vi "Beampointing_ajgEditObsolete.vi"() -> ()   [LabVIEW 2020]
uses:
  Shared/GUI_Template/GUI_master/tcp new data cluster.ctl
  <userlib>/_OpenG.lib/array/array.llb/Filter 1D Array with Scalar (String)__ogtk.vi
  <vilib>/Analysis/NI_AALBase.lvlib
  GUI_Beampointing_single_TRA/Ctrs/move.ctl
  Ctrs/beam detection.ctl
  <vilib>/vision/NI_Vision_Development_Module.lvlib
  General GUIs/Device GUIs/GUI_Cameras/Controls/Crosshair type def.ctl
  Ctrs/BP configuration.ctl
  <userlib>/_OpenG.lib/array/array.llb/Remove Duplicates from 1D Array (String)__ogtk.vi
  <vilib>/Utility/file.llb/Write To Spreadsheet File (string).vi
  <userlib>/_OpenG.lib/file/file.llb/Strip Path Extension - String__ogtk.vi
  <userlib>/_OpenG.lib/file/file.llb/File Exists - Scalar__ogtk.vi
  Shared/GUI_Template/GUI_master/tcp_new_data_event.ctl
panel:
  in  "active CCDs":i32(listbox)
  out "Prev State":string
  out "tcp data event 2":T1
  out "error out 3":errorcluster
  out "cam means":sgl[](array[numeric])
  in  "save path":path=path "W:/BP_DATA"
  out "particles":T2(array[cluster])
  out "millisecond timer value":u32
  out "motor refs 3":refnum<vi>[](array[refnum])
  in  "active man refs":cluster{"Ref X":refnum<vi>, "Ref Y":refnum<vi>}
  in  "#imgs avd so far":dbl
  out "Current State":string
  out "CCDs":string[](array[string])
  in  "GUIdevice 12":string
  in  "GUIdevice 11":string
  in  "GUIdevice 10":string
  in  "GUIdevice 9":string
  out "error out 2":errorcluster
  out "Names":string[](array[string])
  out "Box":T3(array[cluster])
  in  "Tab Cams":enum32{"Config ", "Main", "History", "Other"}(tab)=enum."Main"
  in  "Cameras and motors":T4(array[cluster]) {"Motor Alias Y" items=["M2 Y Axis", "M2 X Axis", "M4 Y Axis", "M4 X Axis", "M5 X Axis", "M5 Y Axis", "M1 Y Axis (mm)", "M1 X Axis (mm)", "Compression", "Grating 2&3", "Grating 1&4", "Clocking", "MIX", "F3M2 Horizontal", "F3M2 Vertical", "F3M3 Vertical", "F3M3 Horizontal", "F3M6 Horizontal", "F3M5 Horizontal", "F3M6 Vertical", "F3M5 Vertical", "HeatM5-X", "HeatM5-Y", "HeatM5-XY", "PlamsaLensHexapod", "HPD2 stage position", "HPD stage position", "M1-HPD X position", "M1-HPD Y position", "M2-HPD X position", "M2-HPD Y position", "HPDccd2 Stage position", "TargetX", "TargetY", "TargetZ", "IP", "PM4-X", "PM4-Y", "SDI_1x", "SDI_1y", "SDI_2x", "SDI_2y", "Comp-2BL-separation [mm]", "Comp-2BL-G1G4-angle [degree]", "Comp-2BL-G2G3-angle [degree]", "Comp-2BL-delay [mm]"]; "Motor Alias X" items=["M2 Y Axis", "M2 X Axis", "M4 Y Axis", "M4 X Axis", "M5 X Axis", "M5 Y Axis", "M1 Y Axis (mm)", "M1 X Axis (mm)", "Compression", "Grating 2&3", "Grating 1&4", "Clocking", "MIX", "F3M2 Horizontal", "F3M2 Vertical", "F3M3 Vertical", "F3M3 Horizontal", "F3M6 Horizontal", "F3M5 Horizontal", "F3M6 Vertical", "F3M5 Vertical", "HeatM5-X", "HeatM5-Y", "HeatM5-XY", "PlamsaLensHexapod", "HPD2 stage position", "HPD stage position", "M1-HPD X position", "M1-HPD Y position", "M2-HPD X position", "M2-HPD Y position", "HPDccd2 Stage position", "TargetX", "TargetY", "TargetZ", "IP", "PM4-X", "PM4-Y", "SDI_1x", "SDI_1y", "SDI_2x", "SDI_2y", "Comp-2BL-separation [mm]", "Comp-2BL-G1G4-angle [degree]", "Comp-2BL-G2G3-angle [degree]", "Comp-2BL-delay [mm]"]}
  out "Status":cluster{i32, i32, "Centroid X":dbl[][]}(graph)
  in  "tdms root":path=path "c:/BP_DATAsd"
  out "get pos time":u32
  out "config path":string
  in  "Exposure:12":dbl=0.095 min=0.0001 max=1.0 format="%#_6f"
  in  "Triggerdelay::12":dbl=0.003 min=0.0 max=0.09 format="%#_6f"
  in  "Exposure::11":dbl=0.095 min=0.0001 max=1.0 format="%#_6f"
  in  "Triggerdelay::11":dbl=0.003 min=0.0 max=0.09 format="%#_6f"
  in  "Exposure::10":dbl=0.095 min=0.0001 max=1.0 format="%#_6f"
  in  "Triggerdelay::10":dbl=0.003 min=0.0 max=0.09 format="%#_6f"
  in  "Exposure::9":dbl=0.095 min=0.0001 max=1.0 format="%#_6f"
  in  "Triggerdelay::9":dbl=0.003 min=0.0 max=0.09 format="%#_6f"
  in  "Trigger::9":bool
  in  "Trigger::10":bool caption="Trigger:10"
  in  "Trigger::11":bool
  in  "Trigger::12":bool
  in  "Target.Y::9":dbl=45.0 caption="T9y" min=0.0 max=2000.0 format="%#_6f"
  in  "Target.X::9":dbl=47.0 caption="Tx9" min=0.0 max=2000.0 format="%#_6f"
  in  "Target.Y::10":dbl=45.0 caption="T10y" min=0.0 max=2000.0 format="%#_6f"
  in  "Target.X::10":dbl=47.0 caption="T10x" min=0.0 max=2000.0 format="%#_6f"
  in  "Target.Y::11":dbl=45.0 caption="T11y" min=0.0 max=2000.0 format="%#_6f"
  in  "Target.X::11":dbl=47.0 caption="T11x" min=0.0 max=2000.0 format="%#_6f"
  in  "Target.Y::12":dbl=45.0 caption="T12y" min=0.0 max=2000.0 format="%#_6f"
  in  "Target.X::12":dbl=47.0 caption="T12x" min=0.0 max=2000.0 format="%#_6f"
  in  "Exposure::8":dbl=0.095 min=0.0001 max=1.0 format="%#_6f"
  in  "Triggerdelay::8":dbl=0.003 min=0.0 max=0.09 format="%#_6f"
  in  "Trigger::8":bool
  in  "Target.Y::8":dbl=45.0 caption="T8y" min=0.0 max=2000.0 format="%#_6f"
  in  "Target.X::8":dbl=47.0 caption="T8x" min=0.0 max=2000.0 format="%#_6f"
  in  "Target.Y::7":dbl=45.0 caption="T7x" min=0.0 max=2000.0 format="%#_6f"
  in  "Target.X::7":dbl=47.0 caption="T7y" min=0.0 max=2000.0 format="%#_6f"
  in  "Target.Y::6":dbl=45.0 caption="T6y" min=0.0 max=2000.0 format="%#_6f"
  in  "Target.X::6":dbl=47.0 caption="T6x" min=0.0 max=2000.0 format="%#_6f"
  in  "Target.Y::5":dbl=45.0 caption="T5y" min=0.0 max=2000.0 format="%#_6f"
  in  "Target.X::5":dbl=47.0 caption="T5x" min=0.0 max=2000.0 format="%#_6f"
  in  "Target.Y::4":dbl=45.0 caption="T4y" min=0.0 max=2000.0 format="%#_6f"
  in  "Target.X::4":dbl=47.0 caption="T4x" min=0.0 max=2000.0 format="%#_6f"
  in  "Target.Y::3":dbl=163.0 caption="T3y" min=0.0 max=2000.0 format="%#_6f"
  in  "Target.X::3":dbl=152.0 caption="T3x" min=0.0 max=2000.0 format="%#_6f"
  in  "Target.Y::2":dbl=74.0 caption="T2y" min=0.0 max=2000.0 format="%#_6f"
  in  "Target.X::2":dbl=75.0 caption="T2x" min=0.0 max=2000.0 format="%#_6f"
  in  "Target.Y::1":dbl=61.0 caption="T1y" min=0.0 max=2000.0 format="%#_6f"
  in  "Target.X::1":dbl=77.0 caption="T1x" min=0.0 max=2000.0 format="%#_6f"
  in  "Exposure::7":dbl=0.095 min=3.8e-05 max=1.0 format="%#_6f"
  in  "Triggerdelay::7":dbl=0.003 min=0.0 max=0.09 format="%#_6f"
  in  "Trigger::7":bool
  in  "Exposure::6":dbl=0.095 min=3.8e-05 max=1.0 format="%#_6f"
  in  "Triggerdelay::6":dbl=0.003 min=0.0 max=0.09 format="%#_6f"
  in  "Trigger::6":bool
  in  "Exposure::5":dbl=0.095 min=3.8e-05 max=1.0 format="%#_6f"
  in  "Triggerdelay::5":dbl=0.003 min=0.0 max=0.09 format="%#_6f"
  in  "Trigger::5":bool
  in  "Exposure::4":dbl=0.095 min=3.8e-05 max=1.0 format="%#_6f"
  in  "Triggerdelay::4":dbl=0.003 min=0.0 max=0.09 format="%#_6f"
  in  "Trigger::4":bool
  in  "Exposure::3":dbl=0.095 min=3.8e-05 max=1.0 format="%#_6f"
  in  "Triggerdelay::3":dbl=0.003 min=0.0 max=0.09 format="%#_6f"
  in  "Trigger::3":bool
  in  "Exposure::2":dbl=0.095 min=3.8e-05 max=1.0 format="%#_6f"
  in  "Triggerdelay::2":dbl=0.003 min=0.0 max=0.09 format="%#_6f"
  in  "Trigger::2":bool
  out "image::1":T5(plugin-control) caption="CAM-2BL-GHOST"
  out "image::2":T5(plugin-control) caption="CAM-2BL-F3M7"
  out "image::3":T5(plugin-control)
  out "image::4":T5(plugin-control)
  out "image::5":T5(plugin-control)
  out "image::6":T5(plugin-control)
  out "image::7":T5(plugin-control)
  out "image::8":T5(plugin-control)
  in  "Exposure::1":dbl=0.095 min=3.8e-05 max=1.0 format="%#_6f"
  in  "Triggerdelay::1":dbl=0.003 min=0.0 max=0.09 format="%#_6f"
  in  "Trigger::1":bool
  in  "UDP error message":string
  out "required Y":bool[](array[boolean])
  out "required X":bool[](array[boolean])
  out "detected":bool[](array[boolean])
  out "name array":string[](array[string])
  out "image::9":T5(plugin-control)
  out "image::10":T5(plugin-control)
  out "image::11":T5(plugin-control)
  out "image::12":T5(plugin-control)
  out "speedmode X":bool[](array[boolean])
  out "speedmode Y":bool[](array[boolean])
  out "CCD 9":cluster{timestamp[], dbl[]}[](graph)
  out "CCD 10":cluster{timestamp[], dbl[]}[](graph)
  out "CCD 11":cluster{timestamp[], dbl[]}[](graph)
  out "CCD 12":cluster{timestamp[], dbl[]}[](graph)
  out "CCD 5":cluster{timestamp[], dbl[]}[](graph)
  out "CCD 6":cluster{timestamp[], dbl[]}[](graph)
  out "CCD 7":cluster{timestamp[], dbl[]}[](graph)
  out "CCD 8":cluster{timestamp[], dbl[]}[](graph)
  out "CCD 2":cluster{timestamp[], dbl[]}[](graph)
  out "CCD 1":cluster{timestamp[], dbl[]}[](graph)
  out "CCD 3":cluster{timestamp[], dbl[]}[](graph)
  out "CCD 4":cluster{timestamp[], dbl[]}[](graph)
  in  "History Size":i32=500
  out "History Index":i32
  out "Moving X":string
  out "Moving Y":string
  in  "Feedback Global":bool
  in  "GUIdevice 8":string
  in  "Tab Control":T6(tab)
  in  "alarms":bool
  in  "new tdms":bool
  in  "Save Stats":bool
  in  "Save Config":bool
  in  "Load Config":bool
  in  "update speed [ms]":i32=2000
  in  "img to avg":i32=6 min=3 max=200
  in  "Reset History":bool
  in  "autodetect":bool
  in  "Detection Rate":dbl=0.9 min=0.001 max=1.0
  in  "Center":bool
  in  "Align":bool
  in  "Speedmode":dbl=5.0 min=1.0 max=20.0
  in  "device ini":bool
  in  "average centroid":bool
  in  "beam detection para":T7={"Filter"=1, "Filter Para"={"X Size"=5, "Y Size"=5, "% Tolerance"=1}, "detection method"=4, "smal para"=[{"Measurement Parameter"=35, "Range Lower Value"=0.0, "Range Upper Value"=500.0, "Range"=FALSE, "Measurement Type"=FALSE}], "Remove small Objects"=TRUE, "Restrict to round Objects"=FALSE} {"smal para"."Measurement Parameter" items=["Center of Mass X", "Center of Mass Y", "First Pixel X", "First Pixel Y", "Bounding Rect Left", "Bounding Rect Top", "Bounding Rect Right", "Bounding Rect Bottom", "Max Feret Diameter Start X", "Max Feret Diameter Start Y", "Max Feret Diameter End X", "Max Feret Diameter End Y", "Max Horiz. Segment Length Left", "Max Horiz. Segment Length Right", "Max Horiz. Segment Length Row", "-", "Bounding Rect Width", "Bounding Rect Height", "Bounding Rect Diagonal", "Perimeter", "Convex Hull Perimeter", "Holes' Perimeter", "Max Feret Diameter", "Equivalent Ellipse Major Axis", "Equivalent Ellipse Minor Axis", "Equivalent Ellipse Minor Axis (Feret)", "Equivalent Rect Long Side", "Equivalent Rect Short Side", "Equivalent Rect Diagonal", "Equivalent Rect Short Side (Feret)", "Average Horiz. Segment Length", "Average Vert. Segment Length", "Hydraulic Radius", "Waddel Disk Diameter", "-", "Area", "Holes' Area", "Particle & Holes' Area", "Convex Hull Area", "Image Area", "-", "Number of Holes", "Number of Horiz. Segments", "Number of Vert. Segments", "-", "Orientation", "Max Feret Diameter Orientation", "-", "% Area/Image Area", "% Area/(Particle & Holes' Area)", "Ratio of Equivalent Ellipse Axes", "Ratio of Equivalent Rect Sides", "-", "Elongation Factor", "Compactness Factor", "Heywood Circularity Factor", "Type Factor", "-", "Sum X", "Sum Y", "Sum XX", "Sum XY", "Sum YY", "Sum XXX", "Sum XXY", "Sum XYY", "Sum YYY", "-", "Moment of Inertia XX", "Moment of Inertia XY", "Moment of Inertia YY", "Moment of Inertia XXX", "Moment of Inertia XXY", "Moment of Inertia XYY", "Moment of Inertia YYY", "Norm. Moment of Inertia XX", "Norm. Moment of Inertia XY", "Norm. Moment of Inertia YY", "Norm. Moment of Inertia XXX", "Norm. Moment of Inertia XXY", "Norm. Moment of Inertia XYY", "Norm. Moment of Inertia YYY", "Hu Moment 1", "Hu Moment 2", "Hu Moment 3", "Hu Moment 4", "Hu Moment 5", "Hu Moment 6", "Hu Moment 7"]; "smal para"."Range Lower Value" format="%.2f"; "smal para"."Range Upper Value" format="%.2f"; "detection method" items=["clustering", "entropy", "metric", "moments", "inter-class variance"]; "Filter" items=["No Filter", "Median Filter", "Low Pass Filter"]}
  in  "move config":T9={"Tolerance [%]"=0.1, "Stepsize"=0.0001, "Invert Axis"=TRUE, "Invert Direction X"=FALSE, "Invert Direction Y"=TRUE, "enable feedback"=FALSE, "Set Centriod Target"=FALSE}
  in  "Position 2":dbl=0.001 caption="Stepsize" min=0.0 max=999999.0 format="%_6f"
  in  "Position 1":dbl=0.001 caption="Stepsize" min=0.0 max=999999.0 format="%_6f"
  in  "Right":bool caption="RelativeMove.Axis 1.CCW::1"
  in  "Left":bool caption="RelativeMove.Axis 1.CW::1"
  in  "Down":bool caption="RelativeMove.Axis. 2.CCW::1"
  in  "Up":bool caption="RelativeMove.Axis 2.CW::1"
  in  "StepSize":dbl=1.0 caption="Stepsize" min=0.0 max=1.0 step=0.001 format="%#_6p"
  in  "Time":timestamp[][](array[timestamp])
  in  "Offset X":dbl[][](array[numeric])
  in  "Mean Centroid X":dbl[][](array[numeric])
  in  "GUIdevice 7":string
  in  "GUIdevice 6":string
  in  "GUIdevice 5":string
  in  "GUIdevice 4":string
  in  "GUIdevice 3":string="TargetCam10Hz_Diode"
  in  "GUIdevice 2":string="StagingM1Far"
  in  "insert tag":bool=TRUE
  in  "stop":bool
  in  "GUIdevice 1":string="StagingM1Near"
  out "error IO 2":errorcluster
  # "Motor axes must have aliases"
  # "max"
  # "invert axis no longer used"
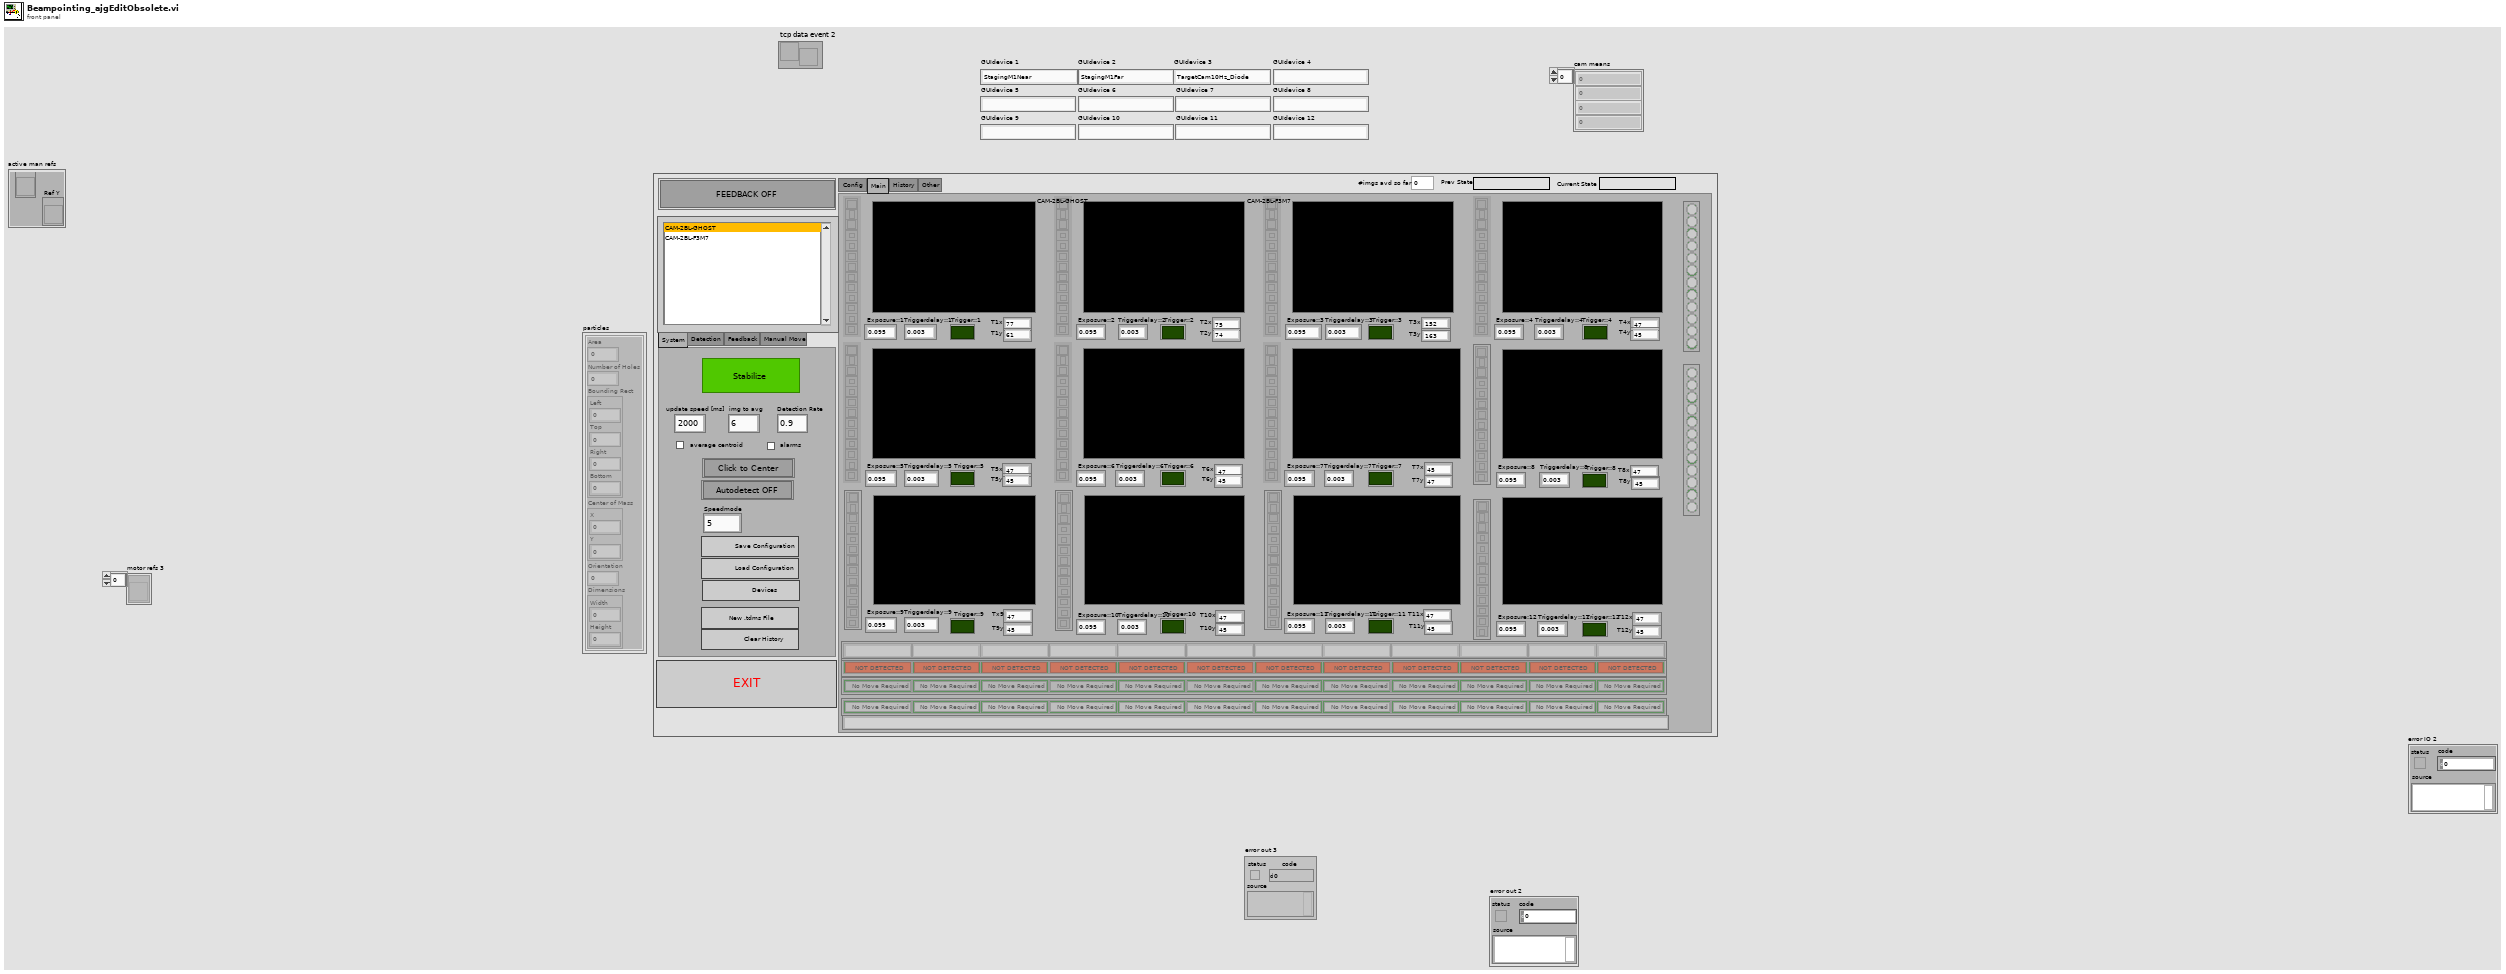
[diagram p1: front panel]
types:
  T1 = typedef "tcp_new_data_event.ctl" = refnum<user-event>
  T2 = cluster{"Area":dbl, "Number of Holes":dbl, "Bounding Rect":cluster{"Left":dbl, "Top":dbl, "Right":dbl, "Bottom":dbl}, "Center of Mass":cluster{"X":dbl, "Y":dbl}, "Orientation":dbl, "Dimensions":cluster{"Width":dbl, "Height":dbl}}[]
  T3 = cluster{"Left":dbl, "Top":dbl, "Right":dbl, "Bottom":dbl}[]
  T4 = cluster{"Camera":string, "Motor Alias X":u16, "Motor Alias Y":u16}[]
  T5 = typedef "IMAQ Image.ctl" = refnum<image>
  T6 = enum32{"System", "Detection", "Feedback", "Manual Move"}
  T7 = typedef "beam detection.ctl" = cluster{"Filter":u16, "Filter Para":cluster{"X Size":i32, "Y Size":i32, "% Tolerance":i32}, "detection method":i32, "smal para":cluster{"Measurement Parameter":T8, "Range Lower Value":dbl, "Range Upper Value":dbl, "Range":bool, "Measurement Type":bool}[], "Remove small Objects":bool, "Restrict to round Objects":bool}
  T8 = typedef "Particle Parameters" = i32
  T9 = typedef "move.ctl" = cluster{"Tolerance [%]":dbl, "Stepsize":dbl, "Invert Axis":bool, "Invert Direction X":bool, "Invert Direction Y":bool, "enable feedback":bool, "Set Centriod Target":bool}
  T10 = cluster{"Target.X::1":refnum<vi>, "Target.Y::1":refnum<vi>}
  T11 = cluster{"Target.X::2":refnum<vi>, "Target.Y::2":refnum<vi>}
  T12 = cluster{"Target.X::3":refnum<vi>, "Target.Y::3":refnum<vi>}
  T13 = cluster{"Target.X::4":refnum<vi>, "Target.Y::4":refnum<vi>}
  T14 = cluster{"Target.X::5":refnum<vi>, "Target.Y::5":refnum<vi>}
  T15 = cluster{"Target.X::6":refnum<vi>, "Target.Y::6":refnum<vi>}
  T16 = cluster{"Target.X::7":refnum<vi>, "Target.Y::7":refnum<vi>}
  T17 = cluster{"Target.X::8":refnum<vi>, "Target.Y::8":refnum<vi>}
  T18 = cluster{"Target.X::12":refnum<vi>, "Target.Y::12":refnum<vi>}
  T19 = cluster{"Target.X::9":refnum<vi>, "Target.Y::9":refnum<vi>}
  T20 = cluster{"Target.X::10":refnum<vi>, "Target.Y::10":refnum<vi>}
  T21 = cluster{"Target.X::11":refnum<vi>, "Target.Y::11":refnum<vi>}
  T22 = cluster{"Target.X::12":refnum<vi>, "Target.Y::12":refnum<vi>}[]
  T23 = enum32{"invalid app kind", "Development System", "Run Time System", "Student Edition", "Embedded LabVIEW", "Evaluation", "Custom"}
  T24 = enum32{"Invalid", "Standard", "Closed", "Hidden", "Minimized", "Maximized"}
  T25 = typedef "tcp new data cluster.ctl" = cluster{"EventEnum":enum16{"new data", "connection status update"}, "Device name":string}
  T26 = enum16{"open", "replace", "create", "open or create", "replace or create", "replace or create with confirmation"}
  T27 = enum8{"Enabled", "Disabled", "Disabled and Grayed Out"}
  T28 = enum16{"open", "open or create", "create or replace", "create", "open (read-only)"}
  T29 = cluster{"Left":dbl, "Top":dbl, "Right":dbl, "Bottom":dbl}
  T30 = typedef "move.ctl" = cluster{"Tolerance [pix]":dbl, "Stepsize":dbl, "Invert Direction X":bool, "Invert Direction Y":bool, "enable feedback":bool, "Set Centriod Target":bool}
  T31 = cluster{"Core":cluster{"Current VI Reference":refnum<vi>, "Close Panel on Exit?":bool}, "detection para":T7[], "thresholds":cluster{"Lower value":sgl, "Upper value":sgl}[], "Centroid X":dbl[][], "Centroid Y":dbl[][], "img to avg":i32, "Mean Centroid X":dbl[][], "Mean Centroid Y":dbl[][], "Offset X":dbl[][], "Offset Y":dbl[][], "Offset X stats ":dbl[][], "Offset Y stats ":dbl[][], "Size":dbl[][], "Mean Size":dbl[][], "Time":timestamp[][], "move properties":T30[], "active axis refs 2":cluster{"Ref X":refnum<vi>, "Ref Y":refnum<vi>}[], "active ccd":i32, "Feedback global":bool, "Motor X":dbl[][], "Motor Y":dbl[][], "active cams":string[], "tdms ref":refnum<k34>, "active man refs":cluster{"Ref X":refnum<vi>, "Ref Y":refnum<vi>}, "detected":bool[], "speedmode X":bool[], "speedmode Y":bool[], "steps speed X":dbl[], "steps speed Y":dbl[], "Supergui":cluster{"STOP queue":refnum<queue>, "SuperGUI ref":refnum<vi>}, "dev var alias arrays":cluster{"dev variable alias":string[][], "dev variable alias Motors X":string[][], "dev variable alias Motors Y":string[][]}, "Motor positions":cluster{"Positions x":dbl[], "Positions y":dbl[]}}
  T32 = cluster{"Positions x":dbl[], "Positions y":dbl[]}
  T33 = cluster{"dev variable alias":string[][], "dev variable alias Motors X":string[][], "dev variable alias Motors Y":string[][]}
  T34 = cluster{"Ref X":refnum<vi>, "Ref Y":refnum<vi>}[]
  T35 = cluster{"STOP queue":refnum<queue>, "SuperGUI ref":refnum<vi>}
  T36 = cluster{"Current VI Reference":refnum<vi>, "Close Panel on Exit?":bool}
  T37 = cluster{"Camera":string, "Motor Alias X":u16, "Motor Alias Y":u16}
  T38 = typedef "BP configuration.ctl" = cluster{"Camera names":string[], "Motor aliases x":string[], "Motor aliases y":string[], "detection para":T7[], "thresholds":cluster{"Lower value":sgl, "Upper value":sgl}[], "move properties":T30[]}
  T39 = typedef "Image Type" = u32
  T40 = cluster{"appended array":timestamp[], "appended array":dbl[]}
  T41 = cluster{"appended array":timestamp[], "appended array":dbl[]}[]
  T42 = typedef "Crosshair type def.ctl" = cluster{"Draw":bool, "Target":cluster{"x":dbl, "y":dbl}, "Size":cluster{"x":dbl, "y":dbl}, "Angle":dbl, "Color":u32, "Thickness":u8, "CrosshairLabel":string}
  T43 = cluster{"Left":i32, "Top":i32, "Right":i32, "Bottom":i32}
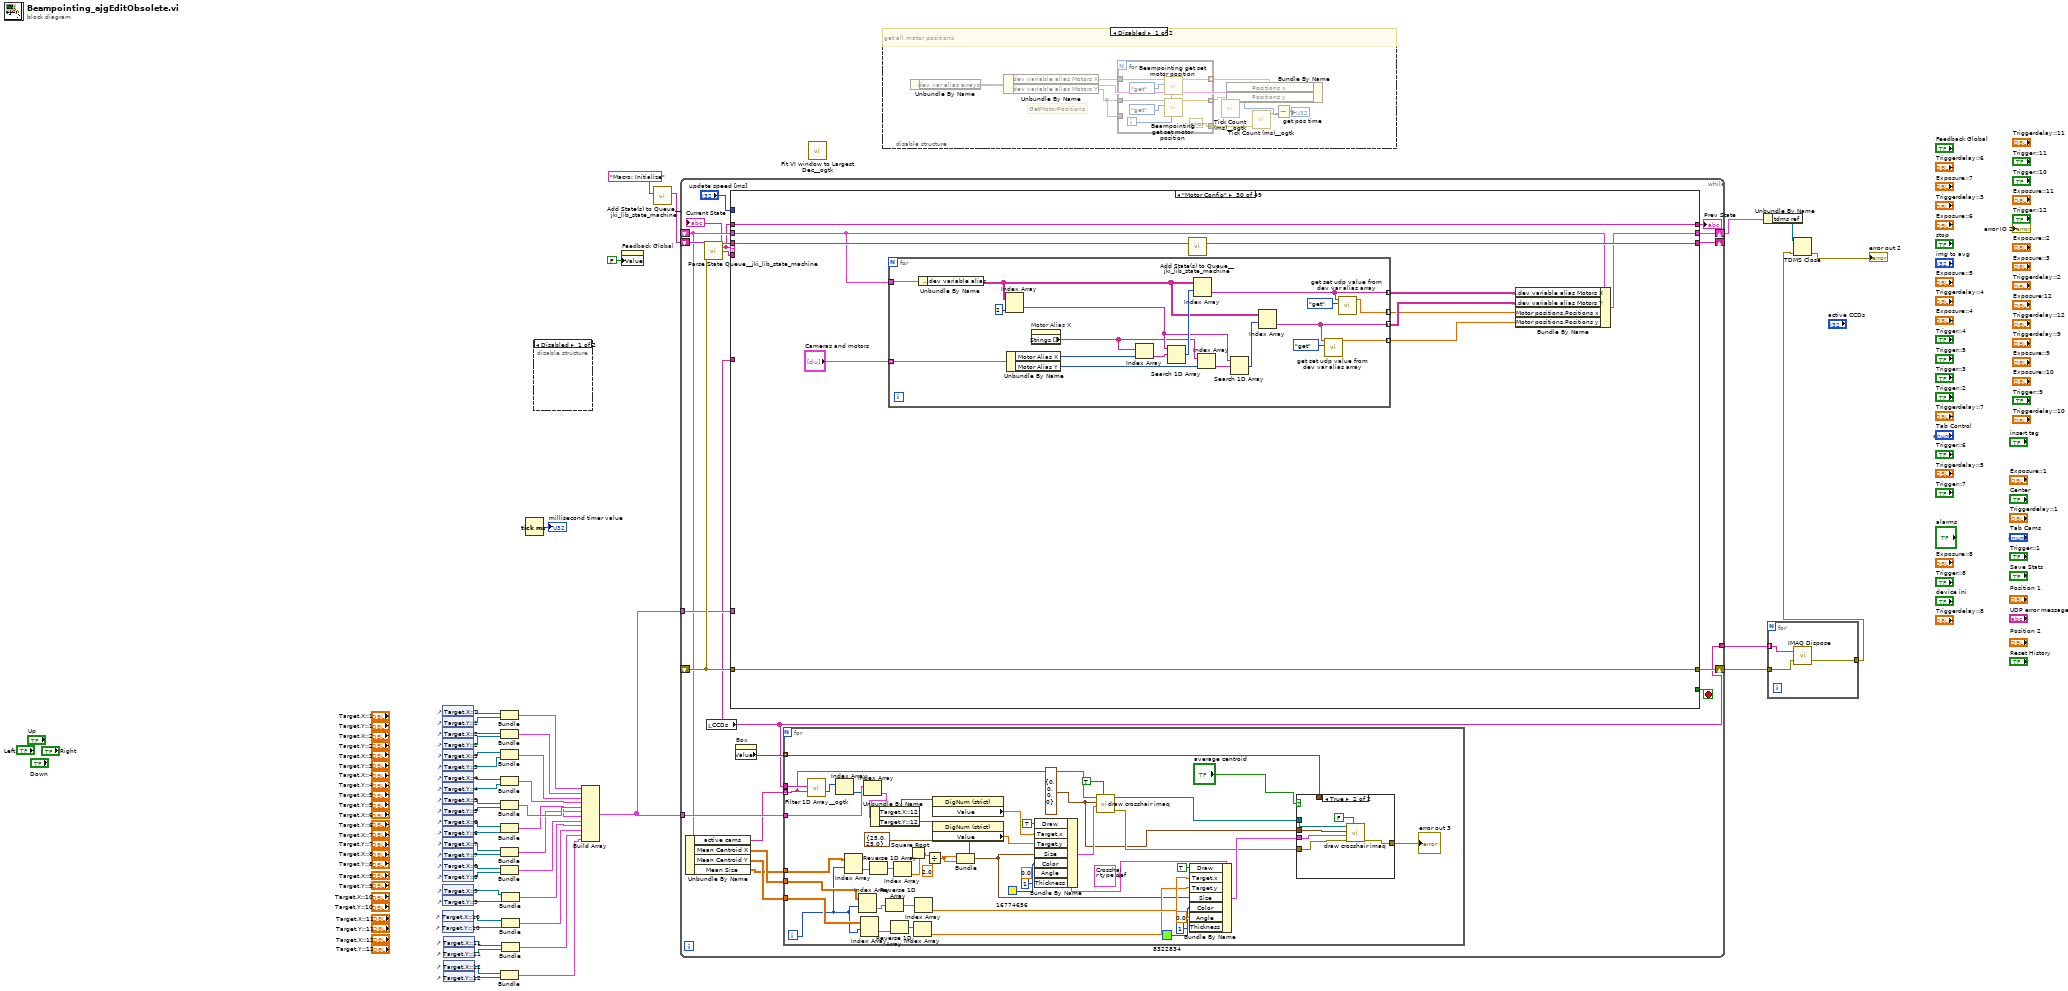
[diagram p0: block diagram]
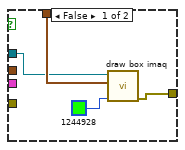
[diagram p4: hidden frame]
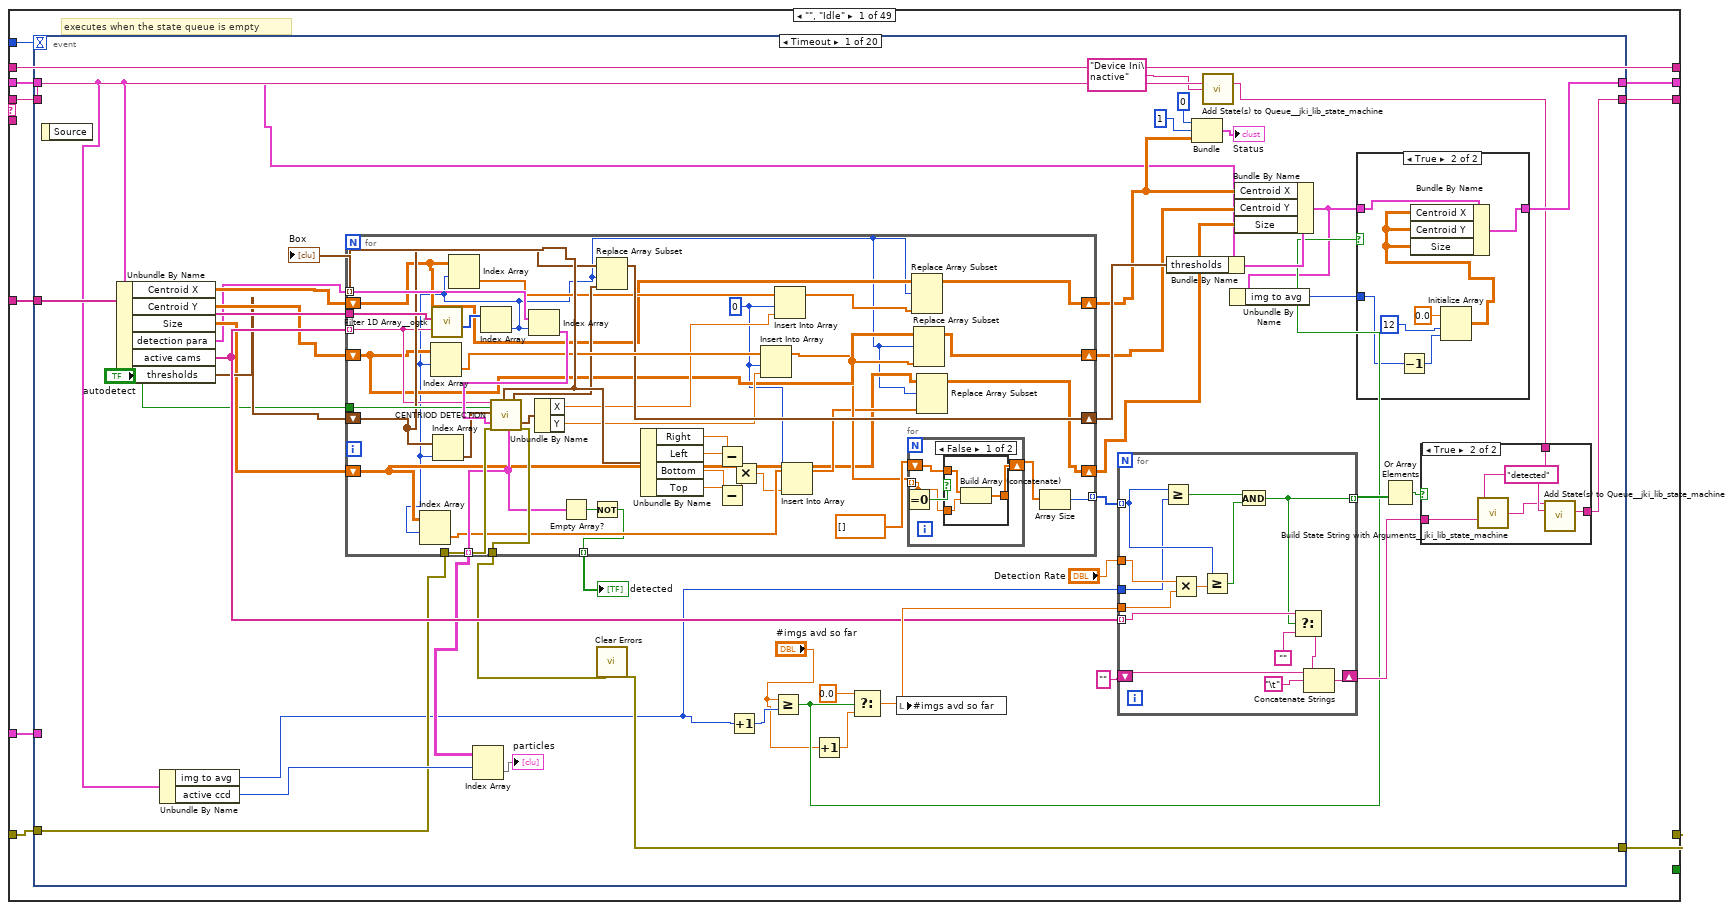
[diagram p5: hidden frame]
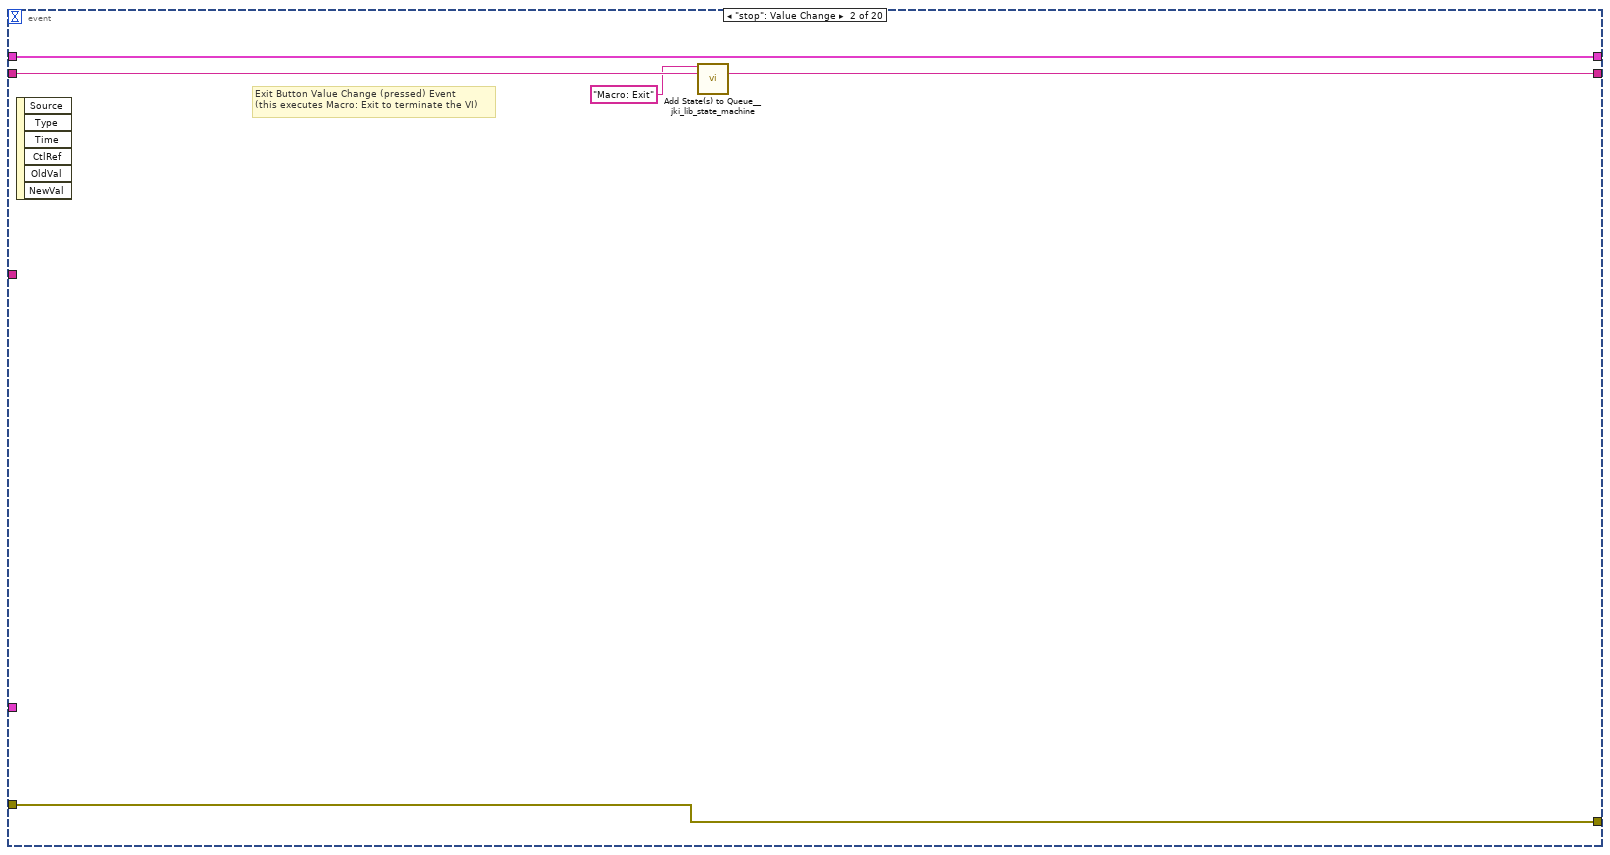
[diagram p9: hidden frame]
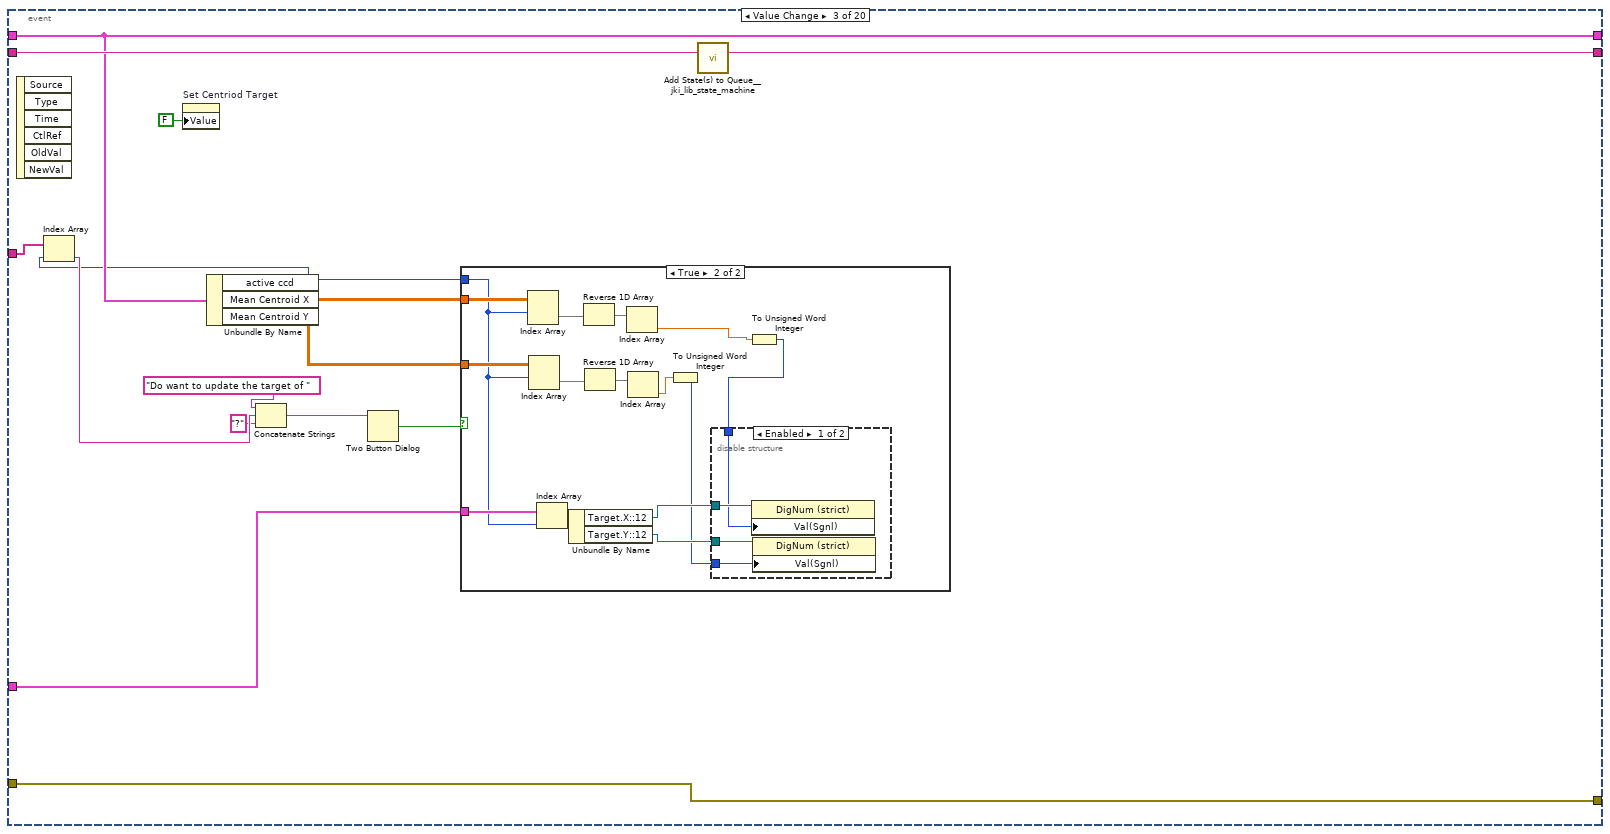
[diagram p10: hidden frame]
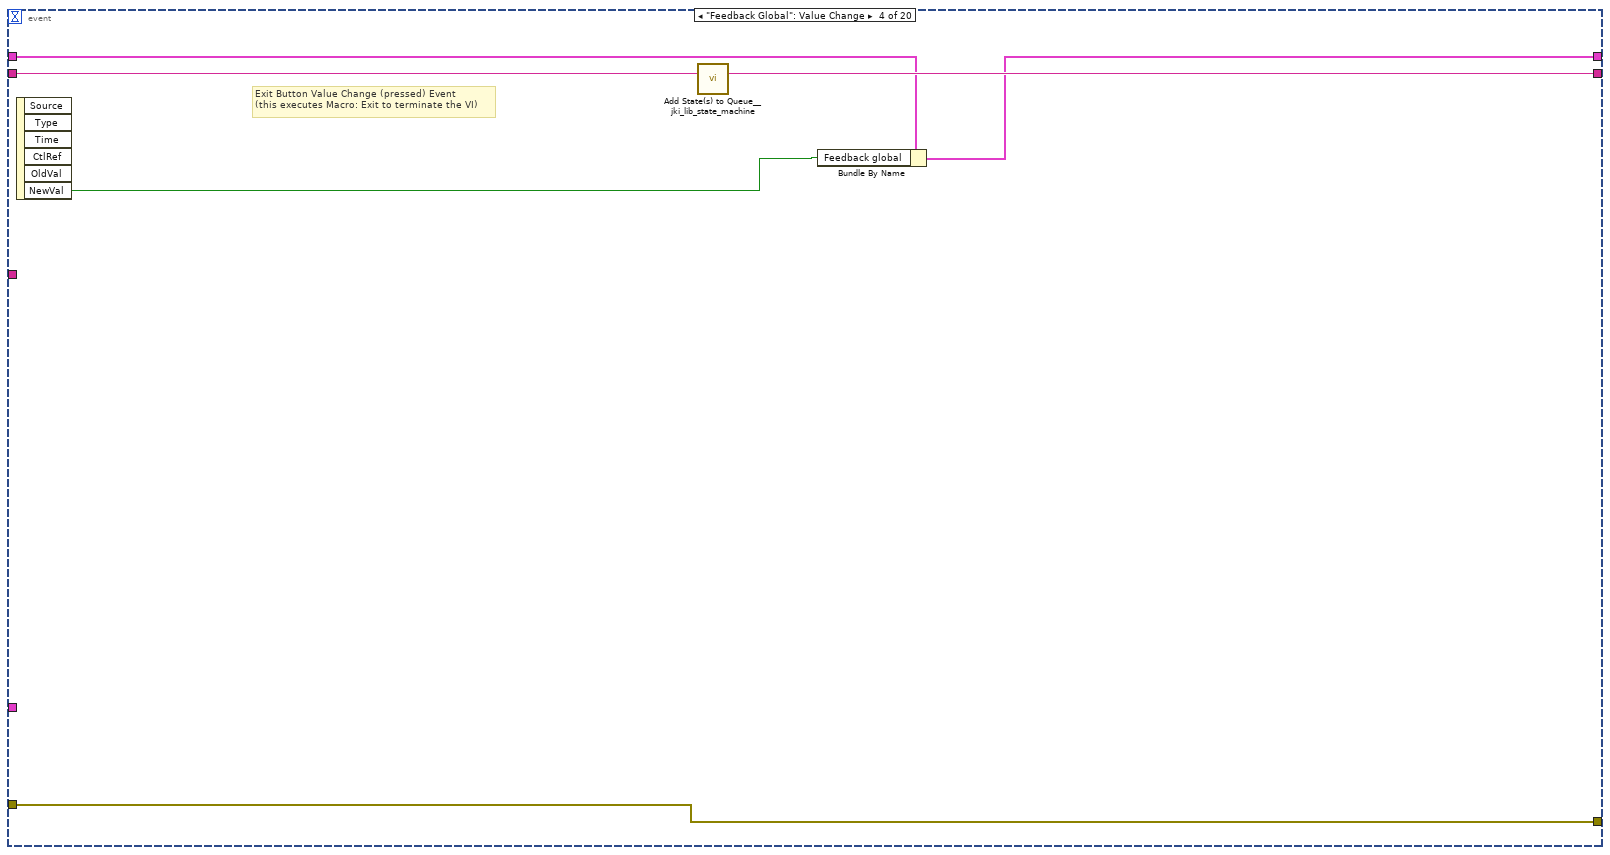
[diagram p13: hidden frame]
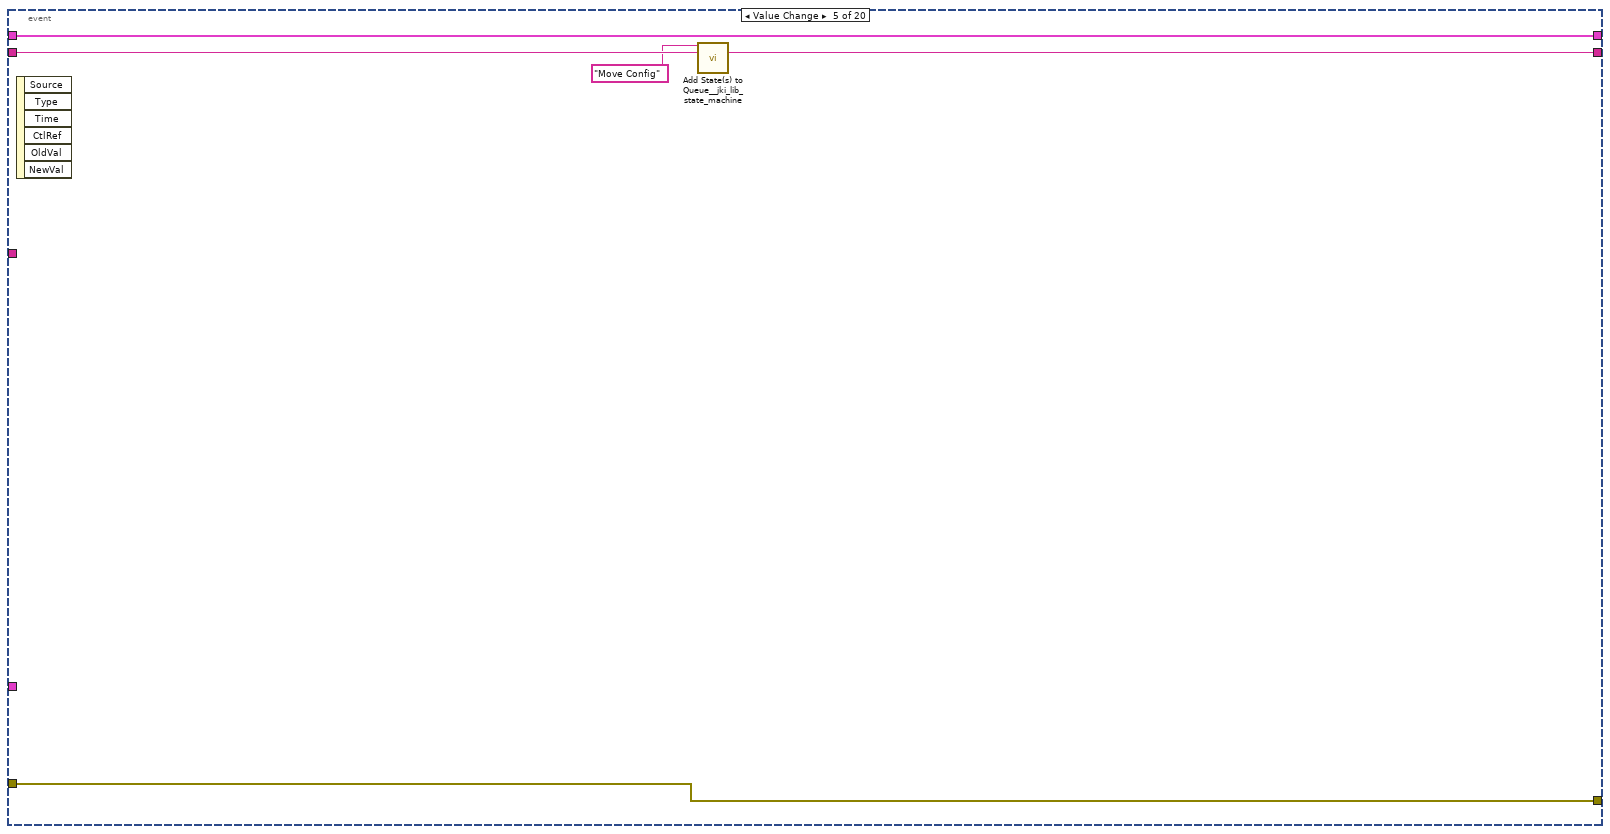
[diagram p14: hidden frame]
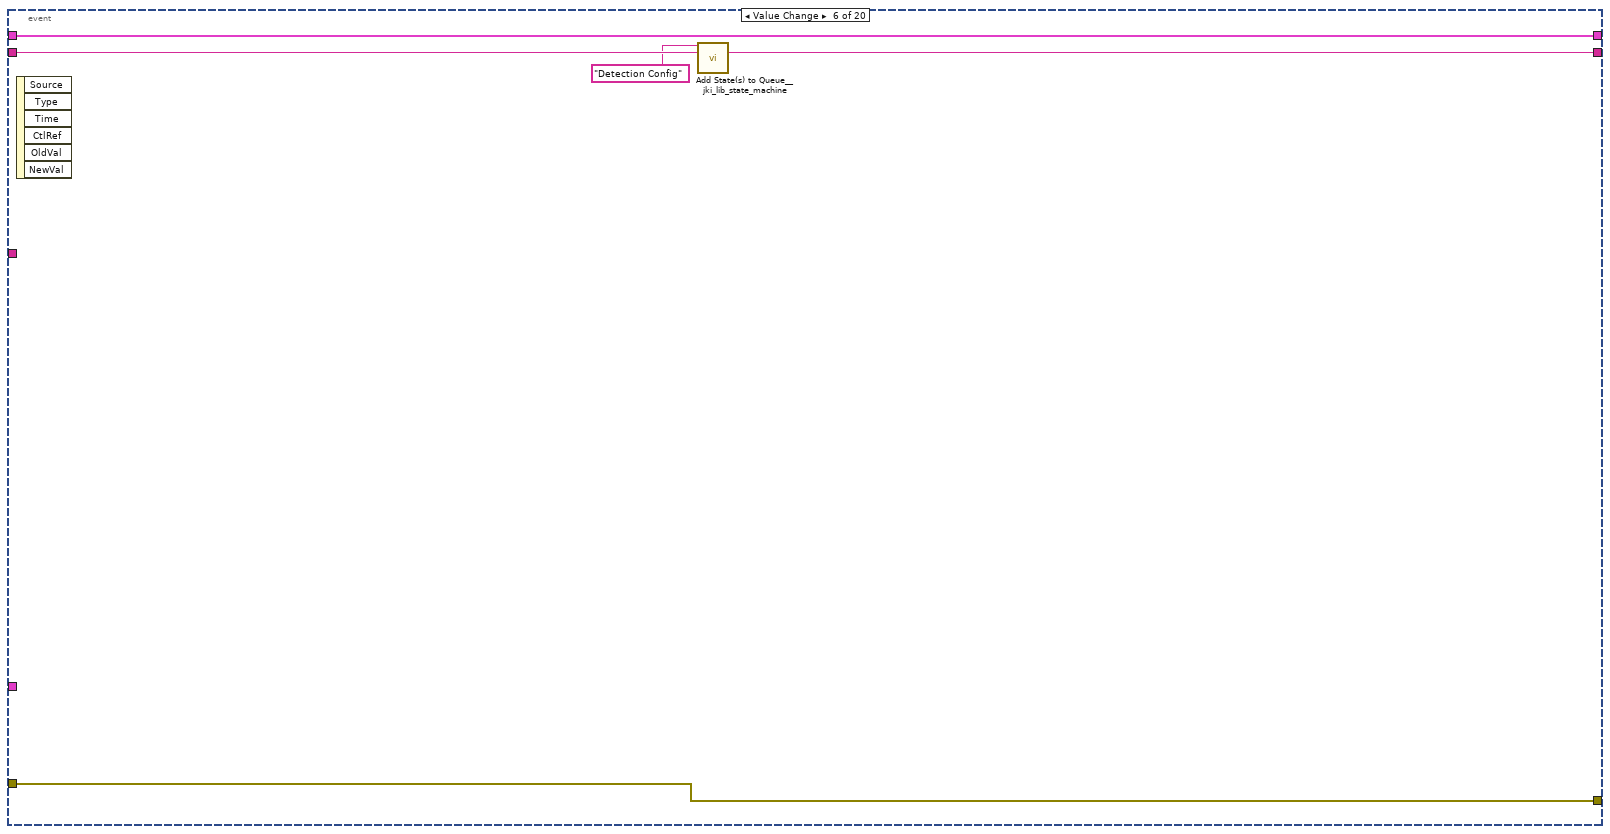
[diagram p15: hidden frame]
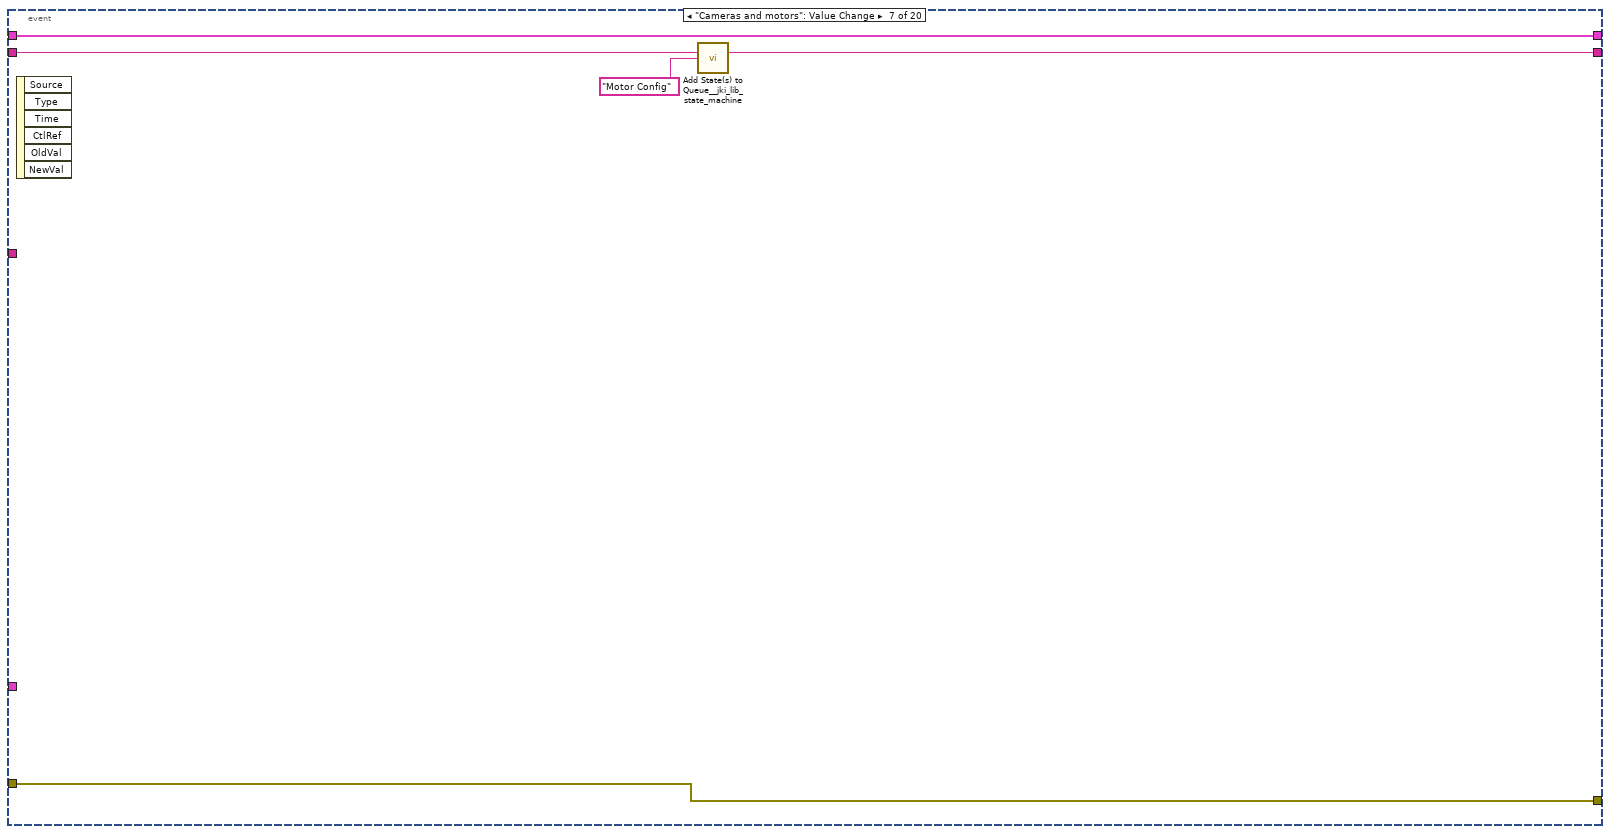
[diagram p16: hidden frame]
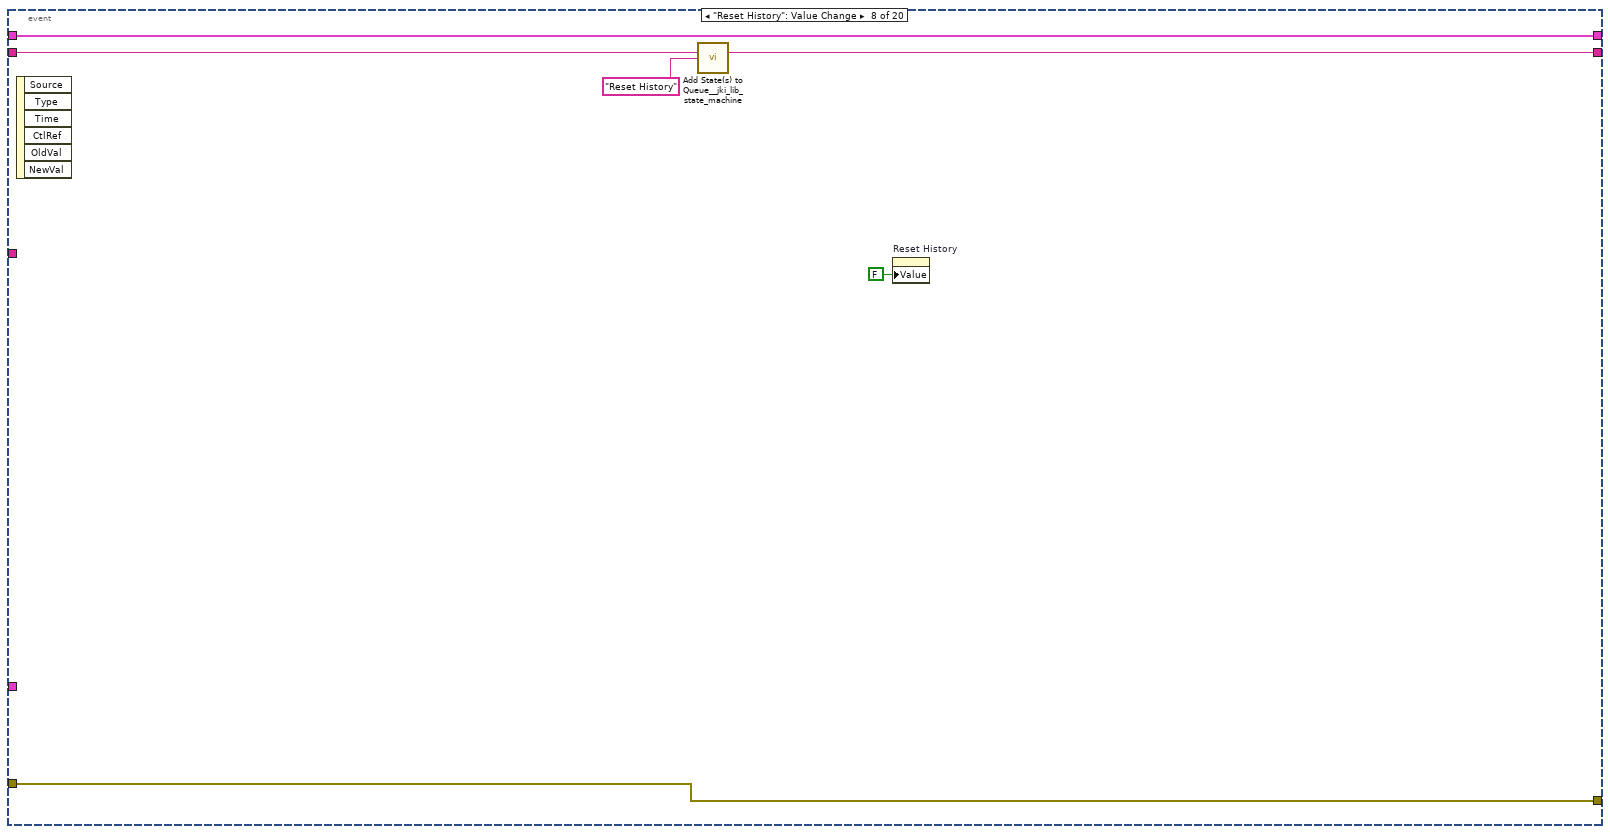
[diagram p17: hidden frame]
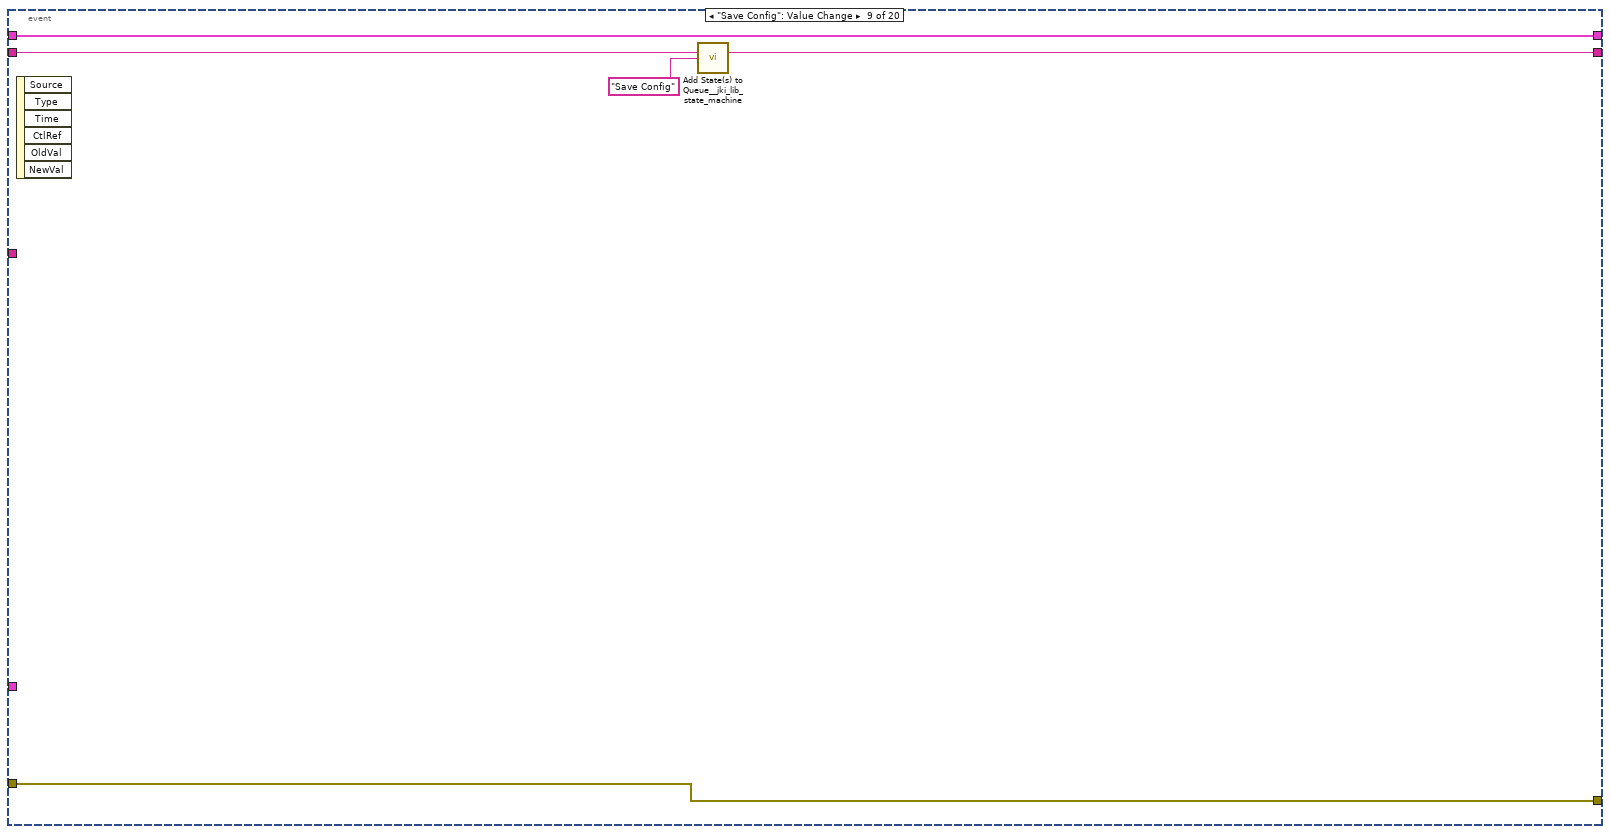
[diagram p18: hidden frame]
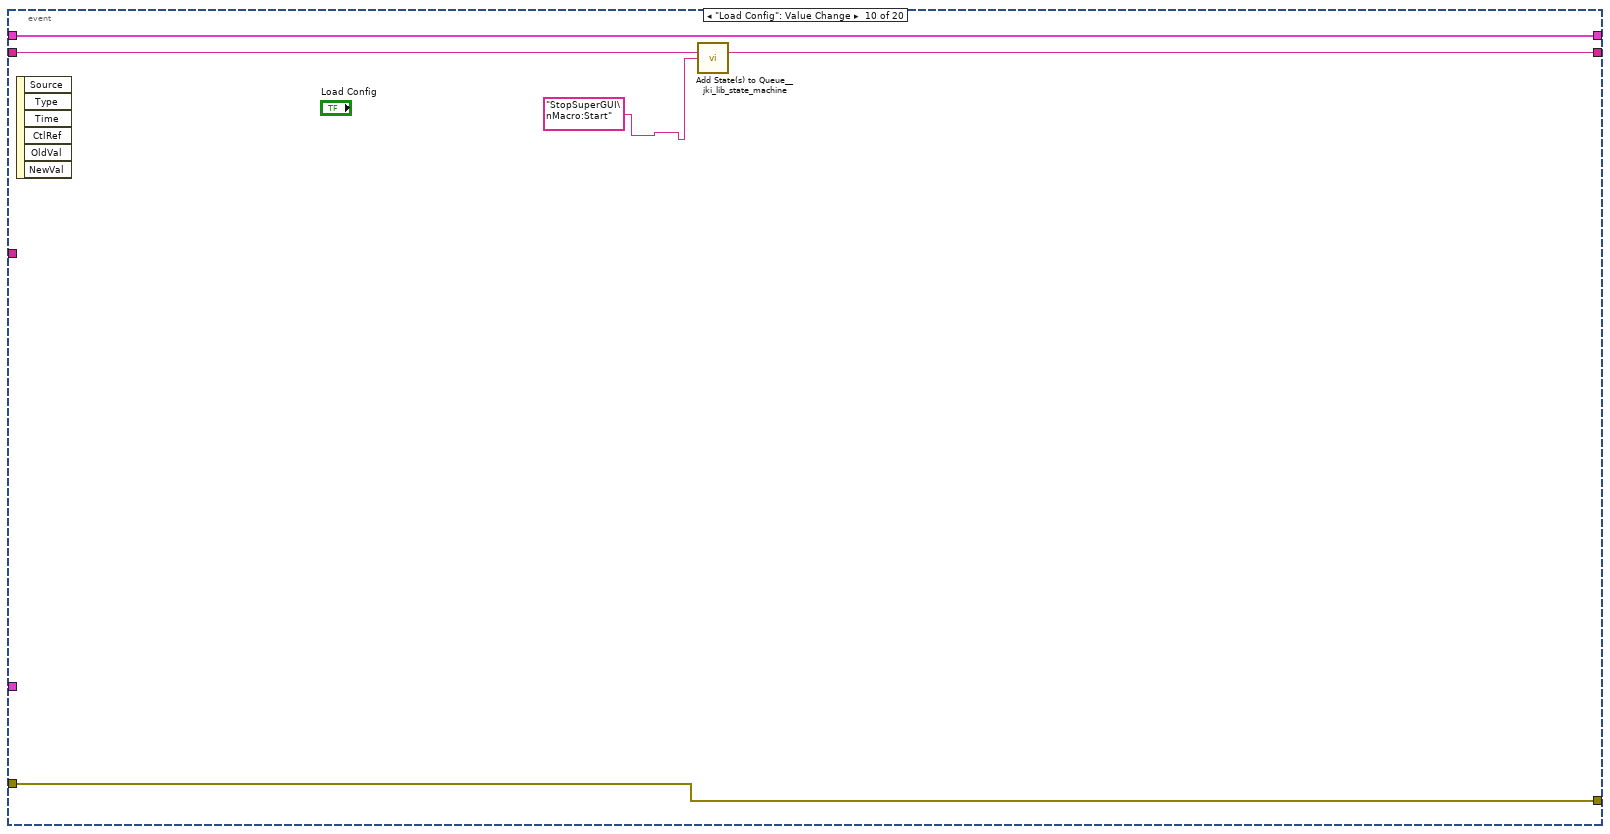
[diagram p19: hidden frame]
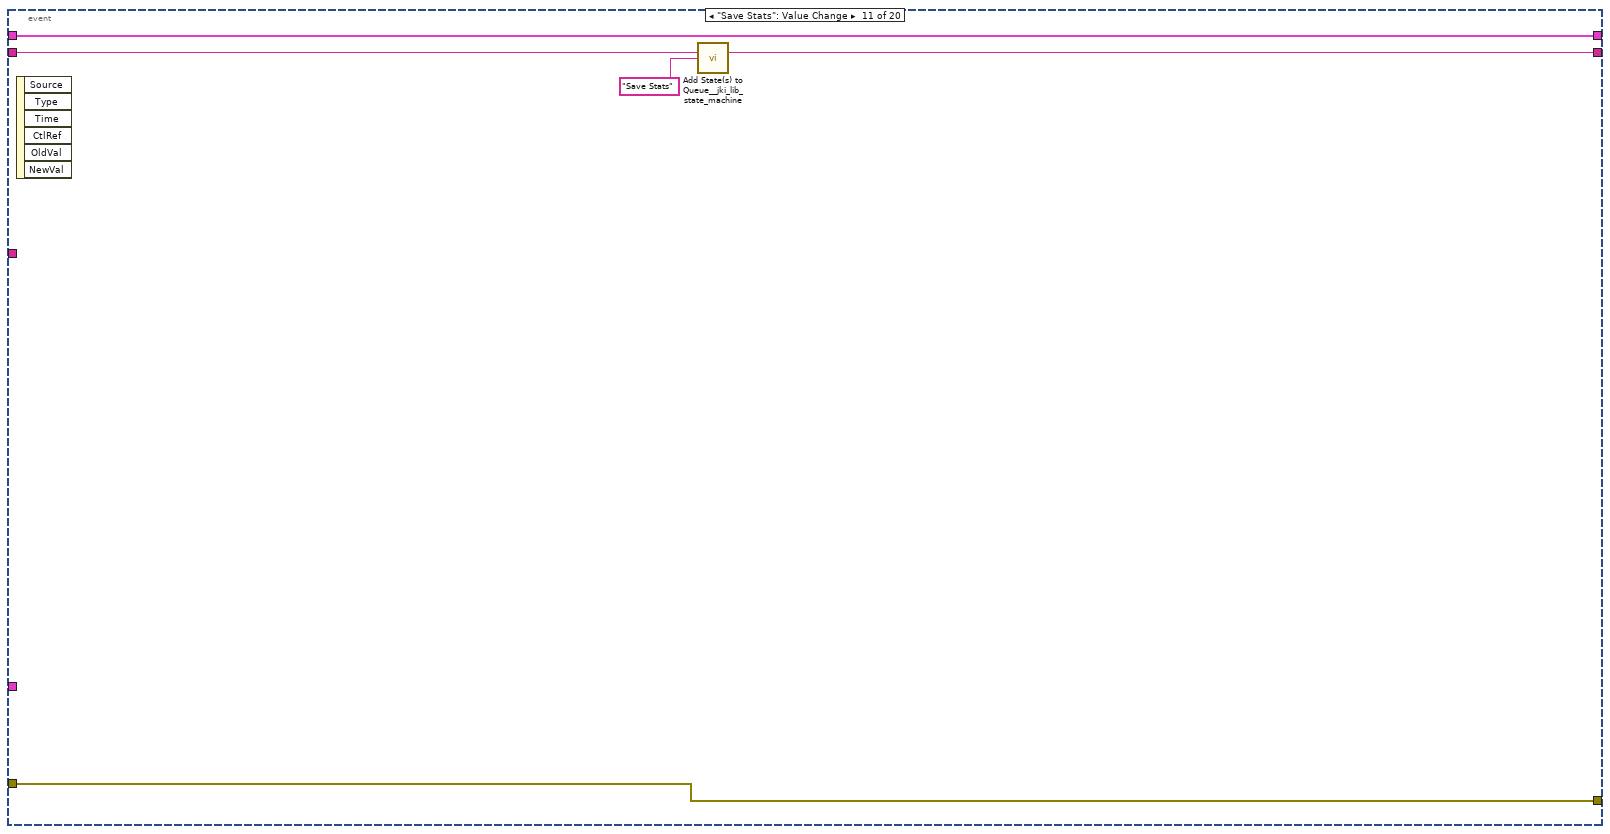
[diagram p20: hidden frame]
diagram:
  n1 = control-ref of="Target.X::1"() -> (w43:refnum<vi>)
  n2 = control-ref of="Target.Y::1"() -> (w42:refnum<vi>)
  n3 = control-ref of="Target.X::2"() -> (w41:refnum<vi>)
  n4 = control-ref of="Target.Y::2"() -> (w40:refnum<vi>)
  n5 = control-ref of="Target.X::3"() -> (w39:refnum<vi>)
  n6 = control-ref of="Target.Y::3"() -> (w38:refnum<vi>)
  n7 = control-ref of="Target.X::4"() -> (w37:refnum<vi>)
  n8 = control-ref of="Target.Y::4"() -> (w36:refnum<vi>)
  n9 = control-ref of="Target.X::5"() -> (w35:refnum<vi>)
  n10 = control-ref of="Target.Y::5"() -> (w34:refnum<vi>)
  n11 = control-ref of="Target.X::6"() -> (w33:refnum<vi>)
  n12 = control-ref of="Target.Y::6"() -> (w32:refnum<vi>)
  n13 = control-ref of="Target.X::7"() -> (w31:refnum<vi>)
  n14 = control-ref of="Target.Y::7"() -> (w30:refnum<vi>)
  n15 = control-ref of="Target.X::8"() -> (w29:refnum<vi>)
  n16 = control-ref of="Target.Y::8"() -> (w28:refnum<vi>)
  n17 = control-ref of="Target.X::9"() -> (w14:refnum<vi>)
  n18 = control-ref of="Target.Y::9"() -> (w13:refnum<vi>)
  n19 = control-ref of="Target.X::10"() -> (w12:refnum<vi>)
  n20 = control-ref of="Target.Y::10"() -> (w11:refnum<vi>)
  n21 = control-ref of="Target.X::11"() -> (w10:refnum<vi>)
  n22 = control-ref of="Target.Y::11"() -> (w9:refnum<vi>)
  n23 = control-ref of="Target.X::12"() -> (w8:refnum<vi>)
  n24 = control-ref of="Target.Y::12"() -> (w7:refnum<vi>)
  n25 = Bundle("Target.X::1"=w43, "Target.Y::1"=w42) -> (w27:T10)  [unwired: 1 in]
  n26 = Bundle("Target.X::2"=w41, "Target.Y::2"=w40) -> (w26:T11)  [unwired: 1 in]
  n27 = Bundle("Target.X::3"=w39, "Target.Y::3"=w38) -> (w25:T12)  [unwired: 1 in]
  n28 = Bundle("Target.X::4"=w37, "Target.Y::4"=w36) -> (w18:T13)  [unwired: 1 in]
  n29 = Bundle("Target.X::5"=w35, "Target.Y::5"=w34) -> (w24:T14)  [unwired: 1 in]
  n30 = Bundle("Target.X::6"=w33, "Target.Y::6"=w32) -> (w23:T15)  [unwired: 1 in]
  n31 = Bundle("Target.X::7"=w31, "Target.Y::7"=w30) -> (w22:T16)  [unwired: 1 in]
  n32 = Bundle("Target.X::8"=w29, "Target.Y::8"=w28) -> (w21:T17)  [unwired: 1 in]
  n33 = Bundle("Target.X::12"=w8, "Target.Y::12"=w7) -> (w3:T18)  [unwired: 1 in]
  n34 = Bundle("Target.X::9"=w14, "Target.Y::9"=w13) -> (w6:T19)  [unwired: 1 in]
  n35 = Bundle("Target.X::10"=w12, "Target.Y::10"=w11) -> (w5:T20)  [unwired: 1 in]
  n36 = Bundle("Target.X::11"=w10, "Target.Y::11"=w9) -> (w4:T21)  [unwired: 1 in]
  n37 = Tick Count (ms)() -> (millisecond timer value=→"millisecond timer value":u32)
  n38 = disable-structure shown="Disabled" {
    frame Disabled {
    }
    frame Enabled {
    }
  }
  n39 = Build Array(w27, w26, w25, w18, w24, w23, w22, w21, w6, w5, w4, w3) -> (w20:T22)
  n40 = property on="Feedback Global" class="Bool (strict)"("Value"=FALSE ("Feedback Global")) -> ()  [unwired: 2 in, 2 out]
  n41 = call <vilib>:"Add State(s) to Queue__jki_lib_state_machine.vi"("State(s) in (\"\")"="Macro: Initialize") -> ("States Out"=w47:string)  [unwired: 14 in]
  n42 = while "JKI - String-Based Queued State Machine (Basic) v1.0" {
    shift-right: [w62] -> w17
    shift-left: _ -> [w56]
    shift-right: [w64] -> w44
    shift-left: _ -> [w61]
    shift-right: [w50] -> _
    shift-left: w47 -> [w65]
    tunnel: w20 -> [w59]
    tunnel: [w51] -> w45
    tunnel: w20 -> [w58]
    stop <- w63 stop-if-true
    n43 = Unbundle By Name(w56) -> ("active cams"=w55:string[], "Mean Centroid X"=w54:dbl[][], "Mean Centroid Y"=w53:dbl[][], "Mean Size"=w52:dbl[][])
    n44 = call <vilib>:"Parse State Queue__jki_lib_state_machine.vi"("State Queue"=w65, "Error In (no error)"=w61) -> ("Remaining States"=w67:string, "Current State"=w48:string, "Arguments"=w66:string)  [unwired: 11 in]
    "Current State" <- w48
    n45 = local read "CCDs"() -> (w51:string[])
    n46 = case shown="\"Motor Config\"" w48 {
      selector: w48 -> [_ _ w413 _ _ _ _ _ _ _ _ _ _ _ _ _ _ _ _ _ _ _ _ _ _ _ _ _ _ _ _ _ _ _ _ _ _ _ _ _ _ _ _ _ _ _ _ _ _]
      tunnel: w67 -> [w133 w411 w417 w436 w443 w449 w454 w495 w506 w514 w524 w529 w536 w548 w573 w579 w589 w600 w612 w617 w651 w698 w716 w746 w767 w795 w872 w919 w929 w940 w968 w973 w995 w1140 w1307 w1370 w1414 w1467 w1517 w1552 w1568 w1644 w1693 w1704 w1746 w1840 w1867 w1882 w1906]
      tunnel: w66 -> [_ _ _ _ _ _ _ _ _ _ _ _ w531 w543 _ _ _ _ _ _ w618 _ _ _ _ w773 _ w906 _ _ _ _ w996 _ w1292 w1360 w1404 w1452 w1511 _ _ _ _ _ _ _ _ w1886 _]
      tunnel: w56 -> [w131 w408 w415 w426 w440 w447 w451 _ w499 w511 w521 w527 w534 w542 w570 w576 w585 w597 w604 w614 w629 w696 w714 w744 w752 w788 w870 w902 w925 w936 w961 w970 w984 w1123 w1284 w1351 w1393 w1439 w1513 w1549 w1565 w1640 w1690 w1701 w1720 w1838 w1864 w1885 w1897]
      tunnel: [w130 w409 w419 w434 errorcluster {"status"=FALSE, "code"=0, "source"=""} ("error out") w446 w452 w463 w504 w510 w522 w526 w532 w545 w571 w577 w587 w598 w610 w615 w633 w695 w713 w743 w749 w791 w868 w910 w927 w938 w966 w971 w1024 w1153 w1305 w1368 w1412 w1465 w1509 w1550 w1566 w1641 w1691 w1702 w1713 w1809 w1865 w1880 w1904] -> w64
      tunnel: w61 -> [w129 w409 w418 w434 w439 w446 w452 w463 w497 w510 w522 w526 w533 w546 w571 w577 w587 w598 w610 w615 w621 w695 w713 w743 w750 w792 w869 w909 w927 w938 w966 w971 w1024 w1153 w1305 w1368 w1412 w1465 w1510 w1550 w1566 w1642 w1691 w1702 w1714 w1836 w1865 w1880 w1904]
      tunnel: [w132 w410 w416 w435 w442 w448 w453 w494 w505 w513 w523 w528 w535 w547 w572 w578 w588 w599 w611 w616 w650 w697 w715 w745 w766 w782 w871 w918 w928 w939 w967 w972 w978 w1154 w1306 w1369 w1413 w1466 w1516 w1551 w1567 w1643 w1692 w1703 w1745 w1839 w1866 w1881 w1905] -> w50
      tunnel: [_ _ _ _ _ TRUE _ _ _ _ _ _ _ _ _ _ _ _ _ _ _ _ _ _ _ _ _ _ _ _ _ _ _ _ _ _ _ _ _ _ _ _ _ _ _ _ _ _ _] -> w63
      tunnel: [w126 w408 w415 w425 w440 w447 w451 w464 w499 w511 w521 w527 w534 w542 w570 w576 w584 w597 w604 w614 w642 w696 w714 w744 w751 w793 w870 w913 w924 w937 w960 w970 w977 w1124 w1279 w1350 w1392 w1438 w1515 w1549 w1565 w1640 w1689 w1701 w1720 w1837 w1864 w1884 w1896] -> w62
      tunnel: "update speed [ms]" -> [w128 _ _ _ _ _ _ _ _ _ _ _ _ _ _ _ _ _ _ _ _ _ _ _ _ _ _ _ _ _ _ _ _ _ _ _ _ _ _ _ _ _ _ _ _ _ _ _ _]
      tunnel: w59 -> [w125 _ _ _ _ _ _ _ _ _ _ _ _ _ _ _ _ _ _ _ _ _ _ _ _ _ _ _ _ _ _ _ w975 _ _ _ _ _ _ _ _ _ _ _ _ _ w1849 _ _]
      tunnel: w51 -> [w127 _ _ _ _ _ _ _ _ _ _ _ _ _ _ _ _ _ _ _ _ _ _ _ _ w794 _ w914 _ _ _ _ w988 w1125 w1304 _ _ w1464 w1512 _ w1555 _ _ _ w1719 _ _ _ _]
      tunnel: [w124 w407 w412 w424 w437 w444 w450 w456 w502 w507 w520 w525 w530 w541 w569 w574 w580 w591 w601 w613 w628 w694 w699 w717 w747 w769 w854 w900 w920 w932 w959 w969 w976 w1114 w1288 w1359 w1403 w1445 w1508 w1548 w1553 w1622 w1684 w1700 w1705 w1810 w1847 w1876 w1887] -> w49
      tunnel: w48 -> [w124 w407 w412 w424 w437 w444 w450 w456 w502 w507 w520 w525 w530 w541 w569 w574 w580 w591 w601 w613 w628 w694 w699 w717 w747 w769 w854 w900 w920 w932 w959 w969 w976 w1114 w1288 w1359 w1403 w1445 w1508 w1548 w1553 w1622 w1684 w1700 w1705 w1810 w1847 w1876 w1887]
      frame "", "Idle" {
        # "executes when the state queue is empty"
        n47 = event shown="[0] Timeout" {
          selector: _ -> [_ _ _ _ _ _ _ _ _ _ _ _ _ _ _ _ _ _ _ _]
          dyn-events: _ -> [_ _ _ _ _ _ _ _ _ _ _ _ _ _ _ _ _ _ _ _]
          timeout: w128 -> [_ _ _ _ _ _ _ _ _ _ _ _ _ _ _ _ _ _ _ _]
          tunnel: w133 -> [w141 w262 w277 w302 w307 w312 w317 w323 w328 w333 w338 w340 w355 w367 w372 w377 w383 w392 w396 w406]
          tunnel: [w164 w261 w276 w301 w306 w311 w316 w322 w327 w332 w337 w339 w354 w366 w371 w376 w382 w391 w395 w405] -> w132
          tunnel: w131 -> [w135 w259 w273 w298 w304 w309 w314 w320 w325 w330 w335 w343 w353 w365 w370 w375 w381 w385 w397 w403]
          tunnel: [w174 w260 w275 w300 w305 w310 w315 w321 w326 w331 w336 w342 w348 w360 w369 w374 w380 w390 w394 w404] -> w130
          tunnel: w129 -> [w152 w260 w275 w300 w305 w310 w315 w321 w326 w331 w336 w342 w349 w361 w369 w374 w380 w390 w394 w404]
          tunnel: [w163 w259 w273 w297 w304 w309 w314 w320 w325 w330 w335 w343 w353 w365 w370 w375 w381 w385 w397 w403] -> w126
          tunnel: w127 -> [w157 _ w269 _ _ _ _ _ _ _ _ _ _ _ _ _ _ _ _ _]
          tunnel: w125 -> [_ _ w271 _ _ _ _ _ _ _ _ _ _ _ _ _ _ _ _ _]
          event Timeout {
            n48 = event-data() -> ()  [unwired: 1 in, 1 out]
            n49 = Unbundle By Name(w135) -> ("Centroid X"=w158:dbl[][], "Centroid Y"=w155:dbl[][], "Size"=w153:dbl[][], "detection para"=w136:T7[], "active cams"=w156:string[], "thresholds"=w154:cluster{"Lower value":sgl, "Upper value":sgl}[])
            n50 = Unbundle By Name(w135) -> ("img to avg"=w138:i32, "active ccd"=w160:i32)
            n51 = for {
              tunnel: w156 -> [w195] mode=indexing
              tunnel: [w196] -> w145 mode=indexing
              tunnel: w157 -> [w218]
              tunnel: w136 -> [w216]
              tunnel: [w179] -> w144 mode=indexing
              tunnel: [w214] -> w151 mode=indexing
              tunnel: [w212] -> w159 mode=indexing
              tunnel: "autodetect" -> [w206]
              tunnel: w152 -> [w219]
              tunnel: [w220] -> w150
              shift-right: [w203] -> w148
              shift-left: w154 -> [w205]
              shift-right: [w190] -> w137
              shift-left: w158 -> [w192]
              shift-right: [w186] -> w147
              shift-left: w155 -> [w188]
              shift-right: [w180] -> w146
              shift-left: w153 -> [w182]
              w184 = 0 ("index")
              n52 = call-poly <userlib>:"Filter 1D Array__ogtk.vi"("items to filter"=w195, "array"=w218) -> ("filtered item indices"=w217:i32[])  [unwired: 4 in, 1 out]
              n53 = Index Array(array=w217) -> (element=w181:i32)  [unwired: 1 in]
              n54 = Index Array(array=w182, index (row)=w181) -> (element=w210:dbl[])  [unwired: 1 in]
              n55 = Index Array(array=w188, index (row)=w181) -> (element=w211:dbl[])  [unwired: 1 in]
              n56 = Index Array(array=w205, index=w181) -> (element=w209:cluster{"Lower value":sgl, "Upper value":sgl})
              n57 = Index Array(array=w192, index (row)=w181) -> (element=w194:dbl[])  [unwired: 1 in]
              n58 = Index Array(array=w216, index=w181) -> (element=w213:T7)
              n59 = call "CENTRIOD DETECTION.vi"("Refnum in"=w195, "auto threshold"=w206, "Threshold Range In"=w209, "beam detection para"=w213, "error in (no error)"=w219) -> ("Bounding Rect"=w212:T29, "Particle Reports (Pixels)"=w214:T2, "Threshold Range Out"=w204:cluster{"Lower value":sgl, "Upper value":sgl}, "Centriod"=w221:cluster{"X":dbl, "Y":dbl}, "error out"=w220:errorcluster)  [unwired: 7 in, 3 out]
              n60 = Unbundle By Name(w221) -> ("X"=w193:dbl, "Y"=w189:dbl)
              n61 = Empty Array?(array=w214) -> (empty?=w215:bool)
              n62 = Not(x=w215) -> (.not. x?=w179:bool)
              n63 = Replace Array Subset(array=w205, new element=w204, index=w181) -> (w203:cluster{"Lower value":sgl, "Upper value":sgl}[])
              n64 = Unbundle By Name(w212) -> ("Right"=w202:dbl, "Left"=w201:dbl, "Bottom"=w200:dbl, "Top"=w199:dbl)
              n65 = Subtract(x=w202, y=w201) -> (x-y=w197:dbl)
              n66 = Subtract(x=w200, y=w199) -> (x-y=w198:dbl)
              n67 = Multiply(x=w197, y=w198) -> (x*y=w185:dbl)
              n68 = Insert Into Array(array=w211, index=w184, new element=w189) -> (w187:dbl[])
              n69 = Insert Into Array(array=w194, index=w184, new element=w193) -> (w191:dbl[])
              n70 = Insert Into Array(array=w210, index=w184, new element=w185) -> (w183:dbl[])
              n71 = for {
                shift-right: [w222] -> w207
                shift-left: dbl[] [] ("Array 4") -> [w225]
                tunnel: w187 -> [w223] mode=indexing
                n72 = Equal To 0?(x=w223) -> (x = 0?=w224:bool)
                n73 = case shown="False" w224 {
                  tunnel: w225 -> [w228 w229]
                  tunnel: w223 -> [w227 _]
                  tunnel: [w226 w229] -> w222
                  frame False {
                    n74 = Build Array (concatenate)(w228, w227) -> (w226:dbl[])
                  }
                  frame True {
                  }
                }
              }
              n75 = Replace Array Subset(array=w192, new element=w191, index (row)=w181) -> (w190:dbl[][])  [unwired: 1 in]
              n76 = Replace Array Subset(array=w188, new element=w187, index (row)=w181) -> (w186:dbl[][])  [unwired: 1 in]
              n77 = Replace Array Subset(array=w182, new element=w183, index (row)=w181) -> (w180:dbl[][])  [unwired: 1 in]
              n78 = Array Size(array=w207) -> (size(s)=w196:i32)
            }
            "detected" <- w144
            "Box" <- w159
            n79 = Index Array(array=w151, index (row)=w160) -> (element=→"particles":T2)  [unwired: 1 in]
            n80 = call <vilib>:"Clear Errors.vi"("error in (no error)"=w150) -> ("error out"=w174:errorcluster)  [unwired: 5 in, 1 out]
            n81 = Increment(x=w138) -> (x+1=w165:i32)
            n82 = Greater Or Equal?(x="#imgs avd so far", y=w165) -> (x >= y?=w162:bool)
            n83 = Increment(x="#imgs avd so far") -> (x+1=w167:dbl)
            n84 = Select(t=0.0, s=w162, f=w167) -> (s? t:f=w166:dbl)
            n85 = local write "#imgs avd so far"(w166) -> ()
            n86 = for {
              tunnel: w145 -> [w251] mode=indexing
              tunnel: w156 -> [w257] mode=indexing
              shift-right: [w252] -> w175
              shift-left: "" ("GUIdevice 7") -> [w255]
              tunnel: [w246] -> w177 mode=indexing
              tunnel: "Detection Rate" -> [w250]
              tunnel: w166 -> [w248]
              tunnel: w138 -> [w244]
              n87 = Greater Or Equal?(x=w251, y=w244) -> (x >= y?=w247:bool)
              n88 = Multiply(x=w250, y=w248) -> (x*y=w249:dbl)
              n89 = Greater Or Equal?(x=w251, y=w249) -> (x >= y?=w245:bool)
              n90 = And(x=w247, y=w245) -> (x .and. y?=w246:bool)
              n91 = Select(t=w257, s=w246, f="") -> (s? t:f=w253:string)
              n92 = Concatenate Strings(w255, "\t", w253) -> (w252:string)
            }
            n93 = Bundle By Name(cluster=w135, "thresholds"=w148) -> (w170:T31)
            n94 = Bundle(0, 1, "Centroid X"=w137) -> (→"Status":cluster{i32, i32, "Centroid X":dbl[][]})  [unwired: 1 in]
            n95 = call <vilib>:"Add State(s) to Queue__jki_lib_state_machine.vi"("State(s) in (\"\")"=w141, "State(s) at Back (\"\")"="Device Ini\nactive" ("State(s) at Back (\"\")")) -> ("States Out"=w140:string)  [unwired: 13 in]
            n96 = Bundle By Name(cluster=w170, "Centroid X"=w137, "Centroid Y"=w147, "Size"=w146) -> (w143:T31)
            n97 = Unbundle By Name(w143) -> ("img to avg"=w142:i32)
            n98 = case shown="True" w162 {
              tunnel: w143 -> [w230 w237]
              tunnel: [w230 w236] -> w163
              tunnel: w142 -> [_ w232]
              frame False {
              }
              frame True {
                n99 = Decrement(x=w232) -> (x-1=w235:i32)
                n100 = Initialize Array(0.0 ("element"), 12 ("dimension size"), w235) -> (w231:dbl[][])
                n101 = Bundle By Name(cluster=w237, "Centroid X"=w231, "Centroid Y"=w231, "Size"=w231) -> (w236:T31)
              }
            }
            n102 = Or Array Elements(Boolean array=w177) -> (logical OR=w176:bool)
            n103 = case shown="True" w176 {
              tunnel: w175 -> [_ w242]
              tunnel: w140 -> [w238 w241]
              tunnel: [w238 w240] -> w164
              frame False {
              }
              frame True {
                n104 = call <vilib>:"Build State String with Arguments__jki_lib_state_machine.vi"("Arguments (\"\")"=w242, "State"="detected") -> ("State with Arguments"=w239:string)  [unwired: 4 in]
                n105 = call <vilib>:"Add State(s) to Queue__jki_lib_state_machine.vi"("State(s) in Front (\"\")"=w239, "State(s) in (\"\")"=w241) -> ("States Out"=w240:string)  [unwired: 13 in]
              }
            }
          }
          event "stop": Value Change {
            # "Exit Button Value Change (pressed) Event\n(this executes Macro: Exit to terminate the VI)"
            n106 = event-data() -> ()  [unwired: 1 in, 6 out]
            n107 = call <vilib>:"Add State(s) to Queue__jki_lib_state_machine.vi"("State(s) in Front (\"\")"="Macro: Exit", "State(s) in (\"\")"=w262) -> ("States Out"=w261:string)  [unwired: 13 in]
          }
          event Value Change {
            n108 = event-data() -> ()  [unwired: 1 in, 6 out]
            n109 = property on="Set Centriod Target" class="Bool (strict)"("Value"=FALSE) -> ()  [unwired: 2 in, 2 out]
            n110 = Unbundle By Name(w273) -> ("active ccd"=w265:i32, "Mean Centroid X"=w264:dbl[][], "Mean Centroid Y"=w263:dbl[][])
            n111 = Index Array(array=w269, index=w265) -> (element=w268:string)
            n112 = Concatenate Strings("Do want to update the target of " ("message"), w268, "?" ("string")) -> (w266:string)
            n113 = Two Button Dialog(message=w266) -> (T button?=w272:bool)  [unwired: 2 in]
            n114 = case shown="True" w272 {
              tunnel: w271 -> [_ w286]
              tunnel: w265 -> [_ w285]
              tunnel: w264 -> [_ w292]
              tunnel: w263 -> [_ w287]
              frame False {
              }
              frame True {
                n115 = Index Array(array=w292, index (row)=w285) -> (element=w291:dbl[])  [unwired: 1 in]
                n116 = Index Array(array=w287, index (row)=w285) -> (element=w288:dbl[])  [unwired: 1 in]
                n117 = Index Array(array=w286, index=w285) -> (element=w284:T18)
                n118 = Unbundle By Name(w284) -> ("Target.X::12"=w283:refnum<vi>, "Target.Y::12"=w282:refnum<vi>)
                n119 = Reverse 1D Array(array=w291) -> (reversed array=w290:dbl[])
                n120 = Reverse 1D Array(array=w288) -> (reversed array=w289:dbl[])
                n121 = Index Array(array=w290) -> (element=w281:dbl)  [unwired: 1 in]
                n122 = Index Array(array=w289) -> (element=w279:dbl)  [unwired: 1 in]
                n123 = To Unsigned Word Integer(number=w279) -> (unsigned 16bit integer=w278:u16)
                n124 = To Unsigned Word Integer(number=w281) -> (unsigned 16bit integer=w280:u16)
                n125 = disable-structure shown="Enabled" {
                  disable-tunnel: w283 -> [w296 _]
                  disable-tunnel: w280 -> [w295 _]
                  disable-tunnel: w282 -> [w294 _]
                  disable-tunnel: w278 -> [w293 _]
                  frame Enabled {
                    n126 = property class="DigNum (strict)"(reference=w296, "Val(Sgnl)"=w295) -> ()  [unwired: 1 in, 2 out]
                    n127 = property class="DigNum (strict)"(reference=w294, "Val(Sgnl)"=w293) -> ()  [unwired: 1 in, 2 out]
                  }
                  frame Disabled {
                  }
                }
              }
            }
            n128 = call <vilib>:"Add State(s) to Queue__jki_lib_state_machine.vi"("State(s) in (\"\")"=w277) -> ("States Out"=w276:string)  [unwired: 14 in]
          }
          event "Feedback Global": Value Change {
            # "Exit Button Value Change (pressed) Event\n(this executes Macro: Exit to terminate the VI)"
            n129 = event-data() -> ("NewVal"=w299:bool)  [unwired: 1 in, 5 out]
            n130 = call <vilib>:"Add State(s) to Queue__jki_lib_state_machine.vi"("State(s) in (\"\")"=w302) -> ("States Out"=w301:string)  [unwired: 14 in]
            n131 = Bundle By Name(cluster=w298, "Feedback global"=w299) -> (w297:T31)
          }
          event Value Change {
            n132 = event-data() -> ()  [unwired: 1 in, 6 out]
            n133 = call <vilib>:"Add State(s) to Queue__jki_lib_state_machine.vi"("State(s) in Front (\"\")"="Move Config", "State(s) in (\"\")"=w307) -> ("States Out"=w306:string)  [unwired: 13 in]
          }
          event Value Change {
            n134 = event-data() -> ()  [unwired: 1 in, 6 out]
            n135 = call <vilib>:"Add State(s) to Queue__jki_lib_state_machine.vi"("State(s) in Front (\"\")"="Detection Config", "State(s) in (\"\")"=w312) -> ("States Out"=w311:string)  [unwired: 13 in]
          }
          event "Cameras and motors": Value Change {
            n136 = event-data() -> ()  [unwired: 1 in, 6 out]
            n137 = call <vilib>:"Add State(s) to Queue__jki_lib_state_machine.vi"("State(s) in (\"\")"=w317, "State(s) at Back (\"\")"="Motor Config" ("State(s) at Back (\"\")")) -> ("States Out"=w316:string)  [unwired: 13 in]
          }
          event "Reset History": Value Change {
            n138 = event-data() -> ()  [unwired: 1 in, 6 out]
            n139 = call <vilib>:"Add State(s) to Queue__jki_lib_state_machine.vi"("State(s) in (\"\")"=w323, "State(s) at Back (\"\")"="Reset History" ("State(s) at Back (\"\")")) -> ("States Out"=w322:string)  [unwired: 13 in]
            n140 = property on="Reset History" class="Bool (strict)"("Value"=FALSE ("Reset History")) -> ()  [unwired: 2 in, 2 out]
          }
          event "Save Config": Value Change {
            n141 = event-data() -> ()  [unwired: 1 in, 6 out]
            n142 = call <vilib>:"Add State(s) to Queue__jki_lib_state_machine.vi"("State(s) in (\"\")"=w328, "State(s) at Back (\"\")"="Save Config" ("State(s) at Back (\"\")")) -> ("States Out"=w327:string)  [unwired: 13 in]
          }
          event "Load Config": Value Change {
            n143 = event-data() -> ()  [unwired: 1 in, 6 out]
            n144 = call <vilib>:"Add State(s) to Queue__jki_lib_state_machine.vi"("State(s) in (\"\")"=w333, "State(s) at Back (\"\")"="StopSuperGUI\nMacro:Start" ("State(s) at Back (\"\")")) -> ("States Out"=w332:string)  [unwired: 13 in]
          }
          event "Save Stats": Value Change {
            n145 = event-data() -> ()  [unwired: 1 in, 6 out]
            n146 = call <vilib>:"Add State(s) to Queue__jki_lib_state_machine.vi"("State(s) in (\"\")"=w338, "State(s) at Back (\"\")"="Save Stats" ("State(s) at Back (\"\")")) -> ("States Out"=w337:string)  [unwired: 13 in]
          }
          event "Tab Cams": Value Change {
            n147 = event-data() -> ()  [unwired: 1 in, 6 out]
            n148 = call <vilib>:"Add State(s) to Queue__jki_lib_state_machine.vi"("State(s) in (\"\")"=w340, "State(s) at Back (\"\")"="stats" ("State")) -> ("States Out"=w339:string)  [unwired: 13 in]
          }
          event "Left", "Right": Value Change {
            n149 = event-data() -> ("CtlRef"=w352:refnum<vi>)  [unwired: 1 in, 5 out]
            n150 = property class="Bool (strict)"(reference=w352, error in=w349) -> (reference out=w351:refnum<vi>, error out=w350:errorcluster, "Label.Text"=w346:string)
            n151 = property class="Bool (strict)"(reference=w351, error in=w350, "Value"=FALSE) -> (error out=w348:errorcluster)  [unwired: 1 out]
            n152 = call <vilib>:"Build State String with Arguments__jki_lib_state_machine.vi"("Arguments (\"\")"=w346, "State"="ManMove X") -> ("State with Arguments"=w345:string)  [unwired: 4 in]
            n153 = call <vilib>:"Add State(s) to Queue__jki_lib_state_machine.vi"("State(s) in (\"\")"=w355, "State(s) at Back (\"\")"=w345) -> ("States Out"=w354:string)  [unwired: 13 in]
          }
          event "Up", "Down": Value Change {
            n154 = event-data() -> ("CtlRef"=w364:refnum<vi>)  [unwired: 1 in, 5 out]
            n155 = property class="Bool (strict)"(reference=w364, error in=w361) -> (reference out=w363:refnum<vi>, error out=w362:errorcluster, "Label.Text"=w358:string)
            n156 = property class="Bool (strict)"(reference=w363, error in=w362, "Value"=FALSE) -> (error out=w360:errorcluster)  [unwired: 1 out]
            n157 = call <vilib>:"Build State String with Arguments__jki_lib_state_machine.vi"("Arguments (\"\")"=w358, "State"="ManMove Y") -> ("State with Arguments"=w357:string)  [unwired: 4 in]
            n158 = call <vilib>:"Add State(s) to Queue__jki_lib_state_machine.vi"("State(s) in (\"\")"=w367, "State(s) at Back (\"\")"=w357) -> ("States Out"=w366:string)  [unwired: 13 in]
          }
          event "Center": Value Change {
            n159 = event-data() -> ()  [unwired: 1 in, 6 out]
            n160 = call <vilib>:"Add State(s) to Queue__jki_lib_state_machine.vi"("State(s) in (\"\")"=w372, "State(s) at Back (\"\")"="Center" ("State(s) at Back (\"\")")) -> ("States Out"=w371:string)  [unwired: 13 in]
          }
          event "new tdms": Value Change {
            n161 = event-data() -> ()  [unwired: 1 in, 6 out]
            n162 = call <vilib>:"Add State(s) to Queue__jki_lib_state_machine.vi"("State(s) in (\"\")"=w377, "State(s) at Back (\"\")"="newtdms" ("State(s) at Back (\"\")")) -> ("States Out"=w376:string)  [unwired: 13 in]
          }
          event "device ini": Value Change {
            n163 = event-data() -> ()  [unwired: 1 in, 6 out]
            n164 = property on="device ini" class="Bool (strict)"("Value"=FALSE ("test")) -> ()  [unwired: 2 in, 2 out]
            n165 = call <vilib>:"Add State(s) to Queue__jki_lib_state_machine.vi"("State(s) in (\"\")"=w383, "State(s) at Back (\"\")"="Device Ini" ("State(s) at Back (\"\")")) -> ("States Out"=w382:string)  [unwired: 13 in]
          }
          event "active CCDs": Value Change {
            n166 = event-data() -> ("NewVal"=w386:i32)  [unwired: 1 in, 5 out]
            n167 = Unbundle By Name(w385) -> ("active cams"=w387:string[])
            n168 = Index Array(array=w387, index=w386) -> (element=w388:string)
            n169 = call <vilib>:"Build State String with Arguments__jki_lib_state_machine.vi"("Arguments (\"\")"=w388, "State"="active" ("State(s) at Back (\"\")")) -> ("State with Arguments"=w384:string)  [unwired: 4 in]
            n170 = call <vilib>:"Add State(s) to Queue__jki_lib_state_machine.vi"("State(s) in (\"\")"=w392, "State(s) at Back (\"\")"=w384) -> ("States Out"=w391:string)  [unwired: 13 in]
          }
          event "img to avg": Value Change {
            n171 = event-data() -> ("NewVal"=w398:i32)  [unwired: 1 in, 5 out]
            n172 = Number To Decimal String(number=w398) -> (decimal integer string=w400:string)  [unwired: 1 in]
            n173 = call <vilib>:"Build State String with Arguments__jki_lib_state_machine.vi"("Arguments (\"\")"=w400, "State"="ImgToAvg" ("State(s) at Back (\"\")")) -> ("State with Arguments"=w393:string)  [unwired: 4 in]
            n174 = call <vilib>:"Add State(s) to Queue__jki_lib_state_machine.vi"("State(s) in Front (\"\")"=w393, "State(s) in (\"\")"=w396) -> ("States Out"=w395:string)  [unwired: 13 in]
          }
          event Panel Close? {
            # "Discard the event because we'll close the front panel ourselves in Macro: Exit"
            # "Close Panel button (pressed) Event\n(this executes Macro: Exit to terminate the VI)"
            n175 = event-data() -> ()  [unwired: 1 in, 1 out]
            n176 = call <vilib>:"Add State(s) to Queue__jki_lib_state_machine.vi"("State(s) in Front (\"\")"="Macro: Exit", "State(s) in (\"\")"=w406) -> ("States Out"=w405:string)  [unwired: 13 in]
            n177 = event-data("Discard?"=TRUE) -> ()  [unwired: 1 in, 1 out]
          }
        }
      }
      frame "---------- Core ----------" {
        # "Do not put any code in this frame.\n(it is a separator no-op)"
        n178 = call <vilib>:"Add State(s) to Queue__jki_lib_state_machine.vi"("State(s) in (\"\")"=w411) -> ("States Out"=w410:string)  [unwired: 14 in]
      }
      frame Default {
        w422 = 42 items=["No error", "Argument error", "Memory is full", "Out of zone", "End of file", "File already open", "Generic file I/O error", "File not found", "File permission error", "Disk is full", "Duplicate path", "Too many files open", "System feature not enabled", "Resource file not found", "Cannot add resource", "Resource not found", "Image not found", "Image memory error", "Pen does not exist", "Config type invalid", "Config token not found", "Config parse error", "Config memory error", "Bad external code format", "Bad external code offset", "External code not present", "Null window", "Destroy window error", "Null menu", "Print aborted", "Bad print record", "Print driver error", "Windows error during printing", "Memory error during printing", "Print dialog error", "Generic print error", "Invalid device refnum", "Device not found", "Device parameter error", "Device unit error", "Cannot open device", "Device call aborted", "Generic error", "Cancelled by user", "Object ID too low", "Object ID too high", "Object not in heap", "Unknown heap", "Unknown object (invalid DefProc)", "Unknown object (DefProc not in table)", "Message out of range", "Invalid (null) method", "Unknown message", "Manager call not supported", "Bad address", "Network operation in progress", "Network operation timed out", "Connection is busy", "Network attribute not supported", "Network error", "Address in use", "System out of memory", "Connection aborted", "Connection refused", "Not connected", "Already connected", "Connection closed", "Initialization error (interapplication manager)", "Bad occurrence", "Wait on unbound occurrence handler", "Occurrence queue overflow", "Datalog type conflict", "Unused", "Unrecognized type (interapplication manager)", "Memory corrupt", "Failed to make temporary DLL", "Old CIN version", "Drag socket not found", "Failed to load drop-object", "Failed to register OLE object", "Failed to release OLE object", "Format specifier type mismatch", "Unknown format specifier", "Too few format specifiers", "Too many format specifiers", "Scan failed", "Newer CIN version", "Error converting to variant", "Runtime menu error", "Password tampered", "Variant attribute not found", "Incompatible variant data type", "Event data is not available", "Event Store is not present", "Occurrence is not found", "Event Queue is not created", "Event info is not available", "Refnum passed is NULL", "Error retrieving Class GUID", "Error retrieving CoClass GUID", "Error retrieving TypeLib GUID.", "Bad built application magic bytes.", "Specific driver is different from the specific driver associated with the Logical Name.", "There is no session opened to the class driver.", "Max Error", "MAX - Error with config objects", "MAX - Error loading configuration", "MAX - Group not supported"]
        # "Current State"
        # "Do not delete, rename, or modify this frame.\n(this is used to capture unhandled states and typos)"
        # "Handle mistyped state name (developer tool)"
        n179 = Format Into String(format string="Software Exception: Unhandled State \"%s\"." ("message"), error in=w418, w413) -> (resulting string=w421:string, error out=w420:errorcluster)  [unwired: 1 in]
        n180 = call <vilib>:"Error Cluster From Error Code.vi"("show call chain? (False)"=TRUE, "error in (no error)"=w420, "error message (\"\")"=w421, "error code (0)"=w422) -> ("error out"=w419:errorcluster)  [unwired: 5 in]
        n181 = call <vilib>:"Add State(s) to Queue__jki_lib_state_machine.vi"("State(s) in (\"\")"=w417) -> ("States Out"=w416:string)  [unwired: 14 in]
      }
      frame "Initialize Core Data" {
        # "Do not delete, rename, or modify this frame.\n(this is used to determine panel behavior on exit)"
        # "originally closed?"
        # "exe?"
        # "If panel starts closed or is an EXE, then close it when we exit"
        n182 = property class="VI"() -> ("Front Panel.Open"=w433:bool)  [unwired: 2 in, 2 out]
        n183 = property class="App"() -> ("App.Kind"=w432:T23)  [unwired: 2 in, 2 out]
        n184 = control-ref of="Current VI Reference"() -> (w427:refnum<vi>)
        n185 = Not(x=w433) -> (.not. x?=w430:bool)
        n186 = Equal?(x=w432, y=T23."Run Time System" ("Application:Kind")) -> (x = y?=w429:bool)
        n187 = Or(x=w430, y=w429) -> (x .or. y?=w428:bool)
        n188 = Bundle By Name(cluster=w426, "Core.Current VI Reference"=w427, "Core.Close Panel on Exit?"=w428) -> (w425:T31)
        n189 = call <vilib>:"Add State(s) to Queue__jki_lib_state_machine.vi"("State(s) in (\"\")"=w436) -> ("States Out"=w435:string)  [unwired: 14 in]
      }
      frame "Error Handler" {
        # "Unhandled Error -- Display it"
        # "Handle any errors here.\nYou can also output any states to clean-up after errors occur"
        # "Clear error"
        n190 = call <vilib>:"General Error Handler.vi"("error in (no error)"=w439) -> ()  [unwired: 10 in, 5 out]
        n191 = call <vilib>:"Add State(s) to Queue__jki_lib_state_machine.vi"("State(s) in Front (\"\")"="/* Post Error States", "State(s) in (\"\")"=w443) -> ("States Out"=w442:string)  [unwired: 13 in]
      }
      frame "Exit" {
        # "Do not put any code in this frame.\n(No errors that occur here will be handled.)"
        n192 = call <vilib>:"Add State(s) to Queue__jki_lib_state_machine.vi"("State(s) in (\"\")"=w449) -> ("States Out"=w448:string)  [unwired: 14 in]
      }
      frame "---------- Data ----------" {
        # "Do not put any code in this frame.\n(It is a separator no-op. You can make a copy of this frame to create a new Data frame)"
        n193 = call <vilib>:"Add State(s) to Queue__jki_lib_state_machine.vi"("State(s) in (\"\")"=w454) -> ("States Out"=w453:string)  [unwired: 14 in]
      }
      frame "Data: Initialize" {
        w455 = T32 {"Positions x"=[0.0, 0.0, 0.0, 0.0, 0.0, 0.0, 0.0, 0.0, 0.0, 0.0, 0.0, 0.0], "Positions y"=[0.0, 0.0, 0.0, 0.0, 0.0, 0.0, 0.0, 0.0, 0.0, 0.0, 0.0, 0.0]}  # Motor positions
        w457 = T33 {"dev variable alias"=[], "dev variable alias Motors X"=[], "dev variable alias Motors Y"=[]}  # dev var alias arrays
        w477 = dbl[][] []  # Offset Y stats
        w487 = dbl[][] []  # Size
        w486 = dbl[][] []  # Mean Size
        w484 = T30[] [{"Tolerance [pix]"=0.1, "Stepsize"=0.0001, "Invert Direction X"=FALSE, "Invert Direction Y"=TRUE, "enable feedback"=FALSE, "Set Centriod Target"=FALSE}, {"Tolerance [pix]"=0.1, "Stepsize"=0.0001, "Invert Direction X"=FALSE, "Invert Direction Y"=TRUE, "enable feedback"=FALSE, "Set Centriod Target"=FALSE}, {"Tolerance [pix]"=0.1, "Stepsize"=0.0001, "Invert Direction X"=FALSE, "Invert Direction Y"=TRUE, "enable feedback"=FALSE, "Set Centriod Target"=FALSE}, {"Tolerance [pix]"=0.1, "Stepsize"=0.0001, "Invert Direction X"=FALSE, "Invert Direction Y"=TRUE, "enable feedback"=FALSE, "Set Centriod Target"=FALSE}, {"Tolerance [pix]"=0.1, "Stepsize"=0.0001, "Invert Direction X"=FALSE, "Invert Direction Y"=TRUE, "enable feedback"=FALSE, "Set Centriod Target"=FALSE}, {"Tolerance [pix]"=0.1, "Stepsize"=0.0001, "Invert Direction X"=FALSE, "Invert Direction Y"=TRUE, "enable feedback"=FALSE, "Set Centriod Target"=FALSE}, {"Tolerance [pix]"=0.1, "Stepsize"=0.0001, "Invert Direction X"=FALSE, "Invert Direction Y"=TRUE, "enable feedback"=FALSE, "Set Centriod Target"=FALSE}, {"Tolerance [pix]"=0.1, "Stepsize"=0.0001, "Invert Direction X"=FALSE, "Invert Direction Y"=TRUE, "enable feedback"=FALSE, "Set Centriod Target"=FALSE}, {"Tolerance [pix]"=0.1, "Stepsize"=0.0001, "Invert Direction X"=FALSE, "Invert Direction Y"=TRUE, "enable feedback"=FALSE, "Set Centriod Target"=FALSE}, {"Tolerance [pix]"=0.1, "Stepsize"=0.0001, "Invert Direction X"=FALSE, "Invert Direction Y"=TRUE, "enable feedback"=FALSE, "Set Centriod Target"=FALSE}, {"Tolerance [pix]"=0.1, "Stepsize"=0.0001, "Invert Direction X"=FALSE, "Invert Direction Y"=TRUE, "enable feedback"=FALSE, "Set Centriod Target"=FALSE}, {"Tolerance [pix]"=0.1, "Stepsize"=0.0001, "Invert Direction X"=FALSE, "Invert Direction Y"=TRUE, "enable feedback"=FALSE, "Set Centriod Target"=FALSE}, {"Tolerance [pix]"=0.1, "Stepsize"=0.0001, "Invert Direction X"=FALSE, "Invert Direction Y"=TRUE, "enable feedback"=FALSE, "Set Centriod Target"=FALSE}]  # move properties
        w483 = T34 []  # active axis refs 2
        w476 = dbl[][] []  # Motor X
        w475 = dbl[][] []  # Motor Y
        w474 = string[] []  # active cams
        w458 = T35 {"STOP queue"=refnum, "SuperGUI ref"=refnum}  # Supergui
        w459 = dbl[] [0.0, 0.0, 0.0, 0.0, 0.0, 0.0, 0.0, 0.0, 0.0, 0.0, 0.0, 0.0]  # steps speed Y
        w460 = dbl[] [0.0, 0.0, 0.0, 0.0, 0.0, 0.0, 0.0, 0.0, 0.0, 0.0, 0.0, 0.0]  # steps speed X
        w461 = refnum<k34> refnum  # tdms ref
        w462 = bool[] [FALSE, FALSE, FALSE, FALSE, TRUE, TRUE, TRUE, FALSE, FALSE, FALSE, FALSE, FALSE]  # detected
        w470 = bool[] [FALSE, FALSE, FALSE, FALSE, FALSE, FALSE, FALSE, FALSE, FALSE, FALSE, FALSE, TRUE]  # speedmode Y
        w471 = bool[] [FALSE, FALSE, FALSE, FALSE, FALSE, FALSE, FALSE, FALSE, FALSE, FALSE, FALSE, TRUE]  # speedmode X
        w473 = cluster{"Lower value":sgl, "Upper value":sgl}[] [{"Lower value"=93.0, "Upper value"=255.0}, {"Lower value"=105.0, "Upper value"=255.0}, {"Lower value"=0.0, "Upper value"=255.0}, {"Lower value"=127.0, "Upper value"=255.0}, {"Lower value"=0.0, "Upper value"=255.0}, {"Lower value"=0.0, "Upper value"=255.0}, {"Lower value"=0.0, "Upper value"=255.0}, {"Lower value"=0.0, "Upper value"=255.0}, {"Lower value"=0.0, "Upper value"=255.0}, {"Lower value"=0.0, "Upper value"=255.0}, {"Lower value"=0.0, "Upper value"=255.0}, {"Lower value"=0.0, "Upper value"=255.0}]  # thresholds
        w480 = FALSE  # Feedback global
        w482 = 0  # active ccd
        w466 = 6  # img to avg
        w493 = T36 {"Current VI Reference"=refnum, "Close Panel on Exit?"=FALSE}  # Core
        # "Initialize the shift-register data, here.\n(data names are defined by what you wire into the bundle function)"
        n194 = call <vilib>:"Add State(s) to Queue__jki_lib_state_machine.vi"("State(s) in (\"\")"=w495) -> ("States Out"=w494:string)  [unwired: 14 in]
        n195 = Bundle("Core"=w493, "detection para"=T7[] [{"Filter"=1, "Filter Para"={"X Size"=5, "Y Size"=5, "% Tolerance"=1}, "detection method"=4, "smal para"=[{"Measurement Parameter"=35, "Range Lower Value"=0.0, "Range Upper Value"=0.0, "Range"=TRUE, "Measurement Type"=FALSE}], "Remove small Objects"=TRUE, "Restrict to round Objects"=FALSE}, {"Filter"=1, "Filter Para"={"X Size"=5, "Y Size"=5, "% Tolerance"=1}, "detection method"=4, "smal para"=[{"Measurement Parameter"=35, "Range Lower Value"=0.0, "Range Upper Value"=500.0, "Range"=FALSE, "Measurement Type"=FALSE}], "Remove small Objects"=TRUE, "Restrict to round Objects"=FALSE}, {"Filter"=1, "Filter Para"={"X Size"=5, "Y Size"=5, "% Tolerance"=1}, "detection method"=4, "smal para"=[{"Measurement Parameter"=35, "Range Lower Value"=0.0, "Range Upper Value"=500.0, "Range"=TRUE, "Measurement Type"=FALSE}], "Remove small Objects"=TRUE, "Restrict to round Objects"=FALSE}, {"Filter"=1, "Filter Para"={"X Size"=5, "Y Size"=5, "% Tolerance"=1}, "detection method"=4, "smal para"=[{"Measurement Parameter"=35, "Range Lower Value"=0.0, "Range Upper Value"=500.0, "Range"=TRUE, "Measurement Type"=FALSE}], "Remove small Objects"=TRUE, "Restrict to round Objects"=FALSE}, {"Filter"=1, "Filter Para"={"X Size"=5, "Y Size"=5, "% Tolerance"=1}, "detection method"=4, "smal para"=[{"Measurement Parameter"=35, "Range Lower Value"=0.0, "Range Upper Value"=500.0, "Range"=TRUE, "Measurement Type"=FALSE}], "Remove small Objects"=TRUE, "Restrict to round Objects"=FALSE}, {"Filter"=1, "Filter Para"={"X Size"=5, "Y Size"=5, "% Tolerance"=1}, "detection method"=4, "smal para"=[{"Measurement Parameter"=35, "Range Lower Value"=0.0, "Range Upper Value"=500.0, "Range"=TRUE, "Measurement Type"=FALSE}], "Remove small Objects"=TRUE, "Restrict to round Objects"=FALSE}, {"Filter"=1, "Filter Para"={"X Size"=5, "Y Size"=5, "% Tolerance"=1}, "detection method"=4, "smal para"=[{"Measurement Parameter"=35, "Range Lower Value"=0.0, "Range Upper Value"=500.0, "Range"=TRUE, "Measurement Type"=FALSE}], "Remove small Objects"=TRUE, "Restrict to round Objects"=FALSE}, {"Filter"=1, "Filter Para"={"X Size"=5, "Y Size"=5, "% Tolerance"=1}, "detection method"=3, "smal para"=[{"Measurement Parameter"=35, "Range Lower Value"=0.0, "Range Upper Value"=0.0, "Range"=FALSE, "Measurement Type"=FALSE}], "Remove small Objects"=TRUE, "Restrict to round Objects"=FALSE}, {"Filter"=1, "Filter Para"={"X Size"=5, "Y Size"=5, "% Tolerance"=1}, "detection method"=4, "smal para"=[{"Measurement Parameter"=35, "Range Lower Value"=0.0, "Range Upper Value"=0.0, "Range"=FALSE, "Measurement Type"=FALSE}], "Remove small Objects"=TRUE, "Restrict to round Objects"=FALSE}, {"Filter"=1, "Filter Para"={"X Size"=5, "Y Size"=5, "% Tolerance"=1}, "detection method"=4, "smal para"=[{"Measurement Parameter"=35, "Range Lower Value"=0.0, "Range Upper Value"=500.0, "Range"=TRUE, "Measurement Type"=FALSE}], "Remove small Objects"=TRUE, "Restrict to round Objects"=FALSE}, {"Filter"=1, "Filter Para"={"X Size"=5, "Y Size"=5, "% Tolerance"=1}, "detection method"=4, "smal para"=[{"Measurement Parameter"=35, "Range Lower Value"=0.0, "Range Upper Value"=500.0, "Range"=TRUE, "Measurement Type"=FALSE}], "Remove small Objects"=TRUE, "Restrict to round Objects"=FALSE}, {"Filter"=1, "Filter Para"={"X Size"=5, "Y Size"=5, "% Tolerance"=1}, "detection method"=4, "smal para"=[{"Measurement Parameter"=35, "Range Lower Value"=0.0, "Range Upper Value"=500.0, "Range"=TRUE, "Measurement Type"=FALSE}], "Remove small Objects"=TRUE, "Restrict to round Objects"=FALSE}], "thresholds"=w473, "Centroid X"=dbl[][] [], "Centroid Y"=dbl[][] [], "img to avg"=w466, "Mean Centroid X"="Mean Centroid X", "Mean Centroid Y"=dbl[][] [], "Offset X"="Offset X", "Offset Y"=dbl[][] [], "Offset X stats"=dbl[][] [], "Offset Y stats"=w477, "Size"=w487, "Mean Size"=w486, "Time"="Time", "move properties"=w484, "active axis refs 2"=w483, "active ccd"=w482, "Feedback global"=w480, "Motor X"=w476, "Motor Y"=w475, "active cams"=w474, "tdms ref"=w461, "active man refs"="active man refs", "detected"=w462, "speedmode X"=w471, "speedmode Y"=w470, "steps speed X"=w460, "steps speed Y"=w459, "Supergui"=w458, "dev var alias arrays"=w457, "Motor positions"=w455) -> (w465:T31)  [unwired: 1 in]
        n196 = Initialize Array(0.0 ("element"), 12 ("dimension size"), w466) -> (w469:dbl[][])
        n197 = Bundle By Name(cluster=w465, "Centroid X"=w469, "Centroid Y"=w469, "Size"=w469) -> (w464:T31)
      }
      frame "Data: Cleanup" {
        # "Cleanup any data and references, here.\n(this is called automatically, by the Macro: Exit)"
        n198 = Unbundle By Name(w499) -> ("Core.Current VI Reference"=w503:refnum<vi>)
        n199 = Unbundle By Name(w499) -> ("tdms ref"=w501:refnum<k34>)
        n200 = TDMS Close(8:w497, 11:w501) -> (0:w500:errorcluster)  [unwired: 1 out]
        n201 = call <vilib>:"Clear Errors.vi"("error in (no error)"=w500) -> ("error out"=w498:errorcluster)  [unwired: 5 in, 1 out]
        n202 = Merge Errors(w498, w497) -> (w496:errorcluster)
        n203 = Close Reference(reference=w503, error in (no error)=w496) -> (error out=w504:errorcluster)
        n204 = call <vilib>:"Add State(s) to Queue__jki_lib_state_machine.vi"("State(s) in (\"\")"=w506) -> ("States Out"=w505:string)  [unwired: 14 in]
      }
      frame "StopSuperGUI" {
        # "Initialize the User Interface, here.\n(this is called automatically, by the Macro: Init)"
        n205 = Unbundle By Name(w511) -> ("Supergui.SuperGUI ref"=w509:refnum<vi>, "Supergui.STOP queue"=w512:refnum<queue>)
        n206 = Not A Number/Path/Refnum?(number/path/refnum=w509) -> (NaN/Path/Refnum?=w508:bool)
        n207 = case shown="False" w508 {
          tunnel: w512 -> [w519 _]
          tunnel: w509 -> [w515 _]
          frame False {
            n208 = Release Queue(queue=w519) -> (error out=w518:errorcluster)  [unwired: 2 in, 2 out]
            n209 = call-by-ref "Wait On Asynchronous Call"(reference=w515, error in=w518) -> (error out=w517:errorcluster, 0:"error out"=w516:errorcluster)  [unwired: 11 in, 1 out]
            n210 = call <vilib>:"Clear Errors.vi"("error in (no error)"=w516) -> ()  [unwired: 5 in, 2 out]
            n211 = call <vilib>:"Clear Errors.vi"("error in (no error)"=w517) -> ()  [unwired: 5 in, 2 out]
          }
          frame True {
          }
        }
        n212 = call <vilib>:"Add State(s) to Queue__jki_lib_state_machine.vi"("State(s) in (\"\")"=w514) -> ("States Out"=w513:string)  [unwired: 14 in]
      }
      frame "---------- UI ----------" {
        # "Do not put any code in this frame.\n(It is a separator no-op. You can make a copy of this frame to create a new UI frame)"
        n213 = call <vilib>:"Add State(s) to Queue__jki_lib_state_machine.vi"("State(s) in (\"\")"=w524) -> ("States Out"=w523:string)  [unwired: 14 in]
      }
      frame "UI: Initialize" {
        # "Initialize the User Interface, here.\n(this is called automatically, by the Macro: Init)"
        n214 = call <vilib>:"Add State(s) to Queue__jki_lib_state_machine.vi"("State(s) in (\"\")"=w529) -> ("States Out"=w528:string)  [unwired: 14 in]
      }
      frame "UI: Cursor Set" {
        # "Argument"
        # "Set and Unset Cursor Busy.\n(Usage: \"UI: Cursor Set >> Busy|Idle\")"
        n215 = case shown="\"Idle\", Default" w531 {
          tunnel: w533 -> [w538 w540]
          tunnel: [w537 w539] -> w532
          frame "Idle", Default {
            n216 = call <vilib>:"Unset Busy.vi"("error in (no error)"=w538) -> ("error out"=w537:errorcluster)  [unwired: 10 in]
          }
          frame "Busy" {
            n217 = call <vilib>:"Set Busy.vi"("error in (no error)"=w540) -> ("error out"=w539:errorcluster)  [unwired: 9 in, 1 out]
          }
        }
        n218 = call <vilib>:"Add State(s) to Queue__jki_lib_state_machine.vi"("State(s) in (\"\")"=w536) -> ("States Out"=w535:string)  [unwired: 14 in]
      }
      frame "UI: Front Panel State" {
        # "Argument"
        # "Set Front Panel Open or Closed\n(Usage: \"UI: Front Panel State >> Open|Close\")"
        n219 = Unbundle By Name(w542) -> ("Core.Current VI Reference"=w544:refnum<vi>)
        n220 = case shown="\"Open\", Default" w543 {
          tunnel: w546 -> [w552 w563]
          tunnel: [w553 w564] -> w545
          tunnel: w544 -> [_ _]
          frame "Open", Default {
            n221 = property class="VI"(error in=w552) -> (reference out=w550:refnum<vi>, error out=w551:errorcluster, "Front Panel.Open"=w549:bool)  [unwired: 1 in]
            n222 = case shown="False" w549 {
              tunnel: [w556 w559] -> w553
              tunnel: w551 -> [w555 w559]
              tunnel: w550 -> [w554 _]
              frame False {
                n223 = invoke class="VI" method="FP.Open"(reference=w554, error in=w555, "Activate"=TRUE, "State"=T24."Standard") -> (error out=w556:errorcluster)  [unwired: 1 in, 4 out]
              }
              frame True {
              }
            }
          }
          frame "Close" {
            n224 = property class="VI"(error in=w563) -> (reference out=w561:refnum<vi>, error out=w562:errorcluster, "Front Panel.Open"=w560:bool)  [unwired: 1 in]
            n225 = case shown="True" w560 {
              tunnel: [w565 w568] -> w564
              tunnel: w562 -> [w565 w567]
              tunnel: w561 -> [_ w566]
              frame False {
              }
              frame True {
                n226 = invoke class="VI" method="FP.Close"(reference=w566, error in=w567) -> (error out=w568:errorcluster)  [unwired: 1 in, 2 out]
              }
            }
          }
        }
        n227 = call <vilib>:"Add State(s) to Queue__jki_lib_state_machine.vi"("State(s) in (\"\")"=w548) -> ("States Out"=w547:string)  [unwired: 14 in]
      }
      frame "---------- Macro ----------" {
        # "Do not put any code in this frame.\n(It is a separator no-op. You can make a copy of this frame to create a new Macro frame)"
        n228 = call <vilib>:"Add State(s) to Queue__jki_lib_state_machine.vi"("State(s) in (\"\")"=w573) -> ("States Out"=w572:string)  [unwired: 14 in]
      }
      frame "Macro: Initialize" {
        # "Initialization Macro\n(This is called once, when the VI starts)"
        n229 = call <vilib>:"Add State(s) to Queue__jki_lib_state_machine.vi"("State(s) in Front (\"\")"="Data: Initialize\nInitialize Core Data\nUI: Initialize\nUI: Front Panel State >> Open\nGetMotorsFromDB\nMacro:Start", "State(s) in (\"\")"=w579) -> ("States Out"=w578:string)  [unwired: 13 in]
      }
      frame "GetMotorsFromDB" {
        n230 = call "get all aliases of a class.vi"("class (eg motor)"="motor") -> ("dev variable alias"=w583:string[][])  [unwired: 10 in]
        n231 = Bundle By Name(cluster=w585, "dev var alias arrays.dev variable alias"=w583) -> (w584:T31)
        n232 = Index Array(array=w583, index (col)=2 ("disabled index (col)")) -> (element=w581:string[])  [unwired: 1 in]
        "Names" <- w581
        n233 = property on="Motor Alias Y" class="Ring (strict)"("Strings []"=w581) -> ()  [unwired: 2 in, 2 out]
        n234 = property on="Motor Alias X" class="Ring (strict)"("Strings []"=w581) -> ()  [unwired: 2 in, 2 out]
        n235 = call <vilib>:"Add State(s) to Queue__jki_lib_state_machine.vi"("State(s) in (\"\")"=w589) -> ("States Out"=w588:string)  [unwired: 14 in]
      }
      frame "Macro:Start" {
        # "Initialization Macro\n(This is called once, when the VI starts)"
        n236 = local write "config path"("" ("config path")) -> ()
        n237 = property on="img to avg" class="DigNum (strict)"() -> ("Value"=w593:i32)  [unwired: 2 in, 2 out]
        n238 = Number To Decimal String(number=w593) -> (decimal integer string=w595:string)  [unwired: 1 in]
        n239 = call <vilib>:"Build State String with Arguments__jki_lib_state_machine.vi"("Arguments (\"\")"=w595, "State"="ImgToAvg") -> ("State with Arguments"=w592:string)  [unwired: 4 in]
        n240 = call <vilib>:"Add State(s) to Queue__jki_lib_state_machine.vi"("State(s) in Front (\"\")"="Load Config\nSetCameraNameControls\nCameraRefs\nStartSuperGUI\nDevice Ini >> 3000\nnewtdms", "State(s) in (\"\")"=w600, "State(s) at Back (\"\")"=w592) -> ("States Out"=w599:string)  [unwired: 12 in]
      }
      frame "Macro: Exit" {
        # "Exit Macro\n(This is called once, when the VI exits)"
        n241 = Unbundle By Name(w604) -> ("Core.Close Panel on Exit?"=w603:bool)
        n242 = Select(t="UI: Front Panel State >> Close", s=w603, f="") -> (s? t:f=w607:string)
        n243 = call <vilib>:"Add State(s) to Queue__jki_lib_state_machine.vi"("State(s) in Front (\"\")"="StopSuperGUI" ("State(s) in Front (\"\")"), "State(s) in (\"\")"=w607, "State(s) at Back (\"\")"="Data: Cleanup\nExit") -> ("States Out"=w605:string)  [unwired: 12 in]
        n244 = call <vilib>:"Add State(s) to Queue__jki_lib_state_machine.vi"("State(s) in Front (\"\")"=w605, "State(s) in (\"\")"=w612) -> ("States Out"=w611:string)  [unwired: 13 in]
      }
      frame "---------- Ini and Configure ----------" {
        # "Template Separator\n(You can make a copy of, or modify, this frame)"
        n245 = call <vilib>:"Add State(s) to Queue__jki_lib_state_machine.vi"("State(s) in (\"\")"=w617) -> ("States Out"=w616:string)  [unwired: 14 in]
      }
      frame "Load Config" {
        w631 = T37 {"Camera"="", "Motor Alias X"=0, "Motor Alias Y"=0}  # Camera and motors
        w634 = T38 {"Camera names"=[], "Motor aliases x"=[], "Motor aliases y"=[], "detection para"=[], "thresholds"=[], "move properties"=[]}  # BP Configuration
        # "Your code here.\n(You can make a copy of, or modify, this frame)"
        n246 = Unbundle By Name(w629) -> ("detection para"=w648:T7[], "move properties"=w645:T30[], "thresholds"=w640:cluster{"Lower value":sgl, "Upper value":sgl}[])
        n247 = Empty String/Path?(string/path=w618) -> (empty?=w619:bool)
        n248 = case shown="True" w619 {
          tunnel: [w653 w662] -> w622
          tunnel: w621 -> [w652 w661]
          tunnel: [w652 w660] -> w620
          tunnel: w618 -> [w654 _]
          frame False {
            n249 = String To Path(string=w654) -> (path=w653:path)
          }
          frame True {
            n250 = call <vilib>:"Application Directory.vi"() -> ("Application Directory"=w656:path)
            n251 = Build Path(base path=w656, name or relative path=path "cfg") -> (appended path=w658:path)
            n252 = call-poly <userlib>:"File Exists__ogtk.vi"("file path"=w658) -> ("exists"=w657:bool)  [unwired: 6 in, 1 out]
            n253 = case shown="True" w657 {
              tunnel: w658 -> [w666 w667]
              tunnel: [w665 w667] -> w655
              frame False {
                n254 = Create Folder(path (use dialog)=w666) -> (created path=w665:path)  [unwired: 2 in, 2 out]
              }
              frame True {
              }
            }
            n255 = call "File Dialog2"("start path"=w655, "error in"=w661, "pattern (all files)"="*.cfg", "pattern label"="config") -> ("selected path"=w662:path, "error out"=w660:errorcluster)  [unwired: 8 in, 2 out]
          }
        }
        n256 = property on="Load Config" class="Bool (strict)"("Value"=FALSE ("Load Config")) -> ()  [unwired: 2 in, 2 out]
        n257 = Path To String(path=w622) -> (string=→"config path":string)
        n258 = call <userlib>:"MGI Read Anything.vi"("Type of Anything"=w634, "Error In"=w620, "Path (dialog)"=w622) -> ("Error Out"=w624:errorcluster, "Anything"=w625:variant)  [unwired: 5 in, 2 out]
        n259 = Variant To Data(error in=w624, type=w634, Variant=w625) -> (data=w649:T38, error out=w633:errorcluster)
        n260 = Unbundle By Name(w649) -> ("Motor aliases x"=w639:string[], "Motor aliases y"=w635:string[], "Camera names"=w627:string[], "detection para"=w647:T7[], "move properties"=w646:T30[], "thresholds"=w641:cluster{"Lower value":sgl, "Upper value":sgl}[])
        n261 = call-poly <userlib>:"Remove Duplicates from 1D Array__ogtk.vi"("Input Array"=w627) -> ("Output Array"=w626:string[])  [unwired: 1 out]
        "CCDs" <- w626
        n262 = call <vilib>:"Add State(s) to Queue__jki_lib_state_machine.vi"("State(s) in (\"\")"=w651, "State(s) at Back (\"\")"="Motor Config" ("State(s) at Back (\"\")")) -> ("States Out"=w650:string)  [unwired: 13 in]
        n263 = property on="Motor Alias X" class="Ring (strict)"() -> ("Strings []"=w632:string[])  [unwired: 2 in, 2 out]
        n264 = for {
          tunnel: w626 -> [w690]
          tunnel: w647 -> [w692]
          tunnel: w646 -> [w691]
          shift-right: [w685] -> w644
          shift-left: w648 -> [w689]
          shift-right: [w683] -> w643
          shift-left: w645 -> [w688]
          tunnel: w641 -> [w684]
          shift-right: [w680] -> w636
          shift-left: w640 -> [w682]
          tunnel: w639 -> [w679]
          tunnel: w635 -> [w677]
          tunnel: w632 -> [w673]
          tunnel: w631 -> [w675]
          tunnel: [w670] -> w630 mode=indexing
          tunnel: w626 -> [w668] mode=indexing
          i -> [w678]
          n265 = call-poly <userlib>:"Filter 1D Array__ogtk.vi"("items to filter"=w668, "array"=w690) -> ("filtered item indices"=w693:i32[])  [unwired: 4 in, 1 out]
          n266 = Index Array(array=w693) -> (element=w676:i32)  [unwired: 1 in]
          n267 = Index Array(array=w677, index=w676) -> (element=w669:string)
          n268 = Index Array(array=w679, index=w676) -> (element=w672:string)
          n269 = Index Array(array=w692, index=w676) -> (element=w687:T7)
          n270 = Index Array(array=w691, index=w676) -> (element=w686:T30)
          n271 = Index Array(array=w684, index=w676) -> (element=w681:cluster{"Lower value":sgl, "Upper value":sgl})
          n272 = Search 1D Array(1D array=w673, element=w669) -> (index of element=w674:i32)  [unwired: 1 in]
          n273 = Search 1D Array(1D array=w673, element=w672) -> (index of element=w671:i32)  [unwired: 1 in]
          n274 = Bundle By Name(cluster=w675, "Camera"=w668, "Motor Alias Y"=w674, "Motor Alias X"=w671) -> (w670:T37)
          n275 = Replace Array Subset(array=w689, new element=w687, index=w678) -> (w685:T7[])
          n276 = Replace Array Subset(array=w688, new element=w686, index=w678) -> (w683:T30[])
          n277 = Replace Array Subset(array=w682, new element=w681, index=w678) -> (w680:cluster{"Lower value":sgl, "Upper value":sgl}[])
        }
        n278 = property on="Cameras and motors" class="Arr (strict)"("Val(Sgnl)"=w630) -> ()  [unwired: 2 in, 2 out]
        n279 = Bundle By Name(cluster=w629, "detection para"=w644, "move properties"=w643, "thresholds"=w636) -> (w642:T31)
      }
      frame "MotorRefs" {
        n280 = call <vilib>:"Add State(s) to Queue__jki_lib_state_machine.vi"("State(s) in (\"\")"=w698) -> ("States Out"=w697:string)  [unwired: 14 in]
      }
      frame "SetCameraNameControls" {
        # "Initialize the User Interface, here.\n(this is called automatically, by the Macro: Init)"
        n281 = local read "CCDs"() -> (w712:string[])
        n282 = Index Array(array=w712) -> (element #1=w711:string, element #2=w710:string, element #3=w709:string, element #4=w708:string, element #5=w707:string, element #6=w706:string, element #7=w705:string, element #8=w704:string, element #9=w703:string, element #10=w702:string, element #11=w701:string, element #12=w700:string)  [unwired: 12 in]
        n283 = property on="GUIdevice 1" class="Str"("Val(Sgnl)"=w711) -> ()  [unwired: 2 in, 2 out]
        n284 = property on="GUIdevice 2" class="Str"("Val(Sgnl)"=w710) -> ()  [unwired: 2 in, 2 out]
        n285 = property on="GUIdevice 3" class="Str"("Val(Sgnl)"=w709) -> ()  [unwired: 2 in, 2 out]
        n286 = property on="GUIdevice 4" class="Str"("Val(Sgnl)"=w708) -> ()  [unwired: 2 in, 2 out]
        n287 = property on="GUIdevice 5" class="Str"("Val(Sgnl)"=w707) -> ()  [unwired: 2 in, 2 out]
        n288 = property on="GUIdevice 6" class="Str"("Val(Sgnl)"=w706) -> ()  [unwired: 2 in, 2 out]
        n289 = property on="GUIdevice 7" class="Str"("Val(Sgnl)"=w705) -> ()  [unwired: 2 in, 2 out]
        n290 = property on="GUIdevice 8" class="Str"("Val(Sgnl)"=w704) -> ()  [unwired: 2 in, 2 out]
        n291 = property on="GUIdevice 9" class="Str"("Val(Sgnl)"=w703) -> ()  [unwired: 2 in, 2 out]
        n292 = property on="GUIdevice 10" class="Str"("Val(Sgnl)"=w702) -> ()  [unwired: 2 in, 2 out]
        n293 = property on="GUIdevice 11" class="Str"("Val(Sgnl)"=w701) -> ()  [unwired: 2 in, 2 out]
        n294 = property on="GUIdevice 12" class="Str"("Val(Sgnl)"=w700) -> ()  [unwired: 2 in, 2 out]
        n295 = call <vilib>:"Add State(s) to Queue__jki_lib_state_machine.vi"("State(s) in (\"\")"=w716) -> ("States Out"=w715:string)  [unwired: 14 in]
      }
      frame "CameraRefs" {
        w718 = T39 0 items=["Grayscale (U8)", "Grayscale (I16)", "Grayscale (SGL)", "Complex (CSG)", "RGB (U32)", "HSL (U32)", "RGB (U64)", "Grayscale (U16)"] ("Image Type")
        n296 = property on="image::5" class="ImageControl"("Caption.Text"="GUIdevice 5") -> ()  [unwired: 2 in, 2 out]
        n297 = property on="image::7" class="ImageControl"("Caption.Text"="GUIdevice 7") -> ()  [unwired: 2 in, 2 out]
        n298 = property on="image::6" class="ImageControl"("Caption.Text"="GUIdevice 6") -> ()  [unwired: 2 in, 2 out]
        n299 = property on="image::9" class="ImageControl"("Caption.Text"="GUIdevice 9") -> ()  [unwired: 2 in, 2 out]
        n300 = property on="image::1" class="ImageControl"("Caption.Text"="GUIdevice 1") -> ()  [unwired: 2 in, 2 out]
        n301 = property on="image::10" class="ImageControl"("Caption.Text"="GUIdevice 10") -> ()  [unwired: 2 in, 2 out]
        n302 = property on="image::8" class="ImageControl"("Caption.Text"="GUIdevice 8") -> ()  [unwired: 2 in, 2 out]
        n303 = property on="image::2" class="ImageControl"("Caption.Text"="GUIdevice 2") -> ()  [unwired: 2 in, 2 out]
        n304 = property on="image::4" class="ImageControl"("Caption.Text"="GUIdevice 4") -> ()  [unwired: 2 in, 2 out]
        n305 = property on="image::3" class="ImageControl"("Caption.Text"="GUIdevice 3") -> ()  [unwired: 2 in, 2 out]
        n306 = property on="image::11" class="ImageControl"("Caption.Text"="GUIdevice 11") -> ()  [unwired: 2 in, 2 out]
        n307 = property on="image::12" class="ImageControl"("Caption.Text"="GUIdevice 12") -> ()  [unwired: 2 in, 2 out]
        n308 = call "IMAQ Create"("Image Name"="GUIdevice 8", "Image Type"=w718) -> ("New Image"=→"image::8":T5)  [unwired: 3 in, 1 out]
        n309 = call "IMAQ Create"("Image Name"="GUIdevice 9", "Image Type"=w718) -> ("New Image"=→"image::9":T5)  [unwired: 3 in, 1 out]
        n310 = call "IMAQ Create"("Image Name"="GUIdevice 10", "Image Type"=w718) -> ("New Image"=→"image::10":T5)  [unwired: 3 in, 1 out]
        n311 = call "IMAQ Create"("Image Name"="GUIdevice 6", "Image Type"=w718) -> ("New Image"=→"image::6":T5)  [unwired: 3 in, 1 out]
        n312 = call "IMAQ Create"("Image Name"="GUIdevice 7", "Image Type"=w718) -> ("New Image"=→"image::7":T5)  [unwired: 3 in, 1 out]
        n313 = call "IMAQ Create"("Image Name"="GUIdevice 11", "Image Type"=w718) -> ("New Image"=→"image::11":T5)  [unwired: 3 in, 1 out]
        n314 = call "IMAQ Create"("Image Name"="GUIdevice 12", "Image Type"=w718) -> ("New Image"=→"image::12":T5)  [unwired: 3 in, 1 out]
        n315 = call "IMAQ Create"("Image Name"="GUIdevice 2") -> ("New Image"=→"image::2":T5)  [unwired: 4 in, 1 out]
        n316 = call "IMAQ Create"("Image Name"="GUIdevice 4", "Image Type"=w718) -> ("New Image"=→"image::4":T5)  [unwired: 3 in, 1 out]
        n317 = call "IMAQ Create"("Image Name"="GUIdevice 1", "Image Type"=w718) -> ("New Image"=→"image::1":T5)  [unwired: 3 in, 1 out]
        n318 = call "IMAQ Create"("Image Name"="GUIdevice 3", "Image Type"=w718) -> ("New Image"=→"image::3":T5)  [unwired: 3 in, 1 out]
        n319 = call "IMAQ Create"("Image Name"="GUIdevice 5", "Image Type"=w718) -> ("New Image"=→"image::5":T5)  [unwired: 3 in, 1 out]
        n320 = call <vilib>:"Add State(s) to Queue__jki_lib_state_machine.vi"("State(s) in (\"\")"=w746) -> ("States Out"=w745:string)  [unwired: 14 in]
      }
      frame "StartSuperGUI" {
        # "create stop queue for supergui and its clones"
        # "can make an icon"
        # "x100 abort will be dependent on caller VI\nx80 abort will be independent of caller vi, this will abort vi when labview is closed."
        # "Initialize the User Interface, here.\n(this is called automatically, by the Macro: Init)"
        n321 = vi-ref "GUI_Master_subvi_reentrant_queues.vi"() -> (w755:refnum<vi>)
        n322 = call "supergui create stop queue.vi"() -> ("STOP Queue out"=w756:refnum<queue>)  [unwired: 11 in]
        n323 = control-ref of="This Application"() -> (w759:refnum<vi>)
        n324 = property class="VI"(reference=w755) -> ("Path"=w754:path)  [unwired: 1 in, 2 out]
        n325 = control-ref of="This VI"() -> (w758:refnum<vi>)
        n326 = Create User Event(user event datatype=T25 {"EventEnum"=enum."new data", "Device name"="Device name"} ("New Event"), error in=w750) -> (user event=w760:refnum<user-event>, error out=w761:errorcluster)
        "tcp data event 2" <- w760
        n327 = Current VI's Menubar() -> (w757:refnum<k9>)
        n328 = register-events(w760) -> ()  [unwired: 2 in, 2 out]
        n329 = Open VI Reference(type specifier VI Refnum (for type only)=refnum<vi> refnum, vi path=w754, options=256, error in (no error)=w750) -> (vi reference=w765:refnum<vi>, error out=w764:errorcluster)  [unwired: 2 in]
        n330 = call <vilib>:"Add State(s) to Queue__jki_lib_state_machine.vi"("State(s) in (\"\")"=w767) -> ("States Out"=w766:string)  [unwired: 14 in]
        n331 = call-by-ref "Start Asynchronous Call"(reference=w765, error in=w764, "STOP Queue in"=w756, "This Application"=w759, 8:"error in (no error)"=w761, "tcp data event"=w760, "Caller menu reference"=w757, "Caller VI ref"=w758) -> (reference out=w753:refnum<vi>, error out=w749:errorcluster)  [unwired: 5 in, 1 out]
        n332 = Bundle By Name(cluster=w752, "Supergui.SuperGUI ref"=w753, "Supergui.STOP queue"=w756) -> (w751:T31)
      }
      frame "Device Ini" {
        n333 = Empty String/Path?(string/path=w773) -> (empty?=w790:bool)
        n334 = flat-sequence {
          tunnel: w794 -> [w797]
          tunnel: [w797] -> w768
          tunnel: w789 -> [w796]
          tunnel: w768 -> [w802]
          tunnel: [w800] -> w776
          frame #0 {
            # "check"
            n335 = Wait (ms)(milliseconds to wait=w796) -> ()  [unwired: 1 out]
          }
          frame #1 {
            # "check if cam images are new"
            n336 = local read "cam means"() -> (w798:sgl[])
            n337 = for {
              tunnel: w802 -> [w805] mode=indexing
              shift-right: [w810] -> w800
              shift-left: string[] [] -> [w811]
              tunnel: [w804] -> w799 mode=indexing
              shift-right: [w808] -> _
              shift-left: w798 -> [w808]
              i -> [w809]
              n338 = call "IMAQ Histograph"("Image"=w805) -> ("error out"=w803:errorcluster, "Mean Value"=w804:sgl)  [unwired: 7 in, 2 out]
              n339 = Index Array(array=w808, index=w809) -> (element=w807:sgl)
              n340 = call <vilib>:"Clear Errors.vi"("error in (no error)"=w803) -> ()  [unwired: 5 in, 2 out]
              n341 = Equal?(x=w804, y=w807) -> (x = y?=w806:bool)
              n342 = case shown="False" w806 {
                tunnel: w811 -> [w814 w815]
                tunnel: [w813 w815] -> w810
                tunnel: w805 -> [w812 _]
                frame False {
                  n343 = Build Array (concatenate)(w814, w812) -> (w813:string[])
                }
                frame True {
                }
              }
            }
            "cam means" <- w799
          }
        }
        n344 = case shown="False" w790 {
          tunnel: w773 -> [w851 _]
          tunnel: [w850 0] -> w789
          frame False {
            n345 = Decimal String To Number(string=w851) -> (number=w850:i32)  [unwired: 2 in, 1 out]
          }
          frame True {
          }
        }
        n346 = Unbundle By Name(w788) -> ("active cams"=w781:string[])
        n347 = Equal?(x=w773, y="T") -> (x = y?=w771:bool)
        n348 = Equal?(x=w781, y=w776) -> (x = y?=w787:bool[])
        n349 = Empty Array?(array=w781) -> (empty?=w786:bool)
        n350 = Not(x=w786) -> (.not. x?=w785:bool)
        n351 = Build Array (concatenate)(w787, w785) -> (w784:bool[])
        n352 = Array Size(array=w776) -> (size(s)=w780:i32)
        n353 = Array Size(array=w781) -> (size(s)=w779:i32)
        n354 = And Array Elements(Boolean array=w784) -> (logical AND=w777:bool)
        n355 = Equal?(x=w780, y=w779) -> (x = y?=w778:bool)
        n356 = And(x=w778, y=w777) -> (x .and. y?=w775:bool)
        n357 = Not(x=w775) -> (.not. x?=w772:bool)
        n358 = Or(x=w772, y=w771) -> (x .or. y?=w770:bool)
        n359 = call <vilib>:"Add State(s) to Queue__jki_lib_state_machine.vi"("State(s) in (\"\")"=w795) -> ("States Out"=w783:string)  [unwired: 14 in]
        n360 = case shown="True" w770 {
          tunnel: [w818 w833] -> w793
          tunnel: w792 -> [w817 w832]
          tunnel: [w817 w832] -> w791
          tunnel: w788 -> [w818 w829]
          tunnel: w776 -> [_ w822]
          tunnel: w783 -> [w816 w820]
          tunnel: [w816 w825] -> w782
          frame False {
          }
          frame True {
            # "#todo check repercussion of not loading config here"
            # "# active cams changed, perform configuration"
            n361 = local write "#imgs avd so far"(0.0 ("Numeric")) -> ()
            n362 = property on="active CCDs" class="LstBox (strict)"("Item Names"=w822) -> ()  [unwired: 2 in, 2 out]
            n363 = Bundle By Name(cluster=w829, "active cams"=w822) -> (w821:T31)
            n364 = Array Size(array=w822) -> (size(s)=w839:i32)
            n365 = Initialize Array(0.0 ("element"), w839, 0 ("dimension size")) -> (w834:dbl[][])
            n366 = Unbundle By Name(w821) -> ("img to avg"=w828:i32)
            n367 = Initialize Array(0.0 ("element"), 12 ("dimension size"), w828) -> (w827:dbl[][])
            n368 = for {
              N: 1 -> [_]
              shift-right: [w844] -> w837
              shift-left: timestamp[][] [] ("Time") -> [w846]
              n369 = for {
                N: 12 -> [_]
                tunnel: w846 -> [w849] mode=indexing
                tunnel: [w847] -> w844 mode=indexing
                n370 = Get Date/Time In Seconds() -> (seconds since 1Jan1904=w848:timestamp)
                n371 = Build Array (concatenate)(w849, w848) -> (w847:timestamp[])
              }
            }
            n372 = Bundle By Name(cluster=w821, "Offset X stats"=w834, "Offset Y stats"=w834, "Centroid X"=w827, "Centroid Y"=w827, "Mean Centroid X"=w834, "Mean Centroid Y"=w834, "Offset X"=w834, "Offset Y"=w834, "Size"=w827, "Mean Size"=w834, "Motor X"=w834, "Motor Y"=w834) -> (w833:T31)
            n373 = disable-structure shown="Enabled" {
              disable-tunnel: [w841 _] -> w824
              frame Enabled {
                n374 = property on="config path" class="Str"() -> ("Value"=w842:string)  [unwired: 2 in, 2 out]
                n375 = call <vilib>:"Build State String with Arguments__jki_lib_state_machine.vi"("Arguments (\"\")"=w842, "State"="Load Config" ("State(s) in Front (\"\")")) -> ("State with Arguments"=w841:string)  [unwired: 4 in]
              }
              frame Disabled {
              }
            }
            n376 = property on="Time" class="Arr (strict)"("Value"=w837) -> ()  [unwired: 2 in, 2 out]
            n377 = call <vilib>:"Add State(s) to Queue__jki_lib_state_machine.vi"("State(s) in (\"\")"=w820, "State(s) at Back (\"\")"="Move Config\nMotor Config\nDetection Config\nactive\nCenter" ("State(s) in Front (\"\")")) -> ("States Out"=w826:string)  [unwired: 13 in]
            n378 = call <vilib>:"Add State(s) to Queue__jki_lib_state_machine.vi"("State(s) in (\"\")"=w826, "State(s) at Back (\"\")"=w824) -> ("States Out"=w825:string)  [unwired: 13 in]
            "name array" <- w822
          }
        }
      }
      frame "Save Config" {
        w860 = T38 {"Camera names"=[], "Motor aliases x"=[], "Motor aliases y"=[], "detection para"=[], "thresholds"=[], "move properties"=[]}  # BP Configuration
        n379 = property on="Save Config" class="Bool (strict)"("Value"=FALSE ("Save Config")) -> ()  [unwired: 2 in, 2 out]
        n380 = local read "Cameras and motors"() -> (w855:T4)
        n381 = property on="Motor Alias X" class="Ring (strict)"() -> ("Strings []"=w856:string[])  [unwired: 2 in, 2 out]
        n382 = call "File Dialog"("pattern (all files)"="*.cfg", "pattern label"="config") -> ("selected path"=w865:path)  [unwired: 10 in, 3 out]
        n383 = for {
          tunnel: [w878] -> w859 mode=indexing
          tunnel: [w874] -> w858 mode=indexing
          tunnel: w856 -> [w876]
          tunnel: w855 -> [w879] mode=indexing
          tunnel: [w873] -> w853 mode=indexing
          n384 = Unbundle By Name(w879) -> ("Camera"=w873:string, "Motor Alias X"=w877:u16, "Motor Alias Y"=w875:u16)
          n385 = Index Array(array=w876, index=w875) -> (element=w874:string)
          n386 = Index Array(array=w876, index=w877) -> (element=w878:string)
        }
        n387 = Unbundle By Name(w870) -> ("move properties"=w863:T30[], "detection para"=w862:T7[], "thresholds"=w861:cluster{"Lower value":sgl, "Upper value":sgl}[])
        n388 = Bundle By Name(cluster=w860, "Camera names"=w853, "move properties"=w863, "detection para"=w862, "thresholds"=w861, "Motor aliases x"=w859, "Motor aliases y"=w858) -> (w857:T38)
        n389 = disable-structure shown="Enabled" {
          disable-tunnel: w869 -> [w883 w891]
          disable-tunnel: [w882 w890] -> w868
          disable-tunnel: w865 -> [w881 w889]
          disable-tunnel: w857 -> [w880 w892]
          frame Disabled {
            n390 = Open/Create/Replace File(file path (use dialog)=w881, error in=w883, operation (0:open)=T26."replace or create with confirmation") -> (refnum out=w885:refnum<file>, error out=w886:errorcluster)  [unwired: 3 in, 1 out]
            n391 = Write to Binary File(file (use dialog)=w885, data=w880, error in=w886) -> (refnum out=w888:refnum<file>, error out=w887:errorcluster)  [unwired: 3 in, 1 out]
            n392 = Close File(refnum=w888, error in=w887) -> (error out=w882:errorcluster)  [unwired: 1 out]
          }
          frame Enabled {
            n393 = call <userlib>:"MGI Write Anything.vi"("Error In"=w891, "Anything"=w892, "Path (dialog)"=w889) -> ("Error Out"=w890:errorcluster)  [unwired: 6 in, 2 out]
          }
        }
        n394 = call <vilib>:"Add State(s) to Queue__jki_lib_state_machine.vi"("State(s) in (\"\")"=w872) -> ("States Out"=w871:string)  [unwired: 14 in]
      }
      frame "active" {
        # "Your code here.\n(You can make a copy of, or modify, this frame)"
        n395 = Empty String/Path?(string/path=w906) -> (empty?=w905:bool)
        n396 = Unbundle By Name(w902) -> ("dev var alias arrays.dev variable alias Motors X"=w899:string[][], "dev var alias arrays.dev variable alias Motors Y"=w895:string[][])
        n397 = Unbundle By Name(w902) -> ("move properties"=w916:T30[], "detection para"=w912:T7[])  [unwired: 1 out]
        n398 = call-poly <userlib>:"Filter 1D Array__ogtk.vi"("items to filter"=w906, "array"=w914) -> ("filtered item indices"=w917:i32[])  [unwired: 4 in, 1 out]
        n399 = Index Array(array=w917) -> (element=w903:i32)  [unwired: 1 in]
        n400 = Select(t=0, s=w905, f=w903) -> (s? t:f=w894:i32)
        n401 = Index Array(array=w916, index=w894) -> (element=w915:T30)
        n402 = Index Array(array=w912, index=w894) -> (element=w911:T7)
        n403 = call "Beampointing get set motor position.vi"("Active CCD"=w894, "get or set"=enum16{"get", "set"}."get", "dev variable alias Motors X"=w895) -> ("Actual Position"=w893:dbl)  [unwired: 8 in]
        n404 = call "Beampointing get set motor position.vi"("Active CCD"=w894, "get or set"=enum16{"get", "set"}."get", "dev variable alias Motors X"=w899) -> ("Actual Position"=w897:dbl)  [unwired: 8 in]
        n405 = property on="move config" class="Clust (strict)"(error in=w909, "Value"=w915) -> (error out=w907:errorcluster)  [unwired: 1 in, 1 out]
        n406 = property on="beam detection para" class="Clust (strict)"(error in=w907, "Value"=w911) -> (error out=w908:errorcluster)  [unwired: 1 in, 1 out]
        n407 = call <vilib>:"Add State(s) to Queue__jki_lib_state_machine.vi"("State(s) in (\"\")"=w919) -> ("States Out"=w918:string)  [unwired: 14 in]
        n408 = Bundle By Name(cluster=w902, "active ccd"=w894) -> (w913:T31)
        n409 = property on="Position 1" class="DigNum (strict)"(error in=w908, "Value"=w897) -> (error out=w901:errorcluster)  [unwired: 1 in, 1 out]
        n410 = property on="Position 2" class="DigNum (strict)"(error in=w901, "Value"=w893) -> (error out=w910:errorcluster)  [unwired: 1 in, 1 out]
      }
      frame "Detection Config" {
        # "Your code here.\n(You can make a copy of, or modify, this frame)"
        n411 = Unbundle By Name(w925) -> ("detection para"=w921:T7[], "active ccd"=w926:i32)
        n412 = Replace Array Subset(array=w921, new element="beam detection para", index=w926) -> (w922:T7[])
        n413 = Bundle By Name(cluster=w925, "detection para"=w922) -> (w924:T31)
        n414 = call <vilib>:"Add State(s) to Queue__jki_lib_state_machine.vi"("State(s) in (\"\")"=w929) -> ("States Out"=w928:string)  [unwired: 14 in]
      }
      frame "Motor Config" {
        n415 = for {
          tunnel: w936 -> [w954]
          tunnel: "Cameras and motors" -> [w953] mode=indexing
          tunnel: [w941] -> w934 mode=indexing
          tunnel: [w946] -> w933 mode=indexing
          tunnel: [w944] -> w931 mode=indexing
          tunnel: [w942] -> w930 mode=indexing
          n416 = Unbundle By Name(w954) -> ("dev var alias arrays.dev variable alias"=w950:string[][])
          n417 = Index Array(array=w950, index (col)=2 ("disabled index (col)")) -> (element=w949:string[])  [unwired: 1 in]
          n418 = Unbundle By Name(w953) -> ("Motor Alias X"=w958:u16, "Motor Alias Y"=w948:u16)
          n419 = property on="Motor Alias X" class="Ring (strict)"() -> ("Strings []"=w947:string[])  [unwired: 2 in, 2 out]
          n420 = Index Array(array=w947, index=w958) -> (element=w957:string)
          n421 = Search 1D Array(1D array=w949, element=w957) -> (index of element=w956:i32)  [unwired: 1 in]
          n422 = Index Array(array=w950, index (row)=w956) -> (element=w941:string[])  [unwired: 1 in]
          n423 = Index Array(array=w947, index=w948) -> (element=w951:string)
          n424 = Search 1D Array(1D array=w949, element=w951) -> (index of element=w952:i32)  [unwired: 1 in]
          n425 = Index Array(array=w950, index (row)=w952) -> (element=w946:string[])  [unwired: 1 in]
          n426 = call "get set udp value from dev var alias array.vi"("get or set"=enum16{"get", "set"}."get", "dev variable alias Motors X"=w946) -> ("Numeric"=w944:dbl)  [unwired: 9 in]
          n427 = call "get set udp value from dev var alias array.vi"("get or set"=enum16{"get", "set"}."get", "dev variable alias Motors X"=w941) -> ("Numeric"=w942:dbl)  [unwired: 9 in]
        }
        n428 = call <vilib>:"Add State(s) to Queue__jki_lib_state_machine.vi"("State(s) in (\"\")"=w940) -> ("States Out"=w939:string)  [unwired: 14 in]
        n429 = Bundle By Name(cluster=w936, "dev var alias arrays.dev variable alias Motors X"=w934, "dev var alias arrays.dev variable alias Motors Y"=w933, "Motor positions.Positions x"=w930, "Motor positions.Positions y"=w931) -> (w937:T31)
      }
      frame "Move Config" {
        # "Your code here.\n(You can make a copy of, or modify, this frame)"
        n430 = Unbundle By Name(w961) -> ("move properties"=w965:T30[], "active ccd"=w964:i32)
        n431 = Replace Array Subset(array=w965, new element="move config", index=w964) -> (w962:T30[])
        n432 = Bundle By Name(cluster=w961, "move properties"=w962) -> (w960:T31)
        n433 = call <vilib>:"Add State(s) to Queue__jki_lib_state_machine.vi"("State(s) in (\"\")"=w968) -> ("States Out"=w967:string)  [unwired: 14 in]
      }
      frame "----------Centroid & Move----------" {
        # "Template Separator\n(You can make a copy of, or modify, this frame)"
        n434 = call <vilib>:"Add State(s) to Queue__jki_lib_state_machine.vi"("State(s) in (\"\")"=w973) -> ("States Out"=w972:string)  [unwired: 14 in]
      }
      frame "detected" {
        n435 = Unbundle By Name(w984) -> ("Offset X"=w1016:dbl[][], "Offset Y"=w1015:dbl[][], "Size"=w1014:dbl[][], "Mean Size"=w1013:dbl[][], "Time"=w1010:timestamp[][], "Motor X"=w993:dbl[][], "Motor positions"=w992:T32, "Motor Y"=w991:dbl[][])  [unwired: 1 out]
        n436 = Spreadsheet String To Array(format string="%s", spreadsheet string=w996, array type (2D Dbl)=string[] []) -> (array=w987:string[])  [unwired: 1 in]
        n437 = for {
          tunnel: w988 -> [w1028] mode=indexing
          tunnel: w987 -> [w1027]
          tunnel: [w1026] -> w986 mode=indexing
          n438 = for {
            tunnel: w1028 -> [w1031]
            tunnel: [w1030] -> w1025 mode=indexing
            tunnel: w1027 -> [w1029] mode=indexing
            n439 = Equal?(x=w1031, y=w1029) -> (x = y?=w1030:bool)
          }
          n440 = Or Array Elements(Boolean array=w1025) -> (logical OR=w1026:bool)
        }
        n441 = local read "Cameras and motors"() -> (w974:T4)
        n442 = Unbundle By Name(w984) -> ("Mean Centroid X"=w1019:dbl[][], "Mean Centroid Y"=w1018:dbl[][], "Centroid X"=w1021:dbl[][], "Centroid Y"=w1020:dbl[][])
        n443 = call <vilib>:"Add State(s) to Queue__jki_lib_state_machine.vi"("State(s) in (\"\")"=w995) -> ("States Out"=w994:string)  [unwired: 14 in]
        n444 = for {
          tunnel: w1021 -> [w1081]
          tunnel: w1020 -> [w1080]
          tunnel: w1019 -> [w1079]
          tunnel: w1018 -> [w1078]
          tunnel: [w1077] -> w1007 mode=indexing
          tunnel: [w1076] -> w1017 mode=indexing
          tunnel: w1016 -> [w1075]
          tunnel: w1015 -> [w1074]
          tunnel: [w1073] -> w985 mode=indexing
          tunnel: [w1072] -> w1008 mode=indexing
          tunnel: w1014 -> [w1071]
          tunnel: w1013 -> [w1070]
          tunnel: [w1069] -> w1012 mode=indexing
          tunnel: w1010 -> [w1068]
          tunnel: [w1067] -> w1009 mode=indexing
          tunnel: w993 -> [w1064]
          tunnel: w992 -> [w1037]
          tunnel: w991 -> [w1063]
          tunnel: [w1043] -> w990 mode=indexing
          tunnel: [w1042] -> w989 mode=indexing
          tunnel: w986 -> [w1041]
          tunnel: w975 -> [w1039]
          tunnel: w974 -> [_] mode=indexing
          i -> [w1033]
          n445 = Index Array(array=w1039, index=w1033) -> (element=w1038:T18)
          n446 = Unbundle By Name(w1037) -> ("Positions x"=w1036:dbl[], "Positions y"=w1034:dbl[])
          n447 = Unbundle By Name(w1038) -> ("Target.X::12"=w1047:refnum<vi>, "Target.Y::12"=w1046:refnum<vi>)
          n448 = Index Array(array=w1064, index (row)=w1033) -> (element=w1065:dbl[])  [unwired: 1 in]
          n449 = Index Array(array=w1036, index=w1033) -> (element=w1035:dbl)
          n450 = Index Array(array=w1063, index (row)=w1033) -> (element=w1066:dbl[])  [unwired: 1 in]
          n451 = Index Array(array=w1041, index=w1033) -> (element=w1040:bool)
          n452 = Index Array(array=w1079, index (row)=w1033) -> (element=w1059:dbl[])  [unwired: 1 in]
          n453 = Index Array(array=w1078, index (row)=w1033) -> (element=w1060:dbl[])  [unwired: 1 in]
          n454 = Index Array(array=w1081, index (row)=w1033) -> (element=w1062:dbl[])  [unwired: 1 in]
          n455 = Index Array(array=w1080, index (row)=w1033) -> (element=w1061:dbl[])  [unwired: 1 in]
          n456 = Index Array(array=w1075, index (row)=w1033) -> (element=w1055:dbl[])  [unwired: 1 in]
          n457 = Index Array(array=w1074, index (row)=w1033) -> (element=w1054:dbl[])  [unwired: 1 in]
          n458 = Index Array(array=w1071, index (row)=w1033) -> (element=w1052:dbl[])  [unwired: 1 in]
          n459 = Index Array(array=w1070, index (row)=w1033) -> (element=w1051:dbl[])  [unwired: 1 in]
          n460 = Index Array(array=w1068, index (row)=w1033) -> (element=w1048:timestamp[])  [unwired: 1 in]
          n461 = Index Array(array=w1034, index=w1033) -> (element=w1032:dbl)
          n462 = property class="DigNum (strict)"(reference=w1047) -> ("Value"=w1045:dbl)  [unwired: 1 in, 2 out]
          n463 = property class="DigNum (strict)"(reference=w1046) -> ("Value"=w1044:dbl)  [unwired: 1 in, 2 out]
          n464 = call <vilib>:"Std Deviation and Variance.vi"("X"=w1062) -> ("mean"=w1058:dbl)  [unwired: 1 in, 2 out]
          n465 = call <vilib>:"Std Deviation and Variance.vi"("X"=w1061) -> ("mean"=w1057:dbl)  [unwired: 1 in, 2 out]
          n466 = call <vilib>:"Std Deviation and Variance.vi"("X"=w1052) -> ("mean"=w1050:dbl)  [unwired: 1 in, 2 out]
          n467 = Get Date/Time In Seconds() -> (seconds since 1Jan1904=w1049:timestamp)
          n468 = Subtract(x=w1045, y=w1058) -> (x-y=w1056:dbl)
          n469 = Subtract(x=w1044, y=w1057) -> (x-y=w1053:dbl)
          n470 = case shown="True" w1040 {
            tunnel: [w1094 w1113] -> w1077
            tunnel: [w1082 w1112] -> w1076
            tunnel: [w1083 w1111] -> w1073
            tunnel: [w1084 w1110] -> w1072
            tunnel: [w1085 w1109] -> w1069
            tunnel: [w1086 w1108] -> w1067
            tunnel: w1060 -> [w1092 w1107]
            tunnel: w1059 -> [w1093 w1106]
            tunnel: w1058 -> [_ w1105]
            tunnel: w1057 -> [_ w1104]
            tunnel: w1056 -> [_ w1103]
            tunnel: w1055 -> [w1091 w1102]
            tunnel: w1054 -> [w1090 w1101]
            tunnel: w1053 -> [_ w1100]
            tunnel: w1051 -> [w1089 w1099]
            tunnel: w1050 -> [_ w1098]
            tunnel: w1049 -> [w1087 w1097]
            tunnel: w1048 -> [w1088 w1096]
            frame False {
              w1095 = 0.0
              n471 = Build Array (concatenate)(w1093, w1095) -> (w1094:dbl[])
              n472 = Build Array (concatenate)(w1092, w1095) -> (w1082:dbl[])
              n473 = Build Array (concatenate)(w1091, w1095) -> (w1083:dbl[])
              n474 = Build Array (concatenate)(w1090, w1095) -> (w1084:dbl[])
              n475 = Build Array (concatenate)(w1089, w1095) -> (w1085:dbl[])
              n476 = Build Array (concatenate)(w1088, w1087) -> (w1086:timestamp[])
            }
            frame True {
              n477 = Build Array (concatenate)(w1106, w1105) -> (w1113:dbl[])
              n478 = Build Array (concatenate)(w1107, w1104) -> (w1112:dbl[])
              n479 = Build Array (concatenate)(w1102, w1103) -> (w1111:dbl[])
              n480 = Build Array (concatenate)(w1101, w1100) -> (w1110:dbl[])
              n481 = Build Array (concatenate)(w1099, w1098) -> (w1109:dbl[])
              n482 = Build Array (concatenate)(w1096, w1097) -> (w1108:timestamp[])
            }
          }
          n483 = Build Array (concatenate)(w1065, w1035) -> (w1043:dbl[])
          n484 = Build Array (concatenate)(w1066, w1032) -> (w1042:dbl[])
        }
        n485 = local write "#imgs avd so far"(0.0 ("Numeric")) -> ()
        n486 = Array Size(array=w985) -> (size(s)=w1006:i32[])
        n487 = Index Array(array=w1006, index=1) -> (element=w1004:i32)
        "History Index" <- w1004
        n488 = call <vilib>:"Add State(s) to Queue__jki_lib_state_machine.vi"("State(s) in (\"\")"=w994, "State(s) at Back (\"\")"="Check Move\ntdms" ("State(s) at Back (\"\")")) -> ("States Out"=w998:string)  [unwired: 13 in]
        n489 = Unbundle By Name(w984) -> ("img to avg"=w981:i32)
        n490 = Initialize Array(0.0 ("element"), 12 ("dimension size"), w981) -> (w980:dbl[][])
        n491 = Greater?(x=w1004, y="History Size") -> (0:w1002:bool)
        n492 = Bundle By Name(cluster=w984, "Centroid X"=w980, "Centroid Y"=w980, "Mean Centroid X"=w1007, "Mean Centroid Y"=w1017, "Offset X"=w985, "Offset Y"=w1008, "Mean Size"=w1012, "Size"=w980, "Time"=w1009, "Motor X"=w990, "Motor Y"=w989) -> (w977:T31)
        n493 = Select(t="history" ("State(s) at Back (\"\")"), s=w1002, f="") -> (s? t:f=w999:string)
        n494 = call <vilib>:"Add State(s) to Queue__jki_lib_state_machine.vi"("State(s) in (\"\")"=w998, "State(s) at Back (\"\")"=w999) -> ("States Out"=w979:string)  [unwired: 13 in]
        n495 = call <vilib>:"Add State(s) to Queue__jki_lib_state_machine.vi"("State(s) in (\"\")"=w979) -> ("States Out"=w978:string)  [unwired: 14 in]
      }
      frame "Check Move" {
        n496 = Unbundle By Name(w1123) -> ("move properties"=w1133:T30[], "Mean Size"=w1132:dbl[][], "move properties"=w1131:T30[], "Offset X"=w1130:dbl[][], "Offset Y"=w1129:dbl[][], "active cams"=w1128:string[])
        n497 = Unbundle By Name(w1123) -> ("steps speed X"=w1122:dbl[], "steps speed Y"=w1121:dbl[])
        n498 = for {
          tunnel: w1131 -> [w1171]
          tunnel: w1130 -> [w1169]
          tunnel: w1129 -> [w1167]
          tunnel: w1132 -> [w1175]
          tunnel: [w1186] -> w1117 mode=indexing
          tunnel: [w1182] -> w1115 mode=indexing
          tunnel: w1128 -> [w1176] mode=indexing
          tunnel: [w1204] -> w1134 mode=indexing
          tunnel: [w1203] -> w1126 mode=indexing
          tunnel: w1133 -> [w1174]
          tunnel: [w1165] -> w1118 mode=indexing
          tunnel: [w1164] -> w1116 mode=indexing
          tunnel: "Speedmode" -> [w1179]
          tunnel: w1125 -> [w1177]
          shift-right: [w1157] -> w1120
          shift-left: w1122 -> [w1162]
          shift-right: [w1156] -> w1119
          shift-left: w1121 -> [w1161]
          n499 = call-poly <userlib>:"Filter 1D Array__ogtk.vi"("items to filter"=w1176, "array"=w1177) -> ("filtered item indices"=w1178:i32[])  [unwired: 4 in, 1 out]
          n500 = Index Array(array=w1178) -> (element=w1160:i32)  [unwired: 1 in]
          n501 = Index Array(array=w1174, index=w1160) -> (element=w1173:T30)
          n502 = Index Array(array=w1175, index (row)=w1160) -> (element=w1172:dbl[])  [unwired: 1 in]
          n503 = Index Array(array=w1171, index=w1160) -> (element=w1170:T30)
          n504 = Index Array(array=w1169, index (row)=w1160) -> (element=w1168:dbl[])  [unwired: 1 in]
          n505 = Index Array(array=w1167, index (row)=w1160) -> (element=w1166:dbl[])  [unwired: 1 in]
          n506 = Unbundle By Name(w1170) -> ("Tolerance [%]"=w1197)
          n507 = Reverse 1D Array(array=w1168) -> (reversed array=w1202:dbl[])
          n508 = Reverse 1D Array(array=w1166) -> (reversed array=w1201:dbl[])
          n509 = Reverse 1D Array(array=w1172) -> (reversed array=w1196:dbl[])
          n510 = Unbundle By Name(w1173) -> ("Stepsize"=w1155:dbl, "enable feedback"=w1185:bool)
          n511 = Index Array(array=w1202) -> (element=w1200:dbl)  [unwired: 1 in]
          n512 = Index Array(array=w1201) -> (element=w1199:dbl)  [unwired: 1 in]
          n513 = Index Array(array=w1196) -> (element=w1195:dbl)  [unwired: 1 in]
          n514 = Absolute Value(x=w1200) -> (abs(x)=w1163:dbl)
          n515 = Absolute Value(x=w1199) -> (abs(x)=w1181:dbl)
          n516 = Square Root(x=w1195) -> (sqrt(x)=w1194:dbl)
          n517 = Divide(x=w1197, y=100.0) -> (x/y=w1193:dbl)
          n518 = Multiply(x=w1194, y=w1193) -> (x*y=w1180:dbl)
          n519 = Not Equal To 0?(x=w1181) -> (x != 0?=w1183:bool)
          n520 = Not Equal To 0?(x=w1163) -> (x != 0?=w1188:bool)
          n521 = Greater Or Equal?(x=w1163, y=w1180) -> (x >= y?=w1187:bool)
          n522 = Greater Or Equal?(x=w1181, y=w1180) -> (x >= y?=w1184:bool)
          n523 = call "speedmode.vi"("offset X"=w1163, "offset Y"=w1181, "beamsize x tolerance"=w1180, "Speedmode @"=w1179, "step size"=w1155) -> ("steps speed Y"=w1158:dbl, "steps speed X"=w1159:dbl, "speedmode X"=w1165:bool, "speedmode Y"=w1164:bool)  [unwired: 3 in]
          n524 = Compound Arithmetic op=AND(w1185, w1188, w1187) -> (w1186:bool)
          n525 = Compound Arithmetic op=AND(w1185, w1184, w1183) -> (w1182:bool)
          n526 = Boolean To (0,1)(Boolean=w1182) -> (0, 1=w1189:i16)
          n527 = Multiply(x=w1189, y=w1181) -> (x*y=w1190:dbl)
          n528 = Boolean To (0,1)(Boolean=w1186) -> (0, 1=w1192:i16)
          n529 = Replace Array Subset(array=w1162, new element=w1159, index=w1160) -> (w1157:dbl[])
          n530 = Replace Array Subset(array=w1161, new element=w1158, index=w1160) -> (w1156:dbl[])
          n531 = Multiply(x=w1192, y=w1163) -> (x*y=w1191:dbl)
          n532 = Bundle(w1190, "GUIdevice 8"=w1176) -> (w1203:cluster{dbl, "GUIdevice 8":string})  [unwired: 1 in]
          n533 = Bundle(w1191, "GUIdevice 8"=w1176) -> (w1204:cluster{dbl, "GUIdevice 8":string})  [unwired: 1 in]
        }
        "required X" <- w1117
        "required Y" <- w1115
        "speedmode X" <- w1118
        "speedmode Y" <- w1116
        n534 = case shown="False" "Align" {
          tunnel: w1134 -> [w1210 w1215]
          tunnel: w1126 -> [w1209 w1212]
          tunnel: [w1208 w1214] -> w1137
          tunnel: [w1207 w1211] -> w1136
          frame False {
            n535 = Sort 1D Array(array=w1209) -> (sorted array=w1206:cluster{dbl, "GUIdevice 8":string}[])
            n536 = Sort 1D Array(array=w1210) -> (sorted array=w1205:cluster{dbl, "GUIdevice 8":string}[])
            n537 = Reverse 1D Array(array=w1206) -> (reversed array=w1207:cluster{dbl, "GUIdevice 8":string}[])
            n538 = Reverse 1D Array(array=w1205) -> (reversed array=w1208:cluster{dbl, "GUIdevice 8":string}[])
          }
          frame True {
            w1213 = cluster{dbl, "GUIdevice 8":string}[] [] ("Array")
            n539 = for {
              shift-right: [w1225] -> w1214
              shift-left: w1213 -> [w1227]
              tunnel: w1215 -> [w1226] mode=indexing
              n540 = Unbundle(w1226) -> (w1229:dbl)  [unwired: 1 out]
              n541 = Not Equal To 0?(x=w1229) -> (x != 0?=w1228:bool)
              n542 = case shown="True" w1228 {
                tunnel: w1227 -> [w1230 w1233]
                tunnel: w1226 -> [_ w1232]
                tunnel: [w1230 w1231] -> w1225
                frame False {
                }
                frame True {
                  n543 = Build Array (concatenate)(w1233, w1232) -> (w1231:cluster{dbl, "GUIdevice 8":string}[])
                }
              }
            }
            n544 = for {
              shift-right: [w1216] -> w1211
              shift-left: w1213 -> [w1218]
              tunnel: w1212 -> [w1217] mode=indexing
              n545 = Unbundle(w1217) -> (w1220:dbl)  [unwired: 1 out]
              n546 = Not Equal To 0?(x=w1220) -> (x != 0?=w1219:bool)
              n547 = case shown="True" w1219 {
                tunnel: w1218 -> [w1221 w1224]
                tunnel: w1217 -> [_ w1223]
                tunnel: [w1221 w1222] -> w1216
                frame False {
                }
                frame True {
                  n548 = Build Array (concatenate)(w1224, w1223) -> (w1222:cluster{dbl, "GUIdevice 8":string}[])
                }
              }
            }
          }
        }
        n549 = call <vilib>:"Add State(s) to Queue__jki_lib_state_machine.vi"("State(s) in (\"\")"=w1140) -> ("States Out"=w1139:string)  [unwired: 14 in]
        n550 = Bundle By Name(cluster=w1123, "speedmode X"=w1118, "speedmode Y"=w1116, "steps speed X"=w1120, "steps speed Y"=w1119) -> (w1124:T31)
        n551 = Index Array(array=w1136) -> (element=w1141:cluster{dbl, "GUIdevice 8":string})  [unwired: 1 in]
        n552 = Index Array(array=w1137) -> (element=w1142:cluster{dbl, "GUIdevice 8":string})  [unwired: 1 in]
        n553 = Empty Array?(array=w1136) -> (empty?=w1144:bool)
        n554 = Unbundle(w1142) -> (w1150:dbl)  [unwired: 1 out]
        n555 = Unbundle(w1141) -> (w1146:dbl)  [unwired: 1 out]
        n556 = Unbundle By Name(w1124) -> ("Feedback global"=w1151:bool)
        n557 = Empty Array?(array=w1137) -> (empty?=w1148:bool)
        n558 = property on="autodetect" class="Bool (strict)"("Value"=FALSE ("autodetect")) -> ()  [unwired: 2 in, 2 out]
        n559 = Equal To 0?(x=w1150) -> (x = 0?=w1149:bool)
        n560 = Equal To 0?(x=w1146) -> (x = 0?=w1145:bool)
        n561 = Or(x=w1149, y=w1148) -> (x .or. y?=w1147:bool)
        n562 = Or(x=w1145, y=w1144) -> (x .or. y?=w1143:bool)
        n563 = case shown="True" w1151 {
          tunnel: w1147 -> [_ w1252]
          tunnel: w1137 -> [_ w1251]
          tunnel: w1143 -> [_ w1249]
          tunnel: w1136 -> [_ w1248]
          tunnel: w1139 -> [w1234 w1247]
          tunnel: [w1234 w1246] -> w1152
          tunnel: w1118 -> [_ w1245]
          tunnel: w1117 -> [_ w1244]
          tunnel: w1116 -> [_ w1243]
          tunnel: w1115 -> [_ w1242]
          frame False {
          }
          frame True {
            n564 = case shown="False" w1252 {
              tunnel: w1251 -> [w1276 _]
              tunnel: w1247 -> [w1272 w1277]
              tunnel: [w1270 w1277] -> w1250
              frame False {
                n565 = Index Array(array=w1276) -> (element=w1275:cluster{dbl, "GUIdevice 8":string})  [unwired: 1 in]
                n566 = Unbundle By Name(w1275) -> ("GUIdevice 8"=w1274:string)
                n567 = call <vilib>:"Build State String with Arguments__jki_lib_state_machine.vi"("Arguments (\"\")"=w1274, "State"="Move X") -> ("State with Arguments"=w1271:string)  [unwired: 4 in]
                n568 = call <vilib>:"Add State(s) to Queue__jki_lib_state_machine.vi"("State(s) in (\"\")"=w1272, "State(s) at Back (\"\")"=w1271) -> ("States Out"=w1270:string)  [unwired: 13 in]
              }
              frame True {
              }
            }
            n569 = case shown="False" w1249 {
              tunnel: w1248 -> [w1268 _]
              tunnel: w1250 -> [w1264 w1269]
              tunnel: [w1262 w1269] -> w1246
              frame False {
                n570 = Index Array(array=w1268) -> (element=w1267:cluster{dbl, "GUIdevice 8":string})  [unwired: 1 in]
                n571 = Unbundle By Name(w1267) -> ("GUIdevice 8"=w1266:string)
                n572 = call <vilib>:"Build State String with Arguments__jki_lib_state_machine.vi"("Arguments (\"\")"=w1266, "State"="Move Y") -> ("State with Arguments"=w1263:string)  [unwired: 4 in]
                n573 = call <vilib>:"Add State(s) to Queue__jki_lib_state_machine.vi"("State(s) in (\"\")"=w1264, "State(s) at Back (\"\")"=w1263) -> ("States Out"=w1262:string)  [unwired: 13 in]
              }
              frame True {
              }
            }
            n574 = for {
              tunnel: w1245 -> [w1261] mode=indexing
              tunnel: w1244 -> [w1260] mode=indexing
              tunnel: [w1259] -> w1241 mode=indexing
              n575 = And(x=w1261, y=w1260) -> (x .and. y?=w1259:bool)
            }
            n576 = for {
              tunnel: w1243 -> [w1258] mode=indexing
              tunnel: w1242 -> [w1257] mode=indexing
              tunnel: [w1256] -> w1240 mode=indexing
              n577 = And(x=w1258, y=w1257) -> (x .and. y?=w1256:bool)
            }
            n578 = Or Array Elements(Boolean array=w1241) -> (logical OR=w1239:bool)
            n579 = Or Array Elements(Boolean array=w1240) -> (logical OR=w1238:bool)
            n580 = Or(x=w1239, y=w1238) -> (x .or. y?=w1237:bool)
            n581 = property on="alarms" class="Bool (strict)"() -> ("Value"=w1236:bool)  [unwired: 2 in, 2 out]
            n582 = And(x=w1236, y=w1237) -> (x .and. y?=w1235:bool)
            n583 = case shown="True" w1235 {
              frame False {
              }
              frame True {
                n584 = call <vilib>:"Beep.vi"("use system alert? (T)"=FALSE, "duration (msec)"=u32 750, "frequency (Hz)"=u32 750) -> ()  [unwired: 9 in]
              }
            }
          }
        }
        n585 = call <vilib>:"Add State(s) to Queue__jki_lib_state_machine.vi"("State(s) in (\"\")"=w1139, "State(s) at Back (\"\")"=w1152) -> ("States Out"=w1154:string)  [unwired: 13 in]
      }
      frame "Move X" {
        # "Your code here.\n(You can make a copy of, or modify, this frame)"
        n586 = Unbundle By Name(w1284) -> ("Offset X"=w1302:dbl[][])
        n587 = call-poly <userlib>:"Filter 1D Array__ogtk.vi"("items to filter"=w1292, "array"=w1304) -> ("filtered item indices"=w1295:i32[])  [unwired: 4 in, 1 out]
        n588 = Unbundle By Name(w1284) -> ("dev var alias arrays.dev variable alias Motors X"=w1286:string[][])
        n589 = Unbundle By Name(w1284) -> ("move properties"=w1291:T30[])
        n590 = for {
          tunnel: w1295 -> [w1309] mode=indexing
          tunnel: w1291 -> [w1313]
          shift-right: [w1308] -> w1293
          shift-left: i32[] [] ("filtered item indices") -> [w1311]
          n591 = Index Array(array=w1313, index=w1309) -> (element=w1312:T30)
          n592 = Unbundle By Name(w1312) -> ("enable feedback"=w1310:bool)
          n593 = case shown="True" w1310 {
            tunnel: w1311 -> [w1314 w1317]
            tunnel: w1309 -> [_ w1316]
            tunnel: [w1314 w1315] -> w1308
            frame False {
            }
            frame True {
              n594 = Build Array (concatenate)(w1317, w1316) -> (w1315:i32[])
            }
          }
        }
        n595 = Index Array(array=w1293) -> (element=w1282:i32)  [unwired: 1 in]
        n596 = call "Beampointing get set motor position.vi"("Active CCD"=w1282, "get or set"=enum16{"get", "set"}."get", "dev variable alias Motors X"=w1286) -> ("Actual Position"=w1285:dbl)  [unwired: 8 in]
        n597 = Index Array(array=w1302, index (row)=w1282) -> (element=w1301:dbl[])  [unwired: 1 in]
        n598 = Reverse 1D Array(array=w1301) -> (reversed array=w1300:dbl[])
        n599 = Index Array(array=w1300) -> (element=w1299:dbl)  [unwired: 1 in]
        n600 = Index Array(array=w1291, index=w1282) -> (element=w1303:T30)
        n601 = Unbundle By Name(w1303) -> ("Invert Direction X"=w1297:bool, "enable feedback"=w1296:bool)  [unwired: 1 out]
        n602 = Greater Or Equal To 0?(x=w1299) -> (x >= 0?=w1298:bool)
        n603 = Unbundle By Name(w1284) -> ("steps speed X"=w1290:dbl[])  [unwired: 1 out]
        n604 = Index Array(array=w1290, index=w1282) -> (element=w1289:dbl)
        n605 = case shown="True" w1296 {
          tunnel: w1298 -> [_ w1327]
          tunnel: w1289 -> [_ w1326]
          tunnel: w1297 -> [_ w1325]
          tunnel: w1286 -> [_ w1323]
          tunnel: w1282 -> [_ w1322]
          tunnel: w1285 -> [w1318 w1320]
          tunnel: [w1318 w1319] -> w1280
          frame False {
          }
          frame True {
            n606 = case shown="False" w1327 {
              tunnel: w1325 -> [w1331 w1341]
              tunnel: w1326 -> [w1330 w1340]
              tunnel: [w1329 w1339] -> w1321
              tunnel: w1320 -> [w1328 w1338]
              frame True {
                n607 = case shown="True" w1331 {
                  tunnel: w1328 -> [w1334 w1337]
                  tunnel: w1330 -> [w1333 w1336]
                  tunnel: [w1332 w1335] -> w1329
                  frame False {
                    n608 = Add(x=w1334, y=w1333) -> (x+y=w1332:dbl)
                  }
                  frame True {
                    n609 = Subtract(x=w1337, y=w1336) -> (x-y=w1335:dbl)
                  }
                }
              }
              frame False {
                n610 = case shown="False" w1341 {
                  tunnel: w1338 -> [w1344 w1347]
                  tunnel: w1340 -> [w1343 w1346]
                  tunnel: [w1342 w1345] -> w1339
                  frame False {
                    n611 = Subtract(x=w1344, y=w1343) -> (x-y=w1342:dbl)
                  }
                  frame True {
                    n612 = Add(x=w1347, y=w1346) -> (x+y=w1345:dbl)
                  }
                }
              }
            }
            n613 = call "Beampointing get set motor position.vi"("Active CCD"=w1322, "Set position"=w1321, "get or set"=enum16{"get", "set"}."set", "dev variable alias Motors X"=w1323) -> ("Actual Position"=w1319:dbl)  [unwired: 7 in]
          }
        }
        n614 = call <vilib>:"Build State String with Arguments__jki_lib_state_machine.vi"("Arguments (\"\")"=w1292, "State"="Wait" ("State(s) in Front (\"\")")) -> ()  [unwired: 4 in, 1 out]
        n615 = call <vilib>:"Add State(s) to Queue__jki_lib_state_machine.vi"("State(s) in (\"\")"=w1307) -> ("States Out"=w1306:string)  [unwired: 14 in]
        n616 = Unbundle By Name(w1284) -> ("Motor positions.Positions x"=w1283:dbl[])
        n617 = Replace Array Subset(array=w1283, new element=w1280, index=w1282) -> (w1281:dbl[])
        n618 = Bundle By Name(cluster=w1284, "Motor positions.Positions x"=w1281) -> (w1279:T31)
        "Moving X" <- w1292
      }
      frame "ManMove X" {
        # "Your code here.\n(You can make a copy of, or modify, this frame)"
        n619 = Unbundle By Name(w1351) -> ("dev var alias arrays.dev variable alias Motors X"=w1355:string[][])
        n620 = Unbundle By Name(w1351) -> ("move properties"=w1365:T30[], "active ccd"=w1348:i32, "active cams"=w1363:string[])  [unwired: 1 out]
        n621 = Index Array(array=w1363, index=w1348) -> (element=w1361:string)
        n622 = call "Beampointing get set motor position.vi"("Active CCD"=w1348, "get or set"=enum16{"get", "set"}."get", "dev variable alias Motors X"=w1355) -> ("Actual Position"=w1356:dbl)  [unwired: 8 in]
        n623 = Index Array(array=w1365, index=w1348) -> (element=w1367:T30)
        n624 = Unbundle By Name(w1367) -> ("Invert Direction X"=w1366:bool)
        n625 = call <vilib>:"Build State String with Arguments__jki_lib_state_machine.vi"("Arguments (\"\")"=w1361, "State"="Wait" ("State(s) in Front (\"\")")) -> ()  [unwired: 4 in, 1 out]
        n626 = call <vilib>:"Add State(s) to Queue__jki_lib_state_machine.vi"("State(s) in (\"\")"=w1370) -> ("States Out"=w1369:string)  [unwired: 14 in]
        n627 = case shown="\"Left\", Default" w1360 {
          tunnel: w1366 -> [w1374 w1384]
          tunnel: "StepSize" -> [w1373 w1383]
          tunnel: w1356 -> [w1372 w1382]
          tunnel: [w1371 w1381] -> w1354
          frame "Right" {
            n628 = case shown="False" w1374 {
              tunnel: w1372 -> [w1377 w1380]
              tunnel: w1373 -> [w1376 w1379]
              tunnel: [w1375 w1378] -> w1371
              frame False {
                n629 = Add(x=w1377, y=w1376) -> (x+y=w1375:dbl)
              }
              frame True {
                n630 = Subtract(x=w1380, y=w1379) -> (x-y=w1378:dbl)
              }
            }
          }
          frame "Left", Default {
            n631 = case shown="True" w1384 {
              tunnel: w1382 -> [w1387 w1390]
              tunnel: w1383 -> [w1386 w1389]
              tunnel: [w1385 w1388] -> w1381
              frame False {
                n632 = Subtract(x=w1387, y=w1386) -> (x-y=w1385:dbl)
              }
              frame True {
                n633 = Add(x=w1390, y=w1389) -> (x+y=w1388:dbl)
              }
            }
          }
        }
        n634 = call "Beampointing get set motor position.vi"("Active CCD"=w1348, "Set position"=w1354, "get or set"=enum16{"get", "set"}."set", "dev variable alias Motors X"=w1355) -> ("Actual Position"=w1349:dbl)  [unwired: 7 in]
        n635 = Unbundle By Name(w1351) -> ("Motor positions.Positions x"=w1353:dbl[])
        n636 = Replace Array Subset(array=w1353, new element=w1349, index=w1348) -> (w1352:dbl[])
        n637 = Bundle By Name(cluster=w1351, "Motor positions.Positions x"=w1352) -> (w1350:T31)
      }
      frame "ManMove Y" {
        # "Your code here.\n(You can make a copy of, or modify, this frame)"
        n638 = Equal?(x=w1404, y="Down") -> ()  [unwired: 1 out]
        n639 = Unbundle By Name(w1393) -> ("active cams"=w1406:string[], "move properties"=w1410:T30[], "active ccd"=w1394:i32)
        n640 = Unbundle By Name(w1393) -> ("dev var alias arrays.dev variable alias Motors Y"=w1402:string[][])
        n641 = Index Array(array=w1406, index=w1394) -> (element=w1405:string)
        n642 = call "Beampointing get set motor position.vi"("Active CCD"=w1394, "get or set"=enum16{"get", "set"}."get", "dev variable alias Motors X"=w1402) -> ("Actual Position"=w1398:dbl)  [unwired: 8 in]
        n643 = Index Array(array=w1410, index=w1394) -> (element=w1411:T30)
        n644 = property on="StepSize" class="DigNum (strict)"() -> ("Value"=w1407:dbl)  [unwired: 2 in, 2 out]
        n645 = Unbundle By Name(w1411) -> ("Invert Direction Y"=w1408:bool)  [unwired: 1 out]
        n646 = call <vilib>:"Build State String with Arguments__jki_lib_state_machine.vi"("Arguments (\"\")"=w1405, "State"="Wait" ("State(s) in Front (\"\")")) -> ()  [unwired: 4 in, 1 out]
        n647 = case shown="\"Up\", Default" w1404 {
          tunnel: w1408 -> [w1418 w1428]
          tunnel: w1407 -> [w1417 w1427]
          tunnel: [w1416 w1425] -> w1399
          tunnel: w1398 -> [w1415 w1426]
          frame "Down" {
            n648 = case shown="False" w1418 {
              tunnel: w1415 -> [w1421 w1424]
              tunnel: w1417 -> [w1420 w1423]
              tunnel: [w1419 w1422] -> w1416
              frame False {
                n649 = Add(x=w1421, y=w1420) -> (x+y=w1419:dbl)
              }
              frame True {
                n650 = Subtract(x=w1424, y=w1423) -> (x-y=w1422:dbl)
              }
            }
          }
          frame "Up", Default {
            n651 = case shown="False" w1428 {
              tunnel: w1426 -> [w1431 w1434]
              tunnel: w1427 -> [w1430 w1433]
              tunnel: [w1429 w1432] -> w1425
              frame False {
                n652 = Subtract(x=w1431, y=w1430) -> (x-y=w1429:dbl)
              }
              frame True {
                n653 = Add(x=w1434, y=w1433) -> (x+y=w1432:dbl)
              }
            }
          }
        }
        n654 = call <vilib>:"Add State(s) to Queue__jki_lib_state_machine.vi"("State(s) in (\"\")"=w1414) -> ("States Out"=w1413:string)  [unwired: 14 in]
        n655 = call "Beampointing get set motor position.vi"("Active CCD"=w1394, "Set position"=w1399, "get or set"=enum16{"get", "set"}."set", "dev variable alias Motors X"=w1402) -> ("Actual Position"=w1395:dbl)  [unwired: 7 in]
        n656 = Unbundle By Name(w1393) -> ("Motor positions.Positions y"=w1397:dbl[])
        n657 = Replace Array Subset(array=w1397, new element=w1395, index=w1394) -> (w1396:dbl[])
        n658 = Bundle By Name(cluster=w1393, "Motor positions.Positions y"=w1396) -> (w1392:T31)
      }
      frame "Move Y" {
        # "Your code here.\n(You can make a copy of, or modify, this frame)"
        n659 = Unbundle By Name(w1439) -> ("dev var alias arrays.dev variable alias Motors Y"=w1442:string[][])
        n660 = Unbundle By Name(w1439) -> ("Offset Y"=w1462:dbl[][])
        n661 = call-poly <userlib>:"Filter 1D Array__ogtk.vi"("items to filter"=w1452, "array"=w1464) -> ("filtered item indices"=w1456:i32[])  [unwired: 4 in, 1 out]
        n662 = Unbundle By Name(w1439) -> ("move properties"=w1454:T30[])
        n663 = for {
          tunnel: w1456 -> [w1469] mode=indexing
          tunnel: w1454 -> [w1473]
          shift-right: [w1468] -> w1455
          shift-left: i32[] [] ("filtered item indices") -> [w1471]
          n664 = Index Array(array=w1473, index=w1469) -> (element=w1472:T30)
          n665 = Unbundle By Name(w1472) -> ("enable feedback"=w1470:bool)
          n666 = case shown="True" w1470 {
            tunnel: w1471 -> [w1474 w1477]
            tunnel: w1469 -> [_ w1476]
            tunnel: [w1474 w1475] -> w1468
            frame False {
            }
            frame True {
              n667 = Build Array (concatenate)(w1477, w1476) -> (w1475:i32[])
            }
          }
        }
        n668 = Index Array(array=w1455) -> (element=w1436:i32)  [unwired: 1 in]
        n669 = call "Beampointing get set motor position.vi"("Active CCD"=w1436, "get or set"=enum16{"get", "set"}."get", "dev variable alias Motors X"=w1442) -> ("Actual Position"=w1443:dbl)  [unwired: 8 in]
        n670 = Index Array(array=w1462, index (row)=w1436) -> (element=w1461:dbl[])  [unwired: 1 in]
        n671 = Reverse 1D Array(array=w1461) -> (reversed array=w1460:dbl[])
        n672 = Index Array(array=w1460) -> (element=w1459:dbl)  [unwired: 1 in]
        n673 = Index Array(array=w1454, index=w1436) -> (element=w1463:T30)
        n674 = Unbundle By Name(w1463) -> ("Invert Direction Y"=w1447:bool, "enable feedback"=w1457:bool)  [unwired: 1 out]
        n675 = Greater Or Equal To 0?(x=w1459) -> (x >= 0?=w1458:bool)
        n676 = Unbundle By Name(w1439) -> ("steps speed X"=w1451:dbl[], "steps speed Y"=w1450:dbl[])
        n677 = Index Array(array=w1450, index=w1436) -> (element=w1448:dbl)
        n678 = Index Array(array=w1451, index=w1436) -> (element=w1449:dbl)
        n679 = Select(t=w1449, s=w1447, f=w1448) -> (s? t:f=w1446:dbl)
        n680 = case shown="False" w1457 {
          tunnel: w1458 -> [_ w1487]
          tunnel: w1446 -> [_ w1486]
          tunnel: w1447 -> [_ w1485]
          tunnel: w1443 -> [w1478 w1484]
          tunnel: w1442 -> [_ w1481]
          tunnel: w1436 -> [_ w1480]
          tunnel: [w1478 w1479] -> w1437
          frame False {
          }
          frame True {
            n681 = case shown="False" w1487 {
              tunnel: w1485 -> [w1491 w1501]
              tunnel: w1486 -> [w1490 w1500]
              tunnel: w1484 -> [w1489 w1499]
              tunnel: [w1488 w1498] -> w1483
              frame True {
                n682 = case shown="False" w1491 {
                  tunnel: w1489 -> [w1494 w1497]
                  tunnel: w1490 -> [w1493 w1496]
                  tunnel: [w1492 w1495] -> w1488
                  frame False {
                    n683 = Add(x=w1494, y=w1493) -> (x+y=w1492:dbl)
                  }
                  frame True {
                    n684 = Subtract(x=w1497, y=w1496) -> (x-y=w1495:dbl)
                  }
                }
              }
              frame False {
                n685 = case shown="False" w1501 {
                  tunnel: w1499 -> [w1504 w1507]
                  tunnel: w1500 -> [w1503 w1506]
                  tunnel: [w1502 w1505] -> w1498
                  frame False {
                    n686 = Subtract(x=w1504, y=w1503) -> (x-y=w1502:dbl)
                  }
                  frame True {
                    n687 = Add(x=w1507, y=w1506) -> (x+y=w1505:dbl)
                  }
                }
              }
            }
            n688 = call "Beampointing get set motor position.vi"("Active CCD"=w1480, "Set position"=w1483, "get or set"=enum16{"get", "set"}."set", "dev variable alias Motors X"=w1481) -> ("Actual Position"=w1479:dbl)  [unwired: 7 in]
          }
        }
        n689 = call <vilib>:"Build State String with Arguments__jki_lib_state_machine.vi"("Arguments (\"\")"=w1452, "State"="Wait" ("State(s) in Front (\"\")")) -> ()  [unwired: 4 in, 1 out]
        n690 = Unbundle By Name(w1439) -> ("Motor positions.Positions y"=w1441:dbl[])
        n691 = call <vilib>:"Add State(s) to Queue__jki_lib_state_machine.vi"("State(s) in (\"\")"=w1467) -> ("States Out"=w1466:string)  [unwired: 14 in]
        n692 = Replace Array Subset(array=w1441, new element=w1437, index=w1436) -> (w1440:dbl[])
        n693 = Bundle By Name(cluster=w1439, "Motor positions.Positions y"=w1440) -> (w1438:T31)
        "Moving Y" <- w1452
      }
      frame "Wait" {
        # "Your code here.\n(You can make a copy of, or modify, this frame)"
        n694 = disable-structure shown="Disabled" {
          disable-tunnel: w1513 -> [w1527 _]
          disable-tunnel: w1512 -> [w1526 _]
          disable-tunnel: w1511 -> [w1525 _]
          disable-tunnel: w1510 -> [w1523 w1547]
          disable-tunnel: [w1522 w1547] -> w1509
          frame Disabled {
            n695 = call-poly <userlib>:"Filter 1D Array__ogtk.vi"("items to filter"=w1525, "array"=w1526) -> ("filtered item indices"=w1524:i32[])  [unwired: 4 in, 1 out]
            n696 = Index Array(array=w1524) -> (element=w1521:i32)  [unwired: 1 in]
            n697 = flat-sequence {
              tunnel: T27."Disabled and Grayed Out" ("Disabled") -> [w1528]
              tunnel: w1523 -> [w1536]
              tunnel: [w1535] -> w1522
              tunnel: w1521 -> [w1534]
              tunnel: w1520 -> [w1533]
              tunnel: T27."Enabled" ("Disabled") -> [w1546]
              frame #0 {
                n698 = property on="Right" class="Bool (strict)"("DisabledEnum"=w1528) -> ()  [unwired: 2 in, 2 out]
                n699 = property on="Up" class="Bool (strict)"("DisabledEnum"=w1528) -> ()  [unwired: 2 in, 2 out]
                n700 = property on="Left" class="Bool (strict)"("DisabledEnum"=w1528) -> ()  [unwired: 2 in, 2 out]
                n701 = property on="Down" class="Bool (strict)"("DisabledEnum"=w1528) -> ()  [unwired: 2 in, 2 out]
                n702 = property on="StepSize" class="DigNum (strict)"("DisabledEnum"=w1528) -> ()  [unwired: 2 in, 2 out]
              }
              frame #1 {
                n703 = Wait (ms)(milliseconds to wait=u32 1500) -> ()  [unwired: 1 out]
              }
              frame #2 {
                n704 = property on="Moving Y" class="Str"("Value"="") -> ()  [unwired: 2 in, 2 out]
                n705 = property on="Moving X" class="Str"("Value"="") -> ()  [unwired: 2 in, 2 out]
              }
              frame #3 {
                n706 = Equal?(x=w1533, y=w1534) -> (x = y?=w1532:bool)
                n707 = case shown="True" w1532 {
                  tunnel: _ -> [_ w1543]
                  tunnel: w1536 -> [w1537 w1540]
                  tunnel: [w1537 w1538] -> w1535
                  frame False {
                  }
                  frame True {
                    n708 = Unbundle By Name(w1543) -> ("Ref X"=w1542, "Ref Y"=w1541)
                    n709 = property class="DigNum (strict)"(reference=w1542, error in=w1540) -> (error out=w1539:errorcluster, "Value"=w1545:dbl)  [unwired: 1 out]
                    n710 = property class="DigNum (strict)"(reference=w1541, error in=w1539) -> (error out=w1538:errorcluster, "Value"=w1544:dbl)  [unwired: 1 out]
                    n711 = property on="Position 1" class="DigNum (strict)"("Value"=w1545) -> ()  [unwired: 2 in, 2 out]
                    n712 = property on="Position 2" class="DigNum (strict)"("Value"=w1544) -> ()  [unwired: 2 in, 2 out]
                  }
                }
              }
              frame #4 {
                n713 = property on="Right" class="Bool (strict)"("DisabledEnum"=w1546) -> ()  [unwired: 2 in, 2 out]
                n714 = property on="Up" class="Bool (strict)"("DisabledEnum"=w1546) -> ()  [unwired: 2 in, 2 out]
                n715 = property on="Left" class="Bool (strict)"("DisabledEnum"=w1546) -> ()  [unwired: 2 in, 2 out]
                n716 = property on="Down" class="Bool (strict)"("DisabledEnum"=w1546) -> ()  [unwired: 2 in, 2 out]
                n717 = property on="StepSize" class="DigNum (strict)"("DisabledEnum"=w1546) -> ()  [unwired: 2 in, 2 out]
              }
            }
            n718 = Unbundle By Name(w1527) -> ("active ccd"=w1520:i32)
          }
          frame Enabled {
          }
        }
        n719 = call <vilib>:"Add State(s) to Queue__jki_lib_state_machine.vi"("State(s) in (\"\")"=w1517) -> ("States Out"=w1516:string)  [unwired: 14 in]
        n720 = local read "Mean Centroid X"() -> (w1514:dbl[][])
        n721 = Bundle By Name(cluster=w1513, "Mean Centroid X"=w1514, "Mean Centroid Y"=w1514) -> (w1515:T31)
      }
      frame "---------------Statistics--------------" {
        # "Template Separator\n(You can make a copy of, or modify, this frame)"
        n722 = call <vilib>:"Add State(s) to Queue__jki_lib_state_machine.vi"("State(s) in (\"\")"=w1552) -> ("States Out"=w1551:string)  [unwired: 14 in]
      }
      frame "Save Stats" {
        # "Your code here.\n(You can make a copy of, or modify, this frame)"
        n723 = property on="CCD 1" class="XYGraph (strict)"() -> ("Value"=w1564:cluster{timestamp[], dbl[]}[])  [unwired: 2 in, 2 out]
        n724 = property on="CCD 2" class="XYGraph (strict)"() -> ("Value"=w1563:cluster{timestamp[], dbl[]}[])  [unwired: 2 in, 2 out]
        n725 = property on="CCD 3" class="XYGraph (strict)"() -> ("Value"=w1562:cluster{timestamp[], dbl[]}[])  [unwired: 2 in, 2 out]
        n726 = property on="CCD 4" class="XYGraph (strict)"() -> ("Value"=w1561:cluster{timestamp[], dbl[]}[])  [unwired: 2 in, 2 out]
        n727 = property on="CCD 5" class="XYGraph (strict)"() -> ("Value"=w1560:cluster{timestamp[], dbl[]}[])  [unwired: 2 in, 2 out]
        n728 = property on="CCD 6" class="XYGraph (strict)"() -> ("Value"=w1559:cluster{timestamp[], dbl[]}[])  [unwired: 2 in, 2 out]
        n729 = property on="CCD 7" class="XYGraph (strict)"() -> ("Value"=w1558:cluster{timestamp[], dbl[]}[])  [unwired: 2 in, 2 out]
        n730 = property on="CCD 8" class="XYGraph (strict)"() -> ("Value"=w1557:cluster{timestamp[], dbl[]}[])  [unwired: 2 in, 2 out]
        n731 = Build Array(w1564, w1563, w1562, w1561, w1560, w1559, w1558, w1557) -> (w1556:cluster{timestamp[], dbl[]}[][])
        n732 = disable-structure shown="Disabled" {
          disable-tunnel: w1568 -> [w1572 _]
          disable-tunnel: [w1571 _] -> w1567
          disable-tunnel: w1556 -> [w1570 _]
          disable-tunnel: w1555 -> [w1569 _]
          frame Disabled {
            n733 = for {
              tunnel: w1570 -> [w1575] mode=indexing
              tunnel: w1569 -> [w1574] mode=indexing
              n734 = Empty String/Path?(string/path=w1574) -> (empty?=w1573:bool)
              n735 = case shown="False" w1573 {
                tunnel: w1575 -> [w1581 _]
                tunnel: w1574 -> [w1579 _]
                frame False {
                  n736 = Index Array(array=w1581, index #1=0 ("index"), index #2=1 ("index"), index #3=2 ("index"), index #4=3 ("index")) -> (element #1=w1616:cluster{timestamp[], dbl[]}, element #2=w1610:cluster{timestamp[], dbl[]}, element #3=w1609:cluster{timestamp[], dbl[]}, element #4=w1608:cluster{timestamp[], dbl[]})  [unwired: 1 in, 1 out]
                  n737 = Concatenate Strings(w1579, ".dat" ("string")) -> (w1577:string)
                  n738 = Unbundle(w1616) -> (w1615:timestamp[], w1593:dbl[])
                  n739 = Unbundle(w1610) -> (w1584:dbl[])  [unwired: 1 out]
                  n740 = Unbundle(w1609) -> (w1583:dbl[])  [unwired: 1 out]
                  n741 = Unbundle(w1608) -> (w1582:dbl[])  [unwired: 1 out]
                  n742 = Build Path(base path="save path", name or relative path=w1577) -> (appended path=w1576:path)
                  n743 = for {
                    tunnel: w1615 -> [w1618] mode=indexing
                    tunnel: [w1617] -> w1591 mode=indexing
                    n744 = Format Date/Time String(time format string (%c)="%Y%m%d%H%M%S", seconds (now)=w1618) -> (date/time string=w1617:string)  [unwired: 1 in]
                  }
                  n745 = Array Size(array=w1593) -> (size(s)=w1594:i32)
                  n746 = Number To Fractional String(number=w1593) -> (F-format string=w1590:string[])  [unwired: 3 in]
                  n747 = Number To Fractional String(number=w1584) -> (F-format string=w1587:string[])  [unwired: 3 in]
                  n748 = Number To Fractional String(number=w1583) -> (F-format string=w1586:string[])  [unwired: 3 in]
                  n749 = Number To Fractional String(number=w1582) -> (F-format string=w1585:string[])  [unwired: 3 in]
                  n750 = Initialize Array("", w1594, 5 ("dimension size")) -> (w1592:string[][])
                  n751 = Insert Into Array(array=w1592, index (col)=0 ("disabled index (col)"), new element=w1591) -> (w1602:string[][])  [unwired: 1 in]
                  n752 = Insert Into Array(array=w1602, index (col)=1 ("disabled index (col)"), new element=w1590) -> (w1601:string[][])  [unwired: 1 in]
                  n753 = Insert Into Array(array=w1601, index (col)=2 ("disabled index (col)"), new element=w1587) -> (w1605:string[][])  [unwired: 1 in]
                  n754 = Insert Into Array(array=w1605, index (col)=3 ("disabled index (col)"), new element=w1586) -> (w1606:string[][])  [unwired: 1 in]
                  n755 = Insert Into Array(array=w1606, index (col)=4 ("disabled index (col)"), new element=w1585) -> (w1607:string[][])  [unwired: 1 in]
                  n756 = Insert Into Array(array=w1607, index (row)=0, new element=string[] ["time", "Centroid X", "Centroid Y", "Motor Axis 1", "Motor Axis 2"] ("new element/subarray 2")) -> (w1589:string[][])  [unwired: 1 in]
                  n757 = call-poly <vilib>:"Write To Spreadsheet File.vi"("2D data"=w1589, "file path (dialog if empty)"=w1576) -> ()  [unwired: 6 in, 1 out]
                }
                frame True {
                }
              }
            }
            n758 = call <vilib>:"Add State(s) to Queue__jki_lib_state_machine.vi"("State(s) in (\"\")"=w1572) -> ("States Out"=w1571:string)  [unwired: 14 in]
          }
          frame Enabled {
          }
        }
        n759 = property on="Save Stats" class="Bool (strict)"("Value"=FALSE ("Save Stats")) -> ()  [unwired: 2 in, 2 out]
      }
      frame "tdms" {
        w1633 = 21600.0 ("new tdms")
        # "Your code here.\n(You can make a copy of, or modify, this frame)"
        n760 = Unbundle By Name(w1640) -> ("active cams"=w1626:string[], "tdms ref"=w1623:refnum<k34>, "Offset X"=w1639:dbl[][], "Offset Y"=w1638:dbl[][], "Motor positions.Positions x"=w1621:dbl[], "Motor positions.Positions y"=w1620:dbl[])
        n761 = for {
          tunnel: w1639 -> [w1683]
          tunnel: w1638 -> [w1682]
          tunnel: w1626 -> [w1655] mode=indexing
          tunnel: w1623 -> [w1656]
          tunnel: w1642 -> [w1650]
          tunnel: [w1659] -> w1641
          tunnel: w1621 -> [w1649]
          tunnel: w1620 -> [w1647]
          i -> [w1646]
          n762 = Index Array(array=w1683, index (row)=w1646) -> (element=w1681:dbl[])  [unwired: 1 in]
          n763 = Index Array(array=w1682, index (row)=w1646) -> (element=w1680:dbl[])  [unwired: 1 in]
          n764 = Reverse 1D Array(array=w1680) -> (reversed array=w1678:dbl[])
          n765 = Reverse 1D Array(array=w1681) -> (reversed array=w1679:dbl[])
          n766 = Index Array(array=w1679) -> (element=w1677:dbl)  [unwired: 1 in]
          n767 = Index Array(array=w1678) -> (element=w1676:dbl)  [unwired: 1 in]
          n768 = Index Array(array=w1647, index=w1646) -> (element=w1645:dbl)
          n769 = Index Array(array=w1649, index=w1646) -> (element=w1648:dbl)
          n770 = Build Array(w1677) -> (w1658:dbl[])
          n771 = Build Array(w1676) -> (w1671:dbl[])
          n772 = Get Date/Time In Seconds() -> (seconds since 1Jan1904=w1657:timestamp)
          n773 = Build Array(w1657) -> (w1653:timestamp[])
          n774 = Build Array(w1648) -> (w1665:dbl[])
          n775 = TDMS Write(0:w1656, 5:w1655, 7:"time", 9:w1653, 11:w1650) -> (4:w1652:refnum<k34>, 15:w1651:errorcluster)  [unwired: 1 in, 2 out]
          n776 = Build Array(w1645) -> (w1660:dbl[])
          n777 = TDMS Write(0:w1652, 5:w1655, 7:"centroid X", 9:w1658, 11:w1651) -> (4:w1674:refnum<k34>, 6:w1673:string, 15:w1672:errorcluster)  [unwired: 1 in, 1 out]
          n778 = TDMS Write(0:w1674, 5:w1673, 7:"centroid Y", 9:w1671, 11:w1672) -> (4:w1668:refnum<k34>, 6:w1667:string, 15:w1669:errorcluster)  [unwired: 1 in, 1 out]
          n779 = TDMS Write(0:w1668, 5:w1667, 7:"Motor Axis 1", 9:w1665, 11:w1669) -> (4:w1664:refnum<k34>, 6:w1663:string, 15:w1661:errorcluster)  [unwired: 1 in, 1 out]
          n780 = TDMS Write(0:w1664, 5:w1663, 7:"Motor Axis 2", 9:w1660, 11:w1661) -> (15:w1659:errorcluster)  [unwired: 1 in, 3 out]
        }
        n781 = property on="millisecond timer value" class="DigNum (strict)"() -> ("Value"=w1625:u32)  [unwired: 2 in, 2 out]
        n782 = Tick Count (ms)() -> (millisecond timer value=w1624:u32)
        n783 = Unbundle By Name(w1640) -> ()  [unwired: 1 out]
        n784 = Subtract(x=w1624, y=w1625) -> (x-y=w1628:u32)
        n785 = Divide(x=w1628, y=u32 1000) -> (x/y=w1630:dbl)
        n786 = Quotient & Remainder(x=w1630, y=w1633) -> (x-y*floor(x/y)=w1631:dbl)  [unwired: 1 out]
        n787 = Subtract(x=w1633, y=20.0) -> (x-y=w1635:dbl)
        n788 = Greater?(x=w1631, y=w1635) -> (0:w1632:bool)
        n789 = Select(t="newtdms", s=w1632, f="") -> (s? t:f=w1627:string)
        n790 = call <vilib>:"Add State(s) to Queue__jki_lib_state_machine.vi"("State(s) in (\"\")"=w1644, "State(s) at Back (\"\")"=w1627) -> ("States Out"=w1643:string)  [unwired: 13 in]
      }
      frame "Reset History" {
        # "Your code here.\n(You can make a copy of, or modify, this frame)"
        n791 = for {
          N: 1 -> [_]
          shift-right: [w1694] -> w1686
          shift-left: timestamp[][] [] ("Time") -> [w1696]
          n792 = for {
            N: 12 -> [_]
            tunnel: w1696 -> [w1699] mode=indexing
            tunnel: [w1697] -> w1694 mode=indexing
            n793 = Get Date/Time In Seconds() -> (seconds since 1Jan1904=w1698:timestamp)
            n794 = Build Array (concatenate)(w1699, w1698) -> (w1697:timestamp[])
          }
        }
        n795 = local read "Offset X"() -> (w1685:dbl[][])
        n796 = Bundle By Name(cluster=w1690, "Offset X"=w1685, "Offset Y"=w1685, "Time"=w1686, "Motor X"=w1685) -> (w1689:T31)
        n797 = call <vilib>:"Add State(s) to Queue__jki_lib_state_machine.vi"("State(s) in (\"\")"=w1693) -> ("States Out"=w1692:string)  [unwired: 14 in]
      }
      frame "New Category: 2" {
        # "Your code here.\n(You can make a copy of, or modify, this frame)"
        n798 = call <vilib>:"Add State(s) to Queue__jki_lib_state_machine.vi"("State(s) in (\"\")"=w1704) -> ("States Out"=w1703:string)  [unwired: 14 in]
      }
      frame "stats" {
        # "Your code here.\n(You can make a copy of, or modify, this frame)"
        n799 = Unbundle By Name(w1720) -> ("Offset X"=w1711:dbl[][], "Offset Y"=w1710:dbl[][], "Time"=w1709:timestamp[][], "Motor X"=w1708:dbl[][], "Motor Y"=w1707:dbl[][], "tdms ref"=w1715:refnum<k34>)
        n800 = TDMS List Contents(4:w1714, 7:w1715) -> (0:w1706:errorcluster, 2:w1718:string[], 3:w1717:refnum<k34>)  [unwired: 1 in, 1 out]
        n801 = call <vilib>:"ClearError.vi"("error in (no error)"=w1706) -> ("error out"=w1716:errorcluster)
        n802 = for {
          tunnel: w1716 -> [w1787]
          tunnel: [w1773] -> w1712 mode=indexing
          tunnel: [w1772] -> w1713
          tunnel: [w1771] -> _
          tunnel: w1717 -> [w1770]
          tunnel: w1718 -> [w1769] mode=indexing
          w1788 = dbl[] [] ("appended array")
          n803 = TDMS Read(0:w1770, 5:w1769, 7:"time", 11:w1787, 12:timestamp[] [] ("appended array")) -> (4:w1802:refnum<k34>, 6:w1798:string, 10:w1779:timestamp[], 15:w1786:errorcluster)  [unwired: 3 in, 2 out]
          n804 = TDMS Read(0:w1802, 5:w1798, 7:"centroid X", 11:w1786, 12:w1788) -> (4:w1801:refnum<k34>, 6:w1797:string, 10:w1782:dbl[], 15:w1785:errorcluster)  [unwired: 3 in, 2 out]
          n805 = TDMS Read(0:w1801, 5:w1797, 7:"centroid Y", 11:w1785, 12:w1788) -> (4:w1800:refnum<k34>, 6:w1796:string, 10:w1781:dbl[], 15:w1784:errorcluster)  [unwired: 3 in, 2 out]
          n806 = TDMS Read(0:w1800, 5:w1796, 7:"Motor Axis 1", 11:w1784, 12:w1788) -> (4:w1799:refnum<k34>, 6:w1795:string, 10:w1780:dbl[], 15:w1783:errorcluster)  [unwired: 3 in, 2 out]
          n807 = TDMS Read(0:w1799, 5:w1795, 7:"Motor Axis 2", 11:w1783, 12:w1788) -> (4:w1771:refnum<k34>, 10:w1778:dbl[], 15:w1772:errorcluster)  [unwired: 3 in, 3 out]
          n808 = Bundle("appended array"=w1779, "appended array"=w1782) -> (w1777:T40)  [unwired: 1 in]
          n809 = Bundle("appended array"=w1779, "appended array"=w1781) -> (w1776:T40)  [unwired: 1 in]
          n810 = Bundle("appended array"=w1779, "appended array"=w1780) -> (w1775:T40)  [unwired: 1 in]
          n811 = Bundle("appended array"=w1779, "appended array"=w1778) -> (w1774:T40)  [unwired: 1 in]
          n812 = Build Array(w1777, w1776, w1775, w1774) -> (w1773:T41)
        }
        n813 = disable-structure shown="Disabled" {
          disable-tunnel: w1719 -> [w1752 _]
          disable-tunnel: w1711 -> [w1751 _]
          disable-tunnel: w1710 -> [w1750 _]
          disable-tunnel: w1709 -> [w1749 _]
          disable-tunnel: w1708 -> [w1748 _]
          disable-tunnel: w1707 -> [w1747 _]
          frame Disabled {
            n814 = for {
              tunnel: w1752 -> [_] mode=indexing
              tunnel: w1751 -> [w1762]
              tunnel: w1750 -> [w1761]
              tunnel: w1749 -> [w1760]
              tunnel: w1748 -> [w1756]
              tunnel: w1747 -> [w1755]
              tunnel: [w1764] -> _ mode=indexing
              i -> [w1763]
              n815 = Index Array(array=w1761, index (row)=w1763) -> (element=w1757:dbl[])  [unwired: 1 in]
              n816 = Index Array(array=w1756, index (row)=w1763) -> (element=w1754:dbl[])  [unwired: 1 in]
              n817 = Index Array(array=w1755, index (row)=w1763) -> (element=w1753:dbl[])  [unwired: 1 in]
              n818 = Index Array(array=w1762, index (row)=w1763) -> (element=w1758:dbl[])  [unwired: 1 in]
              n819 = Index Array(array=w1760, index (row)=w1763) -> (element=w1759:timestamp[])  [unwired: 1 in]
              n820 = Bundle("Time"=w1759, "Motor X"=w1754) -> (w1767:cluster{"Time":timestamp[], "Motor X":dbl[]})  [unwired: 1 in]
              n821 = Bundle("Time"=w1759, "Motor Y"=w1753) -> (w1768:cluster{"Time":timestamp[], "Motor Y":dbl[]})  [unwired: 1 in]
              n822 = Bundle("Time"=w1759, "Offset X"=w1758) -> (w1766:cluster{"Time":timestamp[], "Offset X":dbl[]})  [unwired: 1 in]
              n823 = Bundle("Time"=w1759, "Offset Y"=w1757) -> (w1765:cluster{"Time":timestamp[], "Offset Y":dbl[]})  [unwired: 1 in]
              n824 = Build Array(w1765, w1766, w1767, w1768) -> (w1764:cluster{"Time":timestamp[], "Motor Y":dbl[]}[])
            }
          }
          frame Enabled {
          }
        }
        n825 = Index Array(array=w1712, index (row) #1=0 ("index (row)"), index (row) #2=1 ("index (row)"), index (row) #3=2 ("index (row)"), index (row) #4=3 ("index (row)"), index (row) #5=4 ("index (row)"), index (row) #6=5 ("index (row)"), index (row) #7=6 ("index (row)"), index (row) #8=7 ("index (row)"), index (row) #9=8 ("index (row)"), index (row) #10=9 ("index (row)"), index (row) #11=10 ("index (row)"), index (row) #12=11 ("index (row)")) -> (element #1=→"CCD 1":T41, element #2=→"CCD 2":T41, element #3=→"CCD 3":T41, element #4=→"CCD 4":T41, element #5=→"CCD 5":T41, element #6=→"CCD 6":T41, element #7=→"CCD 7":T41, element #8=→"CCD 8":T41, element #9=→"CCD 9":T41, element #10=→"CCD 10":T41, element #11=→"CCD 11":T41, element #12=→"CCD 12":T41)  [unwired: 12 in]
        n826 = call <vilib>:"Add State(s) to Queue__jki_lib_state_machine.vi"("State(s) in (\"\")"=w1746) -> ("States Out"=w1745:string)  [unwired: 14 in]
      }
      frame "newtdms" {
        # "Your code here.\n(You can make a copy of, or modify, this frame)"
        n827 = Unbundle By Name(w1838) -> ("tdms ref"=w1831:refnum<k34>, "active cams"=w1826:string[])
        n828 = local read "config path"() -> (w1806:string)
        n829 = call-poly <userlib>:"Strip Path Extension__ogtk.vi"("path"=w1806) -> ("root"=w1805:string)  [unwired: 1 out]
        n830 = TDMS Close(8:w1836, 11:w1831) -> (0:w1825:errorcluster)  [unwired: 1 out]
        n831 = String To Path(string=w1805) -> (path=w1804:path)
        n832 = Strip Path(path=w1804) -> (name=w1803:string)  [unwired: 1 out]
        n833 = call <vilib>:"Clear Errors.vi"("error in (no error)"=w1825) -> ("error out"=w1814:errorcluster)  [unwired: 5 in, 1 out]
        n834 = Get Date/Time In Seconds() -> (seconds since 1Jan1904=w1819:timestamp)
        n835 = property on="new tdms" class="Bool (strict)"("Value"=FALSE ("new tdms")) -> ()  [unwired: 2 in, 2 out]
        n836 = Format Date/Time String(time format string (%c)="%Y%m%d", seconds (now)=w1819) -> (date/time string=w1820:string)  [unwired: 1 in]
        n837 = Format Date/Time String(time format string (%c)="%Y%m%d%H%M", seconds (now)=w1819) -> (date/time string=w1817:string)  [unwired: 1 in]
        n838 = Build Path(base path="tdms root", name or relative path=w1820) -> (appended path=w1821:path)
        n839 = Concatenate Strings(w1817, w1803, ".tdms" ("string")) -> (w1816:string)
        n840 = String To Path(string=w1816) -> (path=w1812:path)
        n841 = call <vilib>:"Check if File or Folder Exists.vi"("error in (no error)"=w1814, "path"=w1821) -> ("error out"=w1824:errorcluster, "file or folder exists?"=w1822:bool, "dup path"=w1823:path)  [unwired: 7 in]
        n842 = case shown="False" w1822 {
          tunnel: w1823 -> [w1844 w1846]
          tunnel: [w1843 w1846] -> w1811
          tunnel: w1824 -> [w1842 w1845]
          tunnel: [w1841 w1845] -> w1813
          frame False {
            n843 = Create Folder(path (use dialog)=w1844, error in=w1842) -> (created path=w1843:path, error out=w1841:errorcluster)  [unwired: 1 in, 1 out]
          }
          frame True {
          }
        }
        n844 = call <vilib>:"Add State(s) to Queue__jki_lib_state_machine.vi"("State(s) in (\"\")"=w1840) -> ("States Out"=w1839:string)  [unwired: 14 in]
        n845 = Build Path(base path=w1811, name or relative path=w1812) -> (appended path=w1832:path)
        n846 = TDMS Open(6:FALSE ("disable buffering (T)"), 7:enum16{"1.0", "2.0"}."2.0" ("file format version (2.0)"), 8:w1813, 10:T28."create or replace" ("operation"), 11:w1832) -> (0:w1829:errorcluster, 3:w1828:refnum<k34>)  [unwired: 2 in]
        n847 = call "TDMSbuffersize.vi"("error in (no error)"=w1829, "group names"=w1826, "Data Value Reference in"=w1828) -> ("error out"=w1809:errorcluster, "Data Value Reference out"=w1827:refnum<k34>)  [unwired: 7 in]
        n848 = Bundle By Name(cluster=w1838, "tdms ref"=w1827) -> (w1837:T31)
      }
      frame "Center" {
        # "Your code here.\n(You can make a copy of, or modify, this frame)"
        n849 = control-ref of="image::1"() -> (w1862:refnum<vi>)
        n850 = control-ref of="image::2"() -> (w1861:refnum<vi>)
        n851 = control-ref of="image::3"() -> (w1860:refnum<vi>)
        n852 = control-ref of="image::4"() -> (w1859:refnum<vi>)
        n853 = control-ref of="image::5"() -> (w1858:refnum<vi>)
        n854 = control-ref of="image::6"() -> (w1857:refnum<vi>)
        n855 = control-ref of="image::7"() -> (w1856:refnum<vi>)
        n856 = control-ref of="image::8"() -> (w1855:refnum<vi>)
        n857 = control-ref of="image::9"() -> (w1854:refnum<vi>)
        n858 = control-ref of="image::10"() -> (w1853:refnum<vi>)
        n859 = control-ref of="image::11"() -> (w1852:refnum<vi>)
        n860 = control-ref of="image::12"() -> (w1851:refnum<vi>)
        n861 = for {
          tunnel: [w1871] -> w1850 mode=indexing
          tunnel: w1849 -> [w1870] mode=indexing
          n862 = Unbundle By Name(w1870) -> ("Target.X::12"=w1869:refnum<vi>, "Target.Y::12"=w1868:refnum<vi>)
          n863 = property class="DigNum (strict)"(reference=w1869) -> ("Value"=w1872:dbl)  [unwired: 1 in, 2 out]
          n864 = property class="DigNum (strict)"(reference=w1868) -> ("Value"=w1873:dbl)  [unwired: 1 in, 2 out]
          n865 = Bundle("Value"=w1872, "Value"=w1873) -> (w1871:cluster{"Value":dbl, "Value":dbl})  [unwired: 1 in]
        }
        n866 = call <vilib>:"Add State(s) to Queue__jki_lib_state_machine.vi"("State(s) in (\"\")"=w1867) -> ("States Out"=w1866:string)  [unwired: 14 in]
        n867 = Build Array(w1862, w1861, w1860, w1859, w1858, w1857, w1856, w1855, w1854, w1853, w1852, w1851) -> (w1863:refnum<vi>[])
        n868 = for {
          tunnel: w1863 -> [w1875] mode=indexing
          tunnel: w1850 -> [w1874] mode=indexing
          n869 = property class="ImageControl"(reference=w1875, "Image Center Position"=w1874) -> ()  [unwired: 1 in, 2 out]
        }
        n870 = property on="Center" class="Bool (strict)"("Value"=FALSE ("Center")) -> ()  [unwired: 2 in, 2 out]
      }
      frame "ImgToAvg" {
        n871 = Decimal String To Number(string=w1886) -> (number=w1883:i32)  [unwired: 2 in, 1 out]
        n872 = Bundle By Name(cluster=w1885, "img to avg"=w1883) -> (w1884:T31)
        n873 = call <vilib>:"Build State String with Arguments__jki_lib_state_machine.vi"("Arguments (\"\")"="T" ("Arguments (\"\")"), "State"=" Device Ini") -> ("State with Arguments"=w1877:string)  [unwired: 4 in]
        n874 = call <vilib>:"Add State(s) to Queue__jki_lib_state_machine.vi"("State(s) in Front (\"\")"=w1877, "State(s) in (\"\")"=w1882) -> ("States Out"=w1881:string)  [unwired: 13 in]
      }
      frame "history" {
        # "Your code here.\n(You can make a copy of, or modify, this frame)"
        n875 = Unbundle By Name(w1897) -> ("Offset X"=w1903:dbl[][], "Offset Y"=w1902:dbl[][], "Mean Centroid X"=w1901:dbl[][], "Mean Centroid Y"=w1900:dbl[][], "Motor X"=w1899:dbl[][], "Motor Y"=w1898:dbl[][], "Time"=w1889:timestamp[][])
        n876 = for {
          tunnel: w1903 -> [w1921] mode=indexing
          tunnel: w1902 -> [w1919] mode=indexing
          tunnel: w1901 -> [w1918] mode=indexing
          tunnel: w1900 -> [w1917] mode=indexing
          tunnel: w1899 -> [w1916] mode=indexing
          tunnel: w1898 -> [w1915] mode=indexing
          tunnel: [w1920] -> w1895 mode=indexing
          tunnel: [w1914] -> w1894 mode=indexing
          tunnel: [w1910] -> w1893 mode=indexing
          tunnel: [w1913] -> w1892 mode=indexing
          tunnel: [w1912] -> w1891 mode=indexing
          tunnel: [w1911] -> w1890 mode=indexing
          tunnel: w1889 -> [w1909] mode=indexing
          tunnel: [w1907] -> w1888 mode=indexing
          w1908 = 0
          n877 = Delete From Array(array=w1916, index=w1908) -> (array with subset deleted=w1912:dbl[])  [unwired: 1 in, 1 out]
          n878 = Delete From Array(array=w1915, index=w1908) -> (array with subset deleted=w1911:dbl[])  [unwired: 1 in, 1 out]
          n879 = Delete From Array(array=w1909, index=w1908) -> (array with subset deleted=w1907:timestamp[])  [unwired: 1 in, 1 out]
          n880 = Delete From Array(array=w1918, index=w1908) -> (array with subset deleted=w1910:dbl[])  [unwired: 1 in, 1 out]
          n881 = Delete From Array(array=w1917, index=w1908) -> (array with subset deleted=w1913:dbl[])  [unwired: 1 in, 1 out]
          n882 = Delete From Array(array=w1919, index=w1908) -> (array with subset deleted=w1914:dbl[])  [unwired: 1 in, 1 out]
          n883 = Delete From Array(array=w1921, index=w1908) -> (array with subset deleted=w1920:dbl[])  [unwired: 1 in, 1 out]
        }
        n884 = call <vilib>:"Add State(s) to Queue__jki_lib_state_machine.vi"("State(s) in (\"\")"=w1906) -> ("States Out"=w1905:string)  [unwired: 14 in]
        n885 = Bundle By Name(cluster=w1897, "Offset X"=w1895, "Offset Y"=w1894, "Mean Centroid X"=w1893, "Mean Centroid Y"=w1892, "Motor X"=w1891, "Motor Y"=w1890, "Time"=w1888) -> (w1896:T31)
      }
    }
    "Prev State" <- w49
    n886 = property on="Box" class="Arr (strict)"() -> ("Value"=w57:T3)  [unwired: 2 in, 2 out]
    n887 = for {
      tunnel: w58 -> [w101]
      tunnel: w51 -> [w110]
      tunnel: w55 -> [w108] mode=indexing
      tunnel: w57 -> [w69] mode=indexing
      tunnel: w54 -> [w99]
      tunnel: w53 -> [w98]
      tunnel: w52 -> [w80]
      i -> [w79]
      w94 = T42 {"Draw"=TRUE, "Target"={"x"=20.0, "y"=20.0}, "Size"={"x"=20.0, "y"=20.0}, "Angle"=1250067.0, "Color"=1250067, "Thickness"=0, "CrosshairLabel"=""} ("Crosshair")
      w88 = T43 {"Left"=0, "Top"=0, "Right"=0, "Bottom"=0} ("Bounding Rectangle")
      n888 = call-poly <userlib>:"Filter 1D Array__ogtk.vi"("items to filter"=w108, "array"=w110) -> ("filtered item indices"=w111:i32[])  [unwired: 4 in, 1 out]
      n889 = Index Array(array=w111) -> (element=w100:i32)  [unwired: 1 in]
      n890 = Index Array(array=w80, index (row)=w79) -> (element=w77:dbl[])  [unwired: 1 in]
      n891 = Index Array(array=w99, index (row)=w79) -> (element=w87:dbl[])  [unwired: 1 in]
      n892 = Index Array(array=w98, index (row)=w79) -> (element=w85:dbl[])  [unwired: 1 in]
      n893 = Index Array(array=w101, index=w100) -> (element=w109:T18)
      n894 = Reverse 1D Array(array=w77) -> (reversed array=w76:dbl[])
      n895 = Unbundle By Name(w109) -> ("Target.X::12"=w113:refnum<vi>, "Target.Y::12"=w112:refnum<vi>)
      n896 = Reverse 1D Array(array=w87) -> (reversed array=w86:dbl[])
      n897 = Reverse 1D Array(array=w85) -> (reversed array=w84:dbl[])
      n898 = Index Array(array=w76) -> (element=w74:dbl)  [unwired: 1 in]
      n899 = Square Root(x=w74) -> (sqrt(x)=w73:dbl)
      n900 = Index Array(array=w84) -> (element=w81:dbl)  [unwired: 1 in]
      n901 = Index Array(array=w86) -> (element=w82:dbl)  [unwired: 1 in]
      n902 = Divide(x=w73, y=2.0) -> (x/y=w71:dbl)
      n903 = property class="DigNum (strict)"(reference=w113) -> ("Value"=w105:dbl)  [unwired: 1 in, 2 out]
      n904 = property class="DigNum (strict)"(reference=w112) -> ("Value"=w104:dbl)  [unwired: 1 in, 2 out]
      n905 = Bundle(cluster=cluster{"xhair size":dbl, "xhair size 2":dbl} {"xhair size"=25.0, "xhair size 2"=25.0} ("size"), "xhair size"=w71, "xhair size 2"=w71) -> (w75:cluster{"xhair size":dbl, "xhair size 2":dbl})
      n906 = Bundle By Name(cluster=w94, "Draw"=TRUE, "Target.x"=w105, "Target.y"=w104, "Size"=w75, "Color"=u32 16774656, "Angle"=0.0, "Thickness"=u8 1) -> (w107:T42)
      n907 = call "draw crosshair imaq.vi"("clear overlay"=TRUE, "Crosshair"=w107, "Bounding Rectangle"=w88, "image in"=w108) -> ("error out"=w91:errorcluster, "image out"=w90:T5)  [unwired: 6 in]
      n908 = Bundle By Name(cluster=w94, "Draw"=TRUE, "Target.x"=w82, "Target.y"=w81, "Size"=w75, "Color"=u32 8322834, "Angle"=0.0, "Thickness"=u8 1) -> (w92:T42)
      n909 = case shown="True" "average centroid" {
        tunnel: w92 -> [_ w118]
        tunnel: w91 -> [_ w123]
        tunnel: w90 -> [w115 w122]
        tunnel: w88 -> [_ w121]
        tunnel: w69 -> [w116 _]
        tunnel: [w114 w120] -> w68
        frame False {
          n910 = call "draw box imaq.vi"("Color"=u32 1244928, "Rectangle"=w116, "image in"=w115) -> ("error out"=w114:errorcluster)  [unwired: 7 in, 1 out]
        }
        frame True {
          n911 = call "draw crosshair imaq.vi"("clear overlay"=FALSE, "error in (no error)"=w123, "Crosshair"=w118, "Bounding Rectangle"=w121, "image in"=w122) -> ("error out"=w120:errorcluster)  [unwired: 5 in, 1 out]
        }
      }
      "error out 3" <- w68
    }
  }
  n912 = call <userlib>:"Fit VI window to Largest Dec__ogtk.vi"() -> ()  [unwired: 6 in, 2 out]
  n913 = disable-structure shown="Disabled" {
    frame Disabled {
      # "GetMotorPositions"
      # "get all motor positions"
      n914 = call <userlib>:"Tick Count (ms)__ogtk.vi"() -> ("millisecond timer value"=w1930:u32)  [unwired: 10 in, 1 out]
      n915 = Unbundle By Name(w1931) -> ("dev var alias arrays"=w1923)
      n916 = Unbundle By Name(w1923) -> ("dev variable alias Motors X"=w1922, "dev variable alias Motors Y"=w1926)
      n917 = for {
        tunnel: w1926 -> [w1939]
        tunnel: w1922 -> [w1938]
        tunnel: [w1934] -> w1924 mode=indexing
        tunnel: [w1933] -> w1925 mode=indexing
        tunnel: w1926 -> [_]
        tunnel: [errorcluster {"status"=FALSE, "code"=0, "source"=""} ("error out")] -> w1927
        i -> [w1935]
        n918 = call "Beampointing get set motor position.vi"("Active CCD"=w1935, "get or set"=enum16{"get", "set"}."get", "dev variable alias Motors X"=w1938) -> ("Actual Position"=w1934:dbl)  [unwired: 8 in]
        n919 = call "Beampointing get set motor position.vi"("Active CCD"=w1935, "get or set"=enum16{"get", "set"}."get", "dev variable alias Motors X"=w1939) -> ("Actual Position"=w1933:dbl)  [unwired: 8 in]
      }
      n920 = Bundle By Name("Positions x"=w1924, "Positions y"=w1925) -> (w1931:cluster{})  [unwired: 1 out]
      n921 = call <userlib>:"Tick Count (ms)__ogtk.vi"("error in (no error)"=w1927) -> ("millisecond timer value"=w1928:u32)  [unwired: 9 in, 1 out]
      n922 = Subtract(x=w1928, y=w1930) -> (x-y=→"get pos time":u32)
    }
    frame Enabled {
    }
  }
  n923 = Unbundle By Name(w17) -> ("tdms ref"=w16:refnum<k34>)
  n924 = for {
    tunnel: w45 -> [w1942] mode=indexing
    tunnel: w44 -> [w1941]
    tunnel: [w1940] -> w15
    n925 = call "IMAQ Dispose"("Image"=w1942, "error in (no error)"=w1941) -> ("error out"=w1940:errorcluster)  [unwired: 4 in]
  }
  n926 = TDMS Close(8:w15, 11:w16) -> (0:→"error out 2":errorcluster)  [unwired: 1 out]
